vi "BeampointingPerpsectiveDelete.vi"() -> ()   [LabVIEW 2020]
uses:
  Ctrs/beam detection.ctl
  GUI_Beampointing_single_TRA/Ctrs/move.ctl
  Shared/GUI_Template/GUI_master/tcp_new_data_event.ctl
  Shared/GUI_Template/GUI_master/tcp new data cluster.ctl
  Ctrs/thresholds.ctl
  Ctrs/Detection all.ctl
  Ctrs/BP configuration.ctl
  General GUIs/Device GUIs/GUI_Cameras/Controls/Crosshair type def.ctl
  <userlib>/_OpenG.lib/array/array.llb/Filter 1D Array with Scalar (String)__ogtk.vi
  <userlib>/_OpenG.lib/array/array.llb/Sort 1D Array (DBL)__ogtk.vi
  <userlib>/_OpenG.lib/array/array.llb/Reorder 1D Array2 (Variant)__ogtk.vi
  <userlib>/_OpenG.lib/file/file.llb/File Exists - Scalar__ogtk.vi
  <userlib>/_OpenG.lib/array/array.llb/Remove Duplicates from 1D Array (String)__ogtk.vi
  <userlib>/_OpenG.lib/file/file.llb/Strip Path Extension - String__ogtk.vi
  <vilib>/Analysis/NI_AALBase.lvlib
  <vilib>/vision/NI_Vision_Development_Module.lvlib
  <vilib>/Utility/file.llb/Write To Spreadsheet File (string).vi
panel:
  out "Image Dst Out":T1(plugin-control)
  out "12camsproc":string[](array[string])
  out "image::1":T1(plugin-control) caption="CAM-2BL-M4A"
  out "image::2":T1(plugin-control) caption="CAM-2BL-F3M5"
  out "image::3":T1(plugin-control) caption="CAM-2BL-F3M7"
  out "image::4":T1(plugin-control)
  out "image::5":T1(plugin-control)
  out "image::6":T1(plugin-control)
  out "image::7":T1(plugin-control)
  out "image::8":T1(plugin-control)
  out "image::9":T1(plugin-control)
  out "image::10":T1(plugin-control)
  out "image::11":T1(plugin-control)
  out "image::12":T1(plugin-control)
  in  "pixel calib":dbl
  out "A2y":dbl
  out "A1y":dbl
  out "A2x":dbl
  out "A1x":dbl
  in  "y'":dbl
  in  "x'":dbl
  in  "y":dbl
  in  "x":dbl
  in  "distance to target plane":dbl
  in  "seperation":dbl
  in  "downstream mirror":dbl
  in  "upstream mirror":dbl
  in  "Coupled Mirror Move":bool
  out "error out":errorcluster
  in  "active CCDs":i32(listbox)
  out "Prev State":string
  out "tcp data event 2":T2
  out "error out 3":errorcluster
  out "cam means":sgl[](array[numeric])
  in  "save path":path=path "W:/BP_DATA"
  out "millisecond timer value":u32
  out "motor refs 3":refnum<vi>[](array[refnum])
  in  "active man refs":cluster{"Ref X":refnum<vi>, "Ref Y":refnum<vi>}
  in  "#imgs avd so far":dbl
  out "Current State":string
  out "CCDs":string[](array[string])
  in  "GUIdevice 12":string
  in  "GUIdevice 11":string
  in  "GUIdevice 10":string
  in  "GUIdevice 9":string
  out "error out 2":errorcluster
  out "Names":string[](array[string])
  out "Box":T3(array[cluster])
  in  "Tab Cams":T4(tab)=enum."Main"
  in  "Cameras and motors":T5(array[cluster]) {"Motor Alias Y" items=["PlamsaLensHexapod", "IP2 M5 hrz", "IP2 M6 (SFL) hrz", "IP2 M3 (LFL) hrz", "IP2 M5 vrt", "IP2 M6 (SFL) vrt", "IP2 M3 (LFL) vrt", "ch1", "ch2", "ch3", "IP2-M6(vrt)", "IP2-TSZ", "PreplasmaMFA", "Preplasma100mm", "TargetX", "TargetY", "TargetZ", "M1 Y Axis (mm)", "M1 X Axis (mm)", "M2 Y Axis", "M2 X Axis", "M4 Y Axis", "M4 X Axis", "M5 X Axis", "M5 Y Axis", "F3M2 Horizontal", "F3M2 Vertical", "F3M5 Horizontal", "F3M5 Vertical", "F3M6 Horizontal", "F3M3 Vertical", "F3M6 Vertical", "F3M3 Horizontal", "M4A Horizontal", "M4A Vertical", "M2A-horizontal", "M2A-vertical", "Input vertical", "Input horizontal", "Output vertical", "Output horizontal", "HeatM5-X", "HeatM5-Y", "HeatM5-XY", "M1-HPD X position", "broken?", "M1-HPD Y position", "M2-HPD X position", "M2-HPD Y position", "HPDccd2 Stage position", "DMpicoVertical", "DMpicosHorizontal", "Booster horizontal", "Booster vertical", "preamp horizontal", "preamp vertical", "Amp1 out horizontal", "Amp1 out vertical", "Dogleg horizontal", "Dogleg vertical", "DPM-X", "DPM-Y", "DPM-Z", "IP", "PM4-X", "PM4-Y", "SDI_1x", "SDI_1y", "SDI_2x", "SDI_2y", "1BLCompClock", "PilotWavelength", "Compression", "Grating 2&3", "Grating 1&4", "Clocking", "Comp-2BL-separation [mm]", "Comp-2BL-G1G4-angle [degree]", "Comp-2BL-G2G3-angle [degree]", "Comp-2BL-delay [mm]", "HPD2 stage position", "HPD stage position", "AxiconHorizontal", "AxiconVertical"]; "Motor Alias X" items=["PlamsaLensHexapod", "IP2 M5 hrz", "IP2 M6 (SFL) hrz", "IP2 M3 (LFL) hrz", "IP2 M5 vrt", "IP2 M6 (SFL) vrt", "IP2 M3 (LFL) vrt", "ch1", "ch2", "ch3", "IP2-M6(vrt)", "IP2-TSZ", "PreplasmaMFA", "Preplasma100mm", "TargetX", "TargetY", "TargetZ", "M1 Y Axis (mm)", "M1 X Axis (mm)", "M2 Y Axis", "M2 X Axis", "M4 Y Axis", "M4 X Axis", "M5 X Axis", "M5 Y Axis", "F3M2 Horizontal", "F3M2 Vertical", "F3M5 Horizontal", "F3M5 Vertical", "F3M6 Horizontal", "F3M3 Vertical", "F3M6 Vertical", "F3M3 Horizontal", "M4A Horizontal", "M4A Vertical", "M2A-horizontal", "M2A-vertical", "Input vertical", "Input horizontal", "Output vertical", "Output horizontal", "HeatM5-X", "HeatM5-Y", "HeatM5-XY", "M1-HPD X position", "broken?", "M1-HPD Y position", "M2-HPD X position", "M2-HPD Y position", "HPDccd2 Stage position", "DMpicoVertical", "DMpicosHorizontal", "Booster horizontal", "Booster vertical", "preamp horizontal", "preamp vertical", "Amp1 out horizontal", "Amp1 out vertical", "Dogleg horizontal", "Dogleg vertical", "DPM-X", "DPM-Y", "DPM-Z", "IP", "PM4-X", "PM4-Y", "SDI_1x", "SDI_1y", "SDI_2x", "SDI_2y", "1BLCompClock", "PilotWavelength", "Compression", "Grating 2&3", "Grating 1&4", "Clocking", "Comp-2BL-separation [mm]", "Comp-2BL-G1G4-angle [degree]", "Comp-2BL-G2G3-angle [degree]", "Comp-2BL-delay [mm]", "HPD2 stage position", "HPD stage position", "AxiconHorizontal", "AxiconVertical"]}
  in  "tdms root":path=path "c:/BP_DATAsd"
  out "get pos time":u32
  out "config path":string
  out "tolerances (pix)":dbl[](array[numeric])
  in  "device ini":bool
  in  "Exposure:12":dbl=0.095 min=0.0001 max=1.0 format="%#_6f"
  in  "Triggerdelay::12":dbl=0.003 min=0.0 max=0.09 format="%#_6f"
  in  "Exposure::11":dbl=0.095 min=0.0001 max=1.0 format="%#_6f"
  in  "Triggerdelay::11":dbl=0.003 min=0.0 max=0.09 format="%#_6f"
  in  "Exposure::10":dbl=0.095 min=0.0001 max=1.0 format="%#_6f"
  in  "Triggerdelay::10":dbl=0.003 min=0.0 max=0.09 format="%#_6f"
  in  "Exposure::9":dbl=0.095 min=0.0001 max=1.0 format="%#_6f"
  in  "Triggerdelay::9":dbl=0.003 min=0.0 max=0.09 format="%#_6f"
  in  "Trigger::9":bool
  in  "Trigger::10":bool caption="Trigger:10"
  in  "Trigger::11":bool
  in  "Trigger::12":bool
  in  "Target.Y::9":dbl=45.0 caption="T9y" min=0.0 max=2000.0 format="%#_6f"
  in  "Target.X::9":dbl=47.0 caption="Tx9" min=0.0 max=2000.0 format="%#_6f"
  in  "Target.Y::10":dbl=45.0 caption="T10y" min=0.0 max=2000.0 format="%#_6f"
  in  "Target.X::10":dbl=47.0 caption="T10x" min=0.0 max=2000.0 format="%#_6f"
  in  "Target.Y::11":dbl=45.0 caption="T11y" min=0.0 max=2000.0 format="%#_6f"
  in  "Target.X::11":dbl=47.0 caption="T11x" min=0.0 max=2000.0 format="%#_6f"
  in  "Target.Y::12":dbl=45.0 caption="T12y" min=0.0 max=2000.0 format="%#_6f"
  in  "Target.X::12":dbl=47.0 caption="T12x" min=0.0 max=2000.0 format="%#_6f"
  in  "Exposure::8":dbl=0.095 min=3.8e-05 max=1.0 format="%#_6f"
  in  "Triggerdelay::8":dbl=0.003 min=0.0 max=0.09 format="%#_6f"
  in  "Trigger::8":bool
  in  "Target.Y::8":dbl=45.0 caption="T8y" min=0.0 max=2000.0 format="%#_6f"
  in  "Target.X::8":dbl=47.0 caption="T8x" min=0.0 max=2000.0 format="%#_6f"
  in  "Target.Y::7":dbl=45.0 caption="T7x" min=0.0 max=2000.0 format="%#_6f"
  in  "Target.X::7":dbl=47.0 caption="T7y" min=0.0 max=2000.0 format="%#_6f"
  in  "Target.Y::6":dbl=45.0 caption="T6y" min=0.0 max=2000.0 format="%#_6f"
  in  "Target.X::6":dbl=47.0 caption="T6x" min=0.0 max=2000.0 format="%#_6f"
  in  "Target.Y::5":dbl=45.0 caption="T5y" min=0.0 max=2000.0 format="%#_6f"
  in  "Target.X::5":dbl=47.0 caption="T5x" min=0.0 max=2000.0 format="%#_6f"
  in  "Target.Y::4":dbl=45.0 caption="T4y" min=0.0 max=2000.0 format="%#_6f"
  in  "Target.X::4":dbl=47.0 caption="T4x" min=0.0 max=2000.0 format="%#_6f"
  in  "Target.Y::3":dbl=163.0 caption="T3y" min=0.0 max=2000.0 format="%#_6f"
  in  "Target.X::3":dbl=152.0 caption="T3x" min=0.0 max=2000.0 format="%#_6f"
  in  "Target.Y::2":dbl=74.0 caption="T2y" min=0.0 max=2000.0 format="%#_6f"
  in  "Target.X::2":dbl=75.0 caption="T2x" min=0.0 max=2000.0 format="%#_6f"
  in  "Target.Y::1":dbl=61.0 caption="T1y" min=0.0 max=2000.0 format="%#_6f"
  in  "Target.X::1":dbl=77.0 caption="T1x" min=0.0 max=2000.0 format="%#_6f"
  in  "Exposure::7":dbl=0.095 min=3.8e-05 max=1.0 format="%#_6f"
  in  "Triggerdelay::7":dbl=0.003 min=0.0 max=0.09 format="%#_6f"
  in  "Trigger::7":bool
  in  "Exposure::6":dbl=0.095 min=3.8e-05 max=1.0 format="%#_6f"
  in  "Triggerdelay::6":dbl=0.003 min=0.0 max=0.09 format="%#_6f"
  in  "Trigger::6":bool
  in  "Exposure::5":dbl=0.095 min=3.8e-05 max=1.0 format="%#_6f"
  in  "Triggerdelay::5":dbl=0.003 min=0.0 max=0.09 format="%#_6f"
  in  "Trigger::5":bool
  in  "Exposure::4":dbl=0.095 min=3.8e-05 max=10.0 format="%#_6f"
  in  "Triggerdelay::4":dbl=0.003 min=0.0 max=0.09 format="%#_6f"
  in  "Trigger::4":bool
  in  "Exposure::3":dbl=0.095 min=3.8e-05 max=1.0 format="%#_6f"
  in  "Triggerdelay::3":dbl=0.003 min=0.0 max=0.09 format="%#_6f"
  in  "Trigger::3":bool
  in  "Exposure::2":dbl=0.095 min=3.8e-05 max=1.0 format="%#_6f"
  in  "Triggerdelay::2":dbl=0.003 min=0.0 max=0.09 format="%#_6f"
  in  "Trigger::2":bool
  out "Display1":T1(plugin-control) caption="CAM-2BL-M4A"
  out "Display2":T1(plugin-control) caption="CAM-2BL-F3M5"
  out "Display3":T1(plugin-control) caption="CAM-2BL-F3M7"
  out "Display4":T1(plugin-control)
  out "Display5":T1(plugin-control)
  out "Display6":T1(plugin-control)
  out "Display7":T1(plugin-control)
  out "Dsiplay8":T1(plugin-control)
  in  "Exposure::1":dbl=0.095 min=3.8e-05 max=10.0 format="%#_6f"
  in  "Triggerdelay::1":dbl=0.003 min=0.0 max=0.09 format="%#_6f"
  in  "Trigger::1":bool
  in  "UDP error message":string
  out "required Y":bool[](array[boolean])
  out "required X":bool[](array[boolean])
  out "detected":bool[](array[boolean])
  out "name array":string[](array[string])
  out "Display9":T1(plugin-control)
  out "Display10":T1(plugin-control)
  out "Display11":T1(plugin-control)
  out "Display12":T1(plugin-control)
  out "CCD 1":cluster{timestamp[], dbl[]}[](graph)
  in  "History Size":i32=500
  out "History Index":i32
  in  "Cam# history":i32
  out "Moving X":string
  out "Moving Y":string
  in  "centroidy::4":dbl=45.0 caption="T4y" min=0.0 max=0.0 format="%#_6f"
  in  "centroidx::4":dbl=47.0 caption="T4x" min=0.0 max=0.0 format="%#_6f"
  in  "centroidy::3":dbl=163.0 caption="T3y" min=0.0 max=0.0 format="%#_6f"
  in  "centroidx::3":dbl=152.0 caption="T3x" min=0.0 max=0.0 format="%#_6f"
  in  "centroidy::2":dbl=74.0 caption="T2y" min=0.0 max=0.0 format="%#_6f"
  in  "centroidx::2":dbl=75.0 caption="T2x" min=0.0 max=0.0 format="%#_6f"
  in  "centroidy::1":dbl=61.0 caption="T1y" min=0.0 max=0.0 format="%#_6f"
  in  "centroidx::1":dbl=77.0 caption="T1x" min=0.0 max=0.0 format="%#_6f"
  in  "centroidy::8":dbl=45.0 caption="T8y" min=0.0 max=0.0 format="%#_6f"
  in  "centroidx::8":dbl=47.0 caption="T8x" min=0.0 max=0.0 format="%#_6f"
  in  "centroidy::7":dbl=45.0 caption="T7x" min=0.0 max=0.0 format="%#_6f"
  in  "centroidx::7":dbl=47.0 caption="T7y" min=0.0 max=0.0 format="%#_6f"
  in  "centroidy::6":dbl=45.0 caption="T6y" min=0.0 max=0.0 format="%#_6f"
  in  "centroidx::6":dbl=47.0 caption="T6x" min=0.0 max=0.0 format="%#_6f"
  in  "centroidy::5":dbl=45.0 caption="T5y" min=0.0 max=0.0 format="%#_6f"
  in  "centroidx::5":dbl=47.0 caption="T5x" min=0.0 max=0.0 format="%#_6f"
  in  "centroidy::12":dbl=45.0 caption="T12y" min=0.0 max=2000.0 format="%#_6f"
  in  "centroidx::12":dbl=47.0 caption="T12x" min=0.0 max=2000.0 format="%#_6f"
  in  "centroidy::11":dbl=45.0 caption="T11y" min=0.0 max=2000.0 format="%#_6f"
  in  "centroidx::11":dbl=47.0 caption="T11x" min=0.0 max=2000.0 format="%#_6f"
  in  "centroidy::10":dbl=45.0 caption="T10y" min=0.0 max=2000.0 format="%#_6f"
  in  "centroidx::10":dbl=47.0 caption="T10x" min=0.0 max=2000.0 format="%#_6f"
  in  "centroidy::9":dbl=45.0 caption="T9y" min=0.0 max=2000.0 format="%#_6f"
  in  "centroidx::9":dbl=47.0 caption="Tx9" min=0.0 max=2000.0 format="%#_6f"
  out "active ccd particles":T6(array[cluster])
  in  "Speedmode":dbl=5.0 min=1.0 max=20.0
  out "all UDP in motor config good":bool
  in  "PerspectiveCorrectGUI::1":bool caption="Perpsective1"
  in  "PerspectivePath::1":string
  in  "PerspectivePath::2":string caption="PerspectivePath::1"
  in  "PerspectiveCorrectGUI::2":bool caption="Perpsective1"
  in  "PerspectivePath::3":string caption="PerspectivePath::1"
  in  "PerspectiveCorrectGUI::3":bool caption="Perpsective1"
  in  "PerspectivePath::4":string caption="PerspectivePath::1"
  in  "PerspectiveCorrectGUI::4":bool caption="Perpsective1"
  in  "PerspectivePath::5":string caption="PerspectivePath::1"
  in  "PerspectiveCorrectGUI::5":bool caption="Perpsective1"
  in  "PerspectivePath::6":string caption="PerspectivePath::1"
  in  "PerspectiveCorrectGUI::6":bool caption="Perpsective1"
  in  "Feedback Global":bool
  in  "GUIdevice 8":string
  in  "Tab Control":T7(tab)
  in  "alarms":bool
  in  "new tdms":bool
  in  "Save Stats":bool
  in  "Save Config":bool
  in  "Load Config":bool
  in  "update speed [ms]":i32=2000 min=1000 max=10000
  in  "img to avg":i32=15 min=3 max=200
  in  "Reset History":bool
  in  "autodetect":bool
  in  "Detection Rate":dbl=0.9 min=0.001 max=1.0
  in  "Center":bool
  in  "Align":bool
  in  "average centroid":bool
  in  "clear error":bool
  in  "thresholds":T8
  in  "beam detection para":T9={"Filter"=1, "Filter Para"={"X Size"=5, "Y Size"=5, "% Tolerance"=1}, "detection method"=4, "Particle filtering"=[{"Measurement Parameter"=35, "Range Lower Value"=0.0, "Range Upper Value"=500.0, "Range"=FALSE, "Measurement Type"=FALSE}], "Remove small Objects"=TRUE, "Restrict to round Objects"=FALSE, "Use Cam COM"=FALSE} {"Particle filtering"."Measurement Parameter" items=["Center of Mass X", "Center of Mass Y", "First Pixel X", "First Pixel Y", "Bounding Rect Left", "Bounding Rect Top", "Bounding Rect Right", "Bounding Rect Bottom", "Max Feret Diameter Start X", "Max Feret Diameter Start Y", "Max Feret Diameter End X", "Max Feret Diameter End Y", "Max Horiz. Segment Length Left", "Max Horiz. Segment Length Right", "Max Horiz. Segment Length Row", "-", "Bounding Rect Width", "Bounding Rect Height", "Bounding Rect Diagonal", "Perimeter", "Convex Hull Perimeter", "Holes' Perimeter", "Max Feret Diameter", "Equivalent Ellipse Major Axis", "Equivalent Ellipse Minor Axis", "Equivalent Ellipse Minor Axis (Feret)", "Equivalent Rect Long Side", "Equivalent Rect Short Side", "Equivalent Rect Diagonal", "Equivalent Rect Short Side (Feret)", "Average Horiz. Segment Length", "Average Vert. Segment Length", "Hydraulic Radius", "Waddel Disk Diameter", "-", "Area", "Holes' Area", "Particle & Holes' Area", "Convex Hull Area", "Image Area", "-", "Number of Holes", "Number of Horiz. Segments", "Number of Vert. Segments", "-", "Orientation", "Max Feret Diameter Orientation", "-", "% Area/Image Area", "% Area/(Particle & Holes' Area)", "Ratio of Equivalent Ellipse Axes", "Ratio of Equivalent Rect Sides", "-", "Elongation Factor", "Compactness Factor", "Heywood Circularity Factor", "Type Factor", "-", "Sum X", "Sum Y", "Sum XX", "Sum XY", "Sum YY", "Sum XXX", "Sum XXY", "Sum XYY", "Sum YYY", "-", "Moment of Inertia XX", "Moment of Inertia XY", "Moment of Inertia YY", "Moment of Inertia XXX", "Moment of Inertia XXY", "Moment of Inertia XYY", "Moment of Inertia YYY", "Norm. Moment of Inertia XX", "Norm. Moment of Inertia XY", "Norm. Moment of Inertia YY", "Norm. Moment of Inertia XXX", "Norm. Moment of Inertia XXY", "Norm. Moment of Inertia XYY", "Norm. Moment of Inertia YYY", "Hu Moment 1", "Hu Moment 2", "Hu Moment 3", "Hu Moment 4", "Hu Moment 5", "Hu Moment 6", "Hu Moment 7"]; "Particle filtering"."Range Lower Value" format="%.2f"; "Particle filtering"."Range Upper Value" format="%.2f"; "detection method" items=["clustering", "entropy", "metric", "moments", "inter-class variance"]; "Filter" items=["No Filter", "Median Filter", "Low Pass Filter"]}
  out "Active CCD":string
  in  "move config":T11={"Tolerance [%]"=0.1, "Stepsize"=0.0001, "Invert Direction X"=FALSE, "Invert Direction Y"=TRUE, "enable feedback"=FALSE, "Set Centriod Target"=FALSE, "xCal"=0.0001, "xCal neg"=0.0001, "yCal"=0.0001, "yCal neg"=0.0001}
  in  "Position 2":dbl=0.001 caption="Stepsize" min=0.0 max=999999.0 format="%_6f"
  in  "Position 1":dbl=0.001 caption="Stepsize" min=0.0 max=999999.0 format="%_6f"
  in  "Right":bool caption="RelativeMove.Axis 1.CCW::1"
  in  "Left":bool caption="RelativeMove.Axis 1.CW::1"
  in  "Down":bool caption="RelativeMove.Axis. 2.CCW::1"
  in  "Up":bool caption="RelativeMove.Axis 2.CW::1"
  in  "StepSize":dbl=0.01 caption="Stepsize" min=0.0 max=1.0 step=0.001 format="%#_6p"
  in  "Time":timestamp[][](array[timestamp])
  in  "Offset X":dbl[][](array[numeric])
  in  "Mean Centroid X":dbl[][](array[numeric])
  in  "GUIdevice 7":string
  in  "GUIdevice 6":string
  in  "GUIdevice 5":string
  in  "GUIdevice 4":string
  in  "GUIdevice 3":string="TargetCam10Hz_Diode"
  in  "GUIdevice 2":string="StagingM1Far"
  in  "insert tag":bool=TRUE
  in  "stop":bool
  in  "GUIdevice 1":string="StagingM1Near"
  out "error IO 2":errorcluster
  # "code in progess for coupled mirror move: please don't delete (Sam)"
  # "Motor axes must have aliases"
  # "Save config after changing cams/motors"
  # "max"
  # "When running for the first time\nCancel the load configuration\nSet the Camera and motors in the config tab\nSave the configuration\nLoad the configuration\nConfigure the detection and feedback for each camera\nSave the configuration\n\nTips\nIn detection, you can exclude or include particles. Typically, include based on the area of the particle.\nYou can either use the particle centroid, or the center of mass calculated in the camera\nFor the case of camera COM, it will only use it if it is in the bounding box of the detected particle.\nA calibration is critical for good performance. Use MC to perform a motor scan and perform a linear fit of COM vs motor position in x and y. Put the gradients into xCal and yCal.\nStep size in move config no longer used.\nFor motors (like LTAs), set the backlash and set it to default in MC. Backlash amount is retrieved from a positive and negative motor scan, and reading the position distance between the lines of the graph of COM vs motor position.\nUnder system tab, update speed must be > than slowest camera update. Otherwise program will find the slow cam/s not having a new image, and it will perform a new configuration."
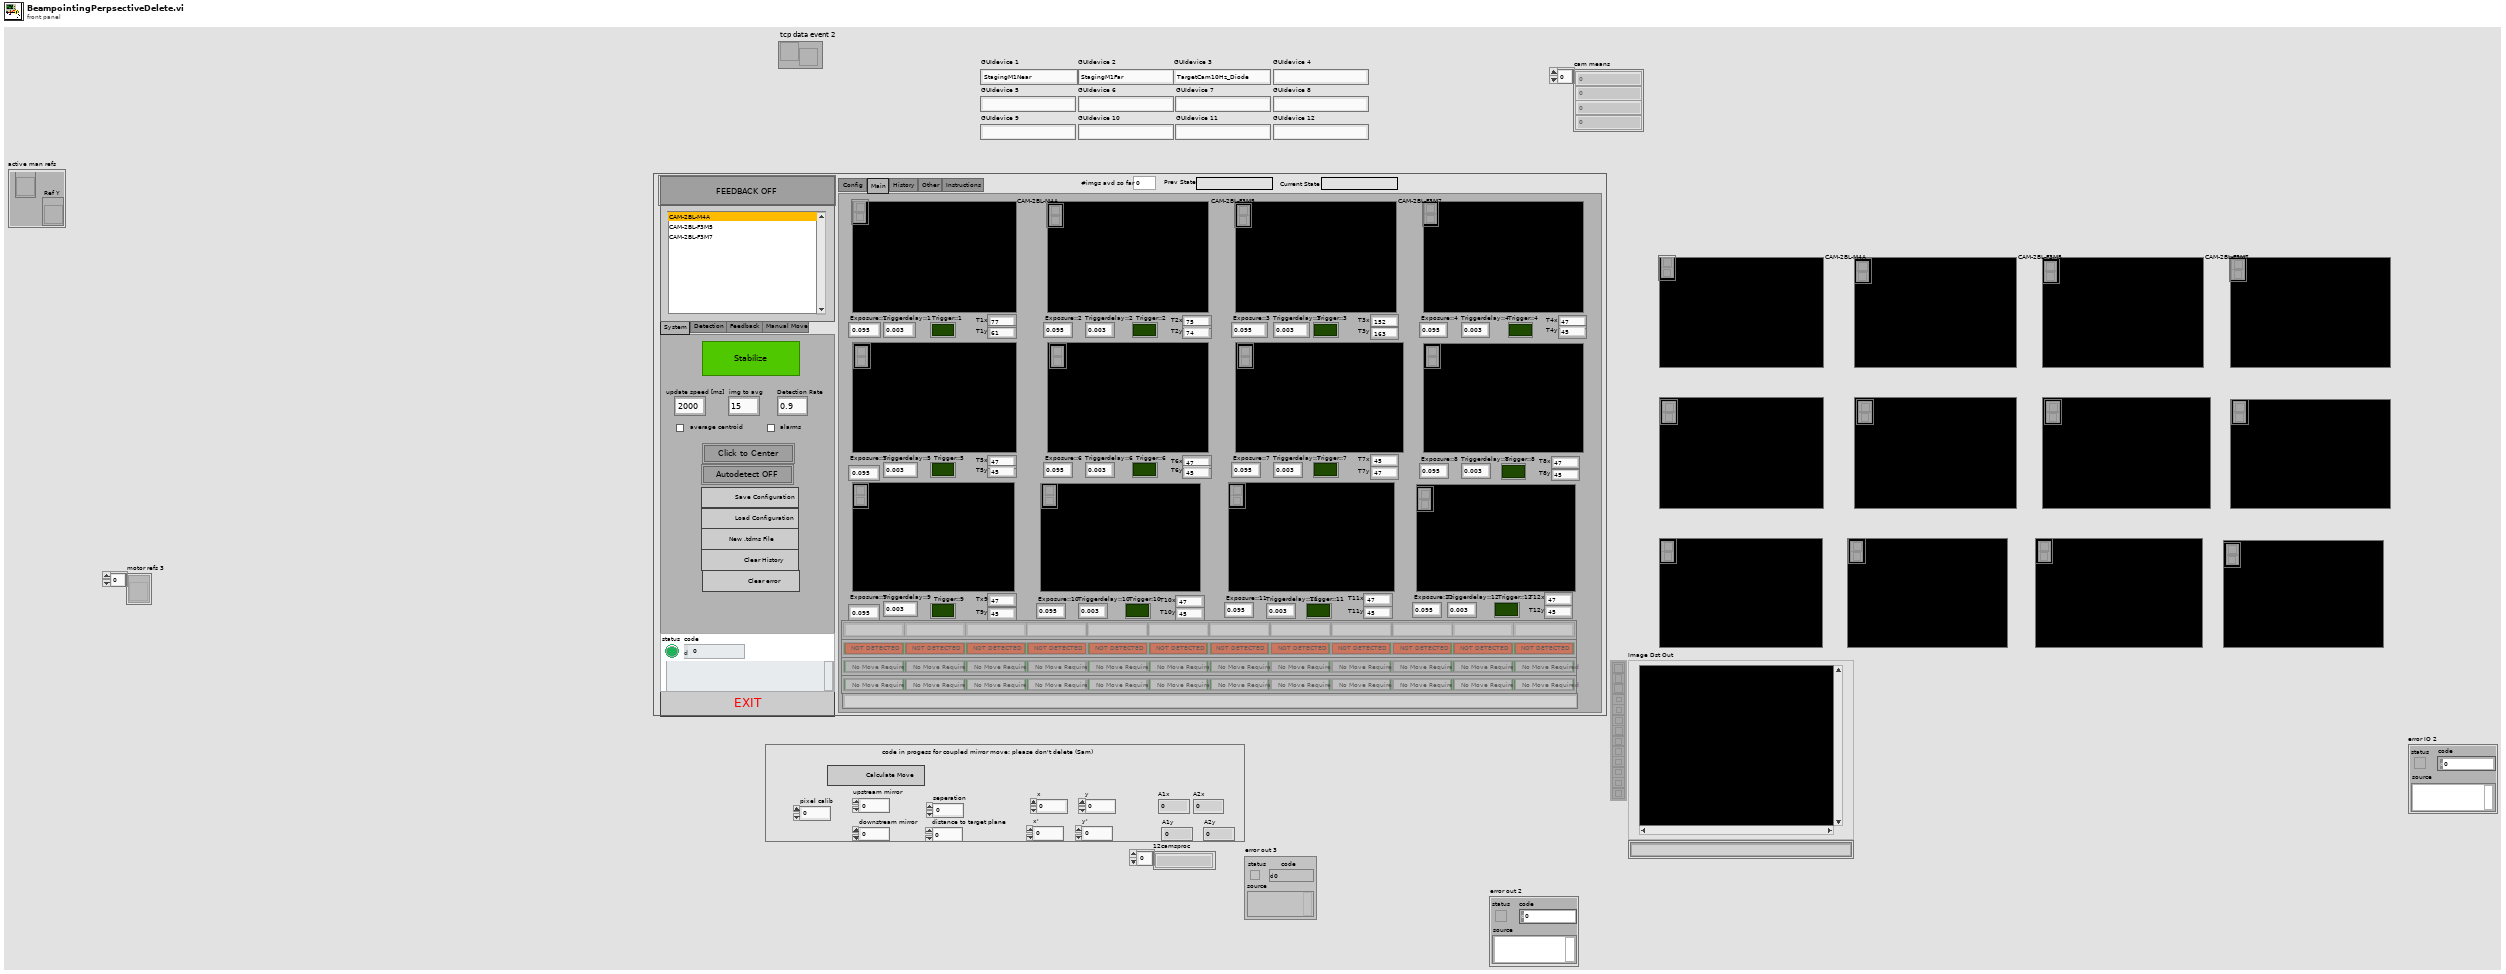
[diagram p1: front panel]
types:
  T1 = typedef "IMAQ Image.ctl" = refnum<image>
  T2 = typedef "tcp_new_data_event.ctl" = refnum<user-event>
  T3 = cluster{"Left":dbl, "Top":dbl, "Right":dbl, "Bottom":dbl}[]
  T4 = enum32{"Config ", "Main", "History", "Other", "Instructions"}
  T5 = cluster{"Camera":string, "Motor Alias X":u16, "Motor Alias Y":u16}[]
  T6 = cluster{"Area":dbl, "Number of Holes":dbl, "Bounding Rect":cluster{"Left":dbl, "Top":dbl, "Right":dbl, "Bottom":dbl}, "Center of Mass":cluster{"X":dbl, "Y":dbl}, "Orientation":dbl, "Dimensions":cluster{"Width":dbl, "Height":dbl}}[]
  T7 = enum32{"System", "Detection", "Feedback", "Manual Move"}
  T8 = typedef "thresholds.ctl" = cluster{"Lower value":sgl, "Upper value":sgl}
  T9 = typedef "beam detection.ctl" = cluster{"Filter":u16, "Filter Para":cluster{"X Size":i32, "Y Size":i32, "% Tolerance":i32}, "detection method":i32, "Particle filtering":cluster{"Measurement Parameter":T10, "Range Lower Value":dbl, "Range Upper Value":dbl, "Range":bool, "Measurement Type":bool}[], "Remove small Objects":bool, "Restrict to round Objects":bool, "Use Cam COM":bool}
  T10 = typedef "Particle Parameters" = i32
  T11 = typedef "move.ctl" = cluster{"Tolerance [%]":dbl, "Stepsize":dbl, "Invert Direction X":bool, "Invert Direction Y":bool, "enable feedback":bool, "Set Centriod Target":bool, "xCal":dbl, "xCal neg":dbl, "yCal":dbl, "yCal neg":dbl}
  T12 = cluster{"Target.X::1":refnum<vi>, "Target.Y::1":refnum<vi>}
  T13 = cluster{"Target.X::2":refnum<vi>, "Target.Y::2":refnum<vi>}
  T14 = cluster{"Target.X::3":refnum<vi>, "Target.Y::3":refnum<vi>}
  T15 = cluster{"Target.X::4":refnum<vi>, "Target.Y::4":refnum<vi>}
  T16 = cluster{"Target.X::5":refnum<vi>, "Target.Y::5":refnum<vi>}
  T17 = cluster{"Target.X::6":refnum<vi>, "Target.Y::6":refnum<vi>}
  T18 = cluster{"Target.X::7":refnum<vi>, "Target.Y::7":refnum<vi>}
  T19 = cluster{"Target.X::8":refnum<vi>, "Target.Y::8":refnum<vi>}
  T20 = cluster{"Target.X::12":refnum<vi>, "Target.Y::12":refnum<vi>}
  T21 = cluster{"Target.X::9":refnum<vi>, "Target.Y::9":refnum<vi>}
  T22 = cluster{"Target.X::10":refnum<vi>, "Target.Y::10":refnum<vi>}
  T23 = cluster{"Target.X::11":refnum<vi>, "Target.Y::11":refnum<vi>}
  T24 = cluster{"Target.X::12":refnum<vi>, "Target.Y::12":refnum<vi>}[]
  T25 = enum32{"invalid app kind", "Development System", "Run Time System", "Student Edition", "Embedded LabVIEW", "Evaluation", "Custom"}
  T26 = enum32{"Invalid", "Standard", "Closed", "Hidden", "Minimized", "Maximized"}
  T27 = typedef "BP configuration.ctl" = cluster{"Camera names":string[], "Motor aliases x":string[], "Motor aliases y":string[], "detection para":T9[], "thresholds":cluster{"Lower value":sgl, "Upper value":sgl}[], "move properties":T11[], "tdms root":path}
  T28 = typedef "tcp new data cluster.ctl" = cluster{"EventEnum":enum16{"new data", "connection status update"}, "Device name":string}
  T29 = enum16{"open", "replace", "create", "open or create", "replace or create", "replace or create with confirmation"}
  T30 = enum8{"Enabled", "Disabled", "Disabled and Grayed Out"}
  T31 = enum16{"open", "open or create", "create or replace", "create", "open (read-only)"}
  T32 = typedef "Detection all.ctl" = cluster{"detection para":T9[], "thresholds":cluster{"Lower value":sgl, "Upper value":sgl}[], "Centroid X":dbl[][], "Centroid Y":dbl[][], "Size":dbl[][], "Centroid refs":cluster{"centroidx::12":refnum<vi>, "centroidy::12":refnum<vi>}[], "img to avg":i32}
  T33 = cluster{"detection para":T9[], "thresholds":cluster{"Lower value":sgl, "Upper value":sgl}[], "Centroid X":dbl[][], "Centroid Y":dbl[][], "Size":dbl[][], "Centroid refs":cluster{"centroidx::12":refnum<vi>, "centroidy::12":refnum<vi>}[], "img to avg":i32}
  T34 = cluster{"Area":dbl, "Number of Holes":dbl, "Bounding Rect":cluster{"Left":dbl, "Top":dbl, "Right":dbl, "Bottom":dbl}, "Center of Mass":cluster{"X":dbl, "Y":dbl}, "Orientation":dbl, "Dimensions":cluster{"Width":dbl, "Height":dbl}}[][]
  T35 = cluster{"Core":cluster{"Current VI Reference":refnum<vi>, "Close Panel on Exit?":bool}, "Detection":T32, "Mean Centroid X":dbl[][], "Mean Centroid Y":dbl[][], "Offset X":dbl[][], "Offset Y":dbl[][], "Offset X stats ":dbl[][], "Offset Y stats ":dbl[][], "Mean Size":dbl[][], "Time":timestamp[][], "move properties":T11[], "active axis refs 2":cluster{"Ref X":refnum<vi>, "Ref Y":refnum<vi>}[], "active ccd":i32, "Feedback global":bool, "Motor X":dbl[][], "Motor Y":dbl[][], "active cams":string[], "tdms ref":refnum<k34>, "active man refs":cluster{"Ref X":refnum<vi>, "Ref Y":refnum<vi>}, "detected":bool[], "speedmode X":bool[], "speedmode Y":bool[], "steps speed X":dbl[], "steps speed Y":dbl[], "Supergui":cluster{"STOP queue":refnum<queue>, "SuperGUI ref":refnum<vi>}, "dev var alias arrays":cluster{"dev variable alias":string[][], "dev variable alias Motors X":string[][], "dev variable alias Motors Y":string[][]}, "Motor positions":cluster{"Positions x":dbl[], "Positions y":dbl[]}, "Config loaded":bool}
  T36 = cluster{"Positions x":dbl[], "Positions y":dbl[]}
  T37 = cluster{"dev variable alias":string[][], "dev variable alias Motors X":string[][], "dev variable alias Motors Y":string[][]}
  T38 = cluster{"Ref X":refnum<vi>, "Ref Y":refnum<vi>}[]
  T39 = cluster{"STOP queue":refnum<queue>, "SuperGUI ref":refnum<vi>}
  T40 = cluster{"Current VI Reference":refnum<vi>, "Close Panel on Exit?":bool}
  T41 = cluster{"centroidx::1":refnum<vi>, "centroidy::1":refnum<vi>}
  T42 = cluster{"centroidx::2":refnum<vi>, "centroidy::2":refnum<vi>}
  T43 = cluster{"centroidx::3":refnum<vi>, "centroidy::3":refnum<vi>}
  T44 = cluster{"centroidx::4":refnum<vi>, "centroidy::4":refnum<vi>}
  T45 = cluster{"centroidx::5":refnum<vi>, "centroidy::5":refnum<vi>}
  T46 = cluster{"centroidx::6":refnum<vi>, "centroidy::6":refnum<vi>}
  T47 = cluster{"centroidx::7":refnum<vi>, "centroidy::7":refnum<vi>}
  T48 = cluster{"centroidx::8":refnum<vi>, "centroidy::8":refnum<vi>}
  T49 = cluster{"centroidx::12":refnum<vi>, "centroidy::12":refnum<vi>}
  T50 = cluster{"centroidx::9":refnum<vi>, "centroidy::9":refnum<vi>}
  T51 = cluster{"centroidx::10":refnum<vi>, "centroidy::10":refnum<vi>}
  T52 = cluster{"centroidx::11":refnum<vi>, "centroidy::11":refnum<vi>}
  T53 = cluster{"centroidx::12":refnum<vi>, "centroidy::12":refnum<vi>}[]
  T54 = cluster{"Camera":string, "Motor Alias X":u16, "Motor Alias Y":u16}
  T55 = typedef "Image Type" = u32
  T56 = cluster{"appended array":timestamp[], "appended array":dbl[]}
  T57 = cluster{"appended array":timestamp[], "appended array":dbl[]}[]
  T58 = typedef "Crosshair type def.ctl" = cluster{"Draw":bool, "Target":cluster{"x":dbl, "y":dbl}, "Size":cluster{"x":dbl, "y":dbl}, "Angle":dbl, "Color":u32, "Thickness":u8, "CrosshairLabel":string}
  T59 = cluster{"Left":i32, "Top":i32, "Right":i32, "Bottom":i32}
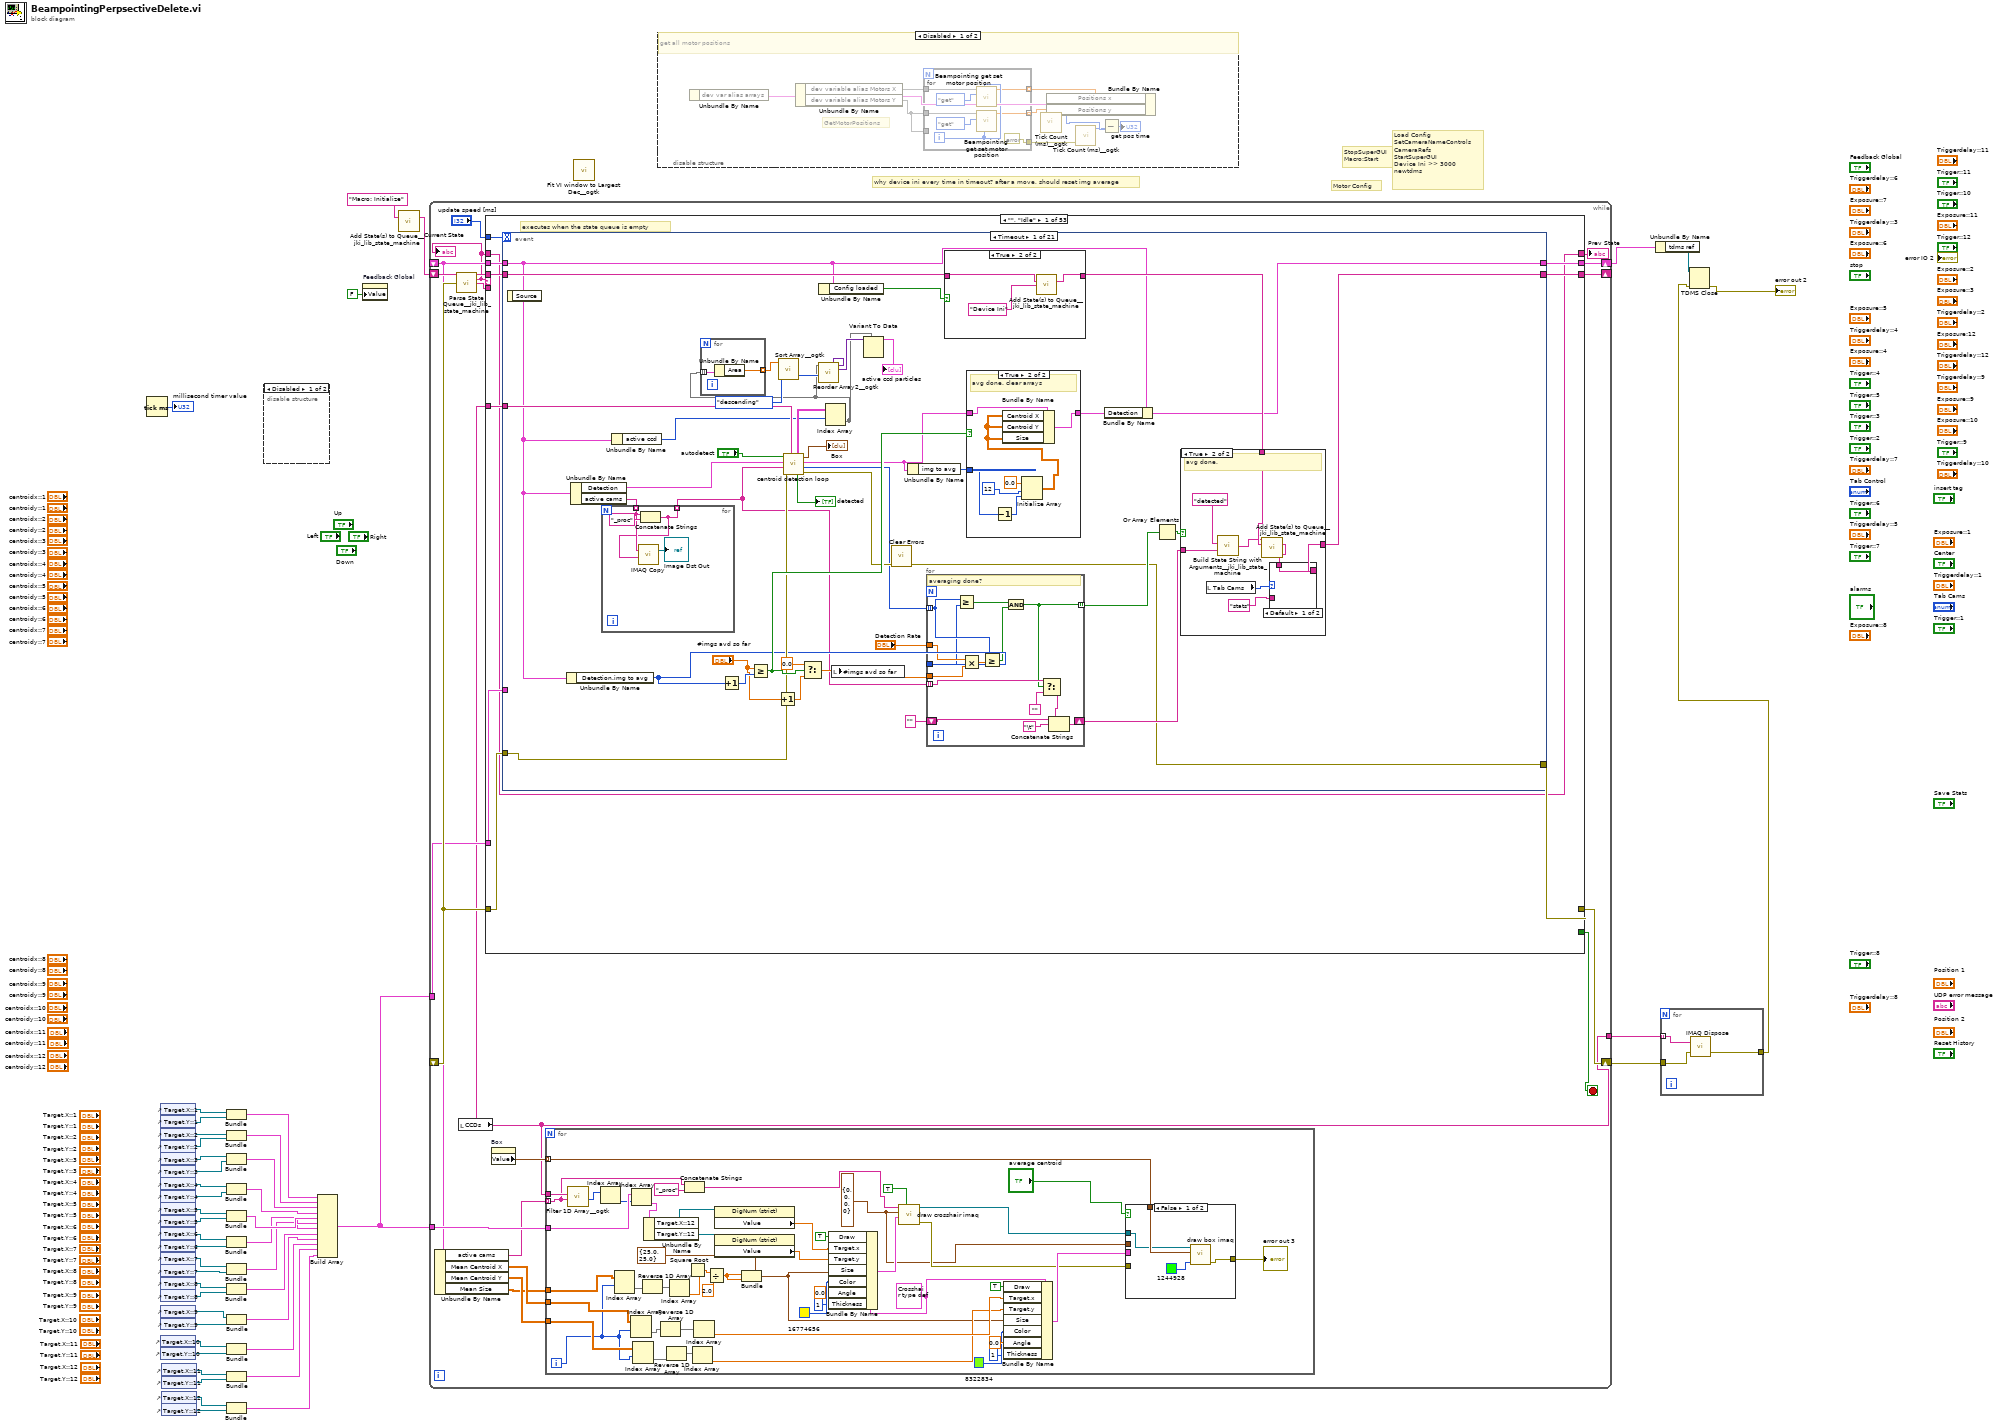
[diagram p0: block diagram]
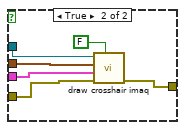
[diagram p4: hidden frame]
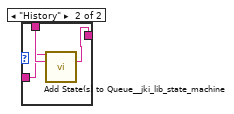
[diagram p8: hidden frame]
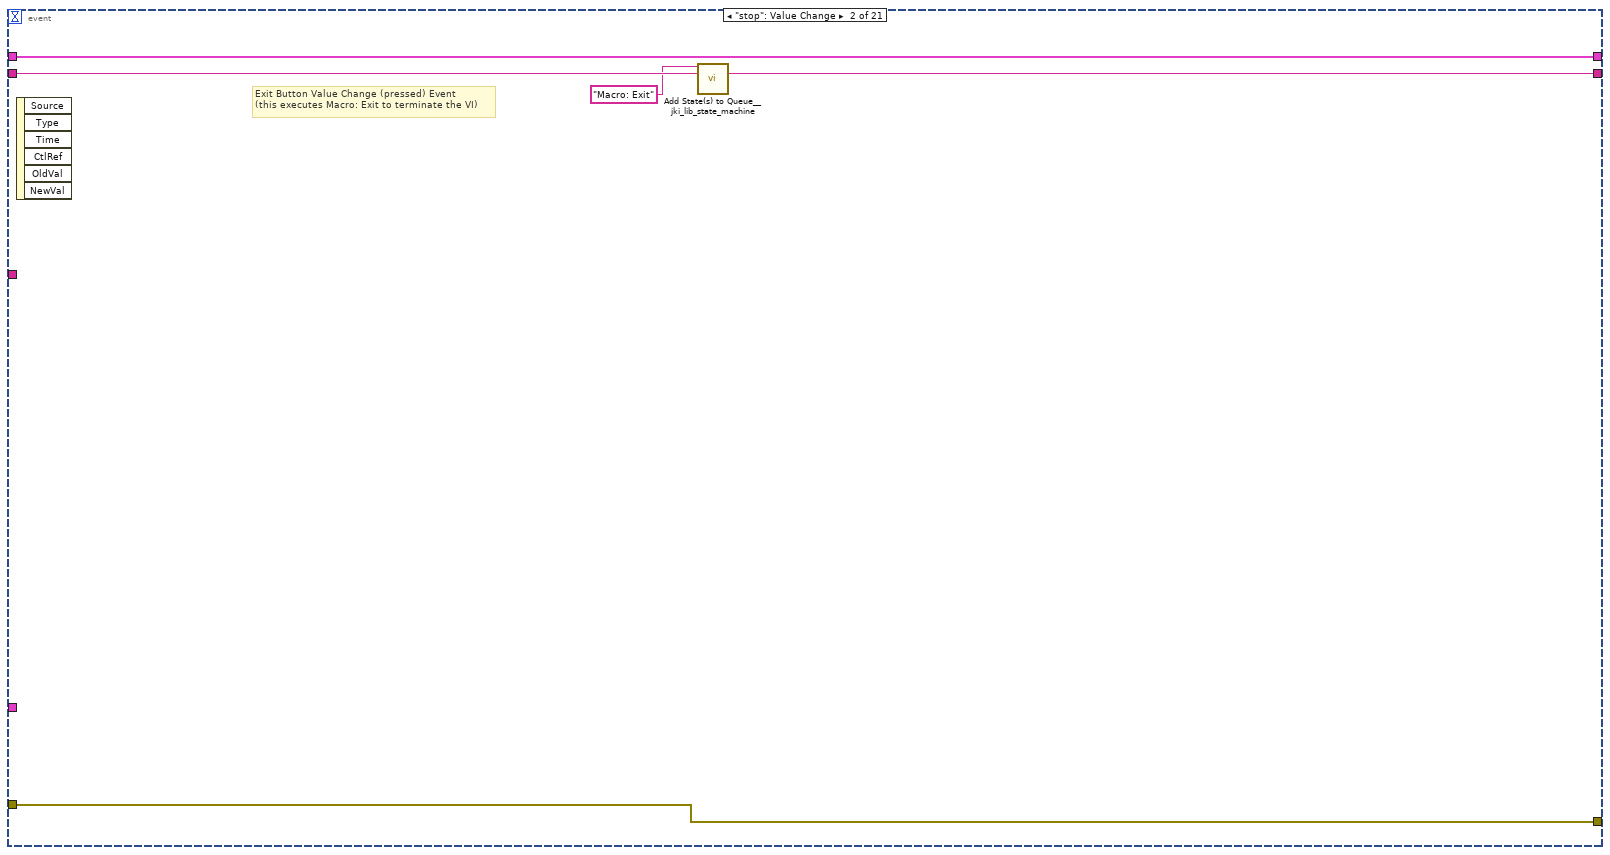
[diagram p9: hidden frame]
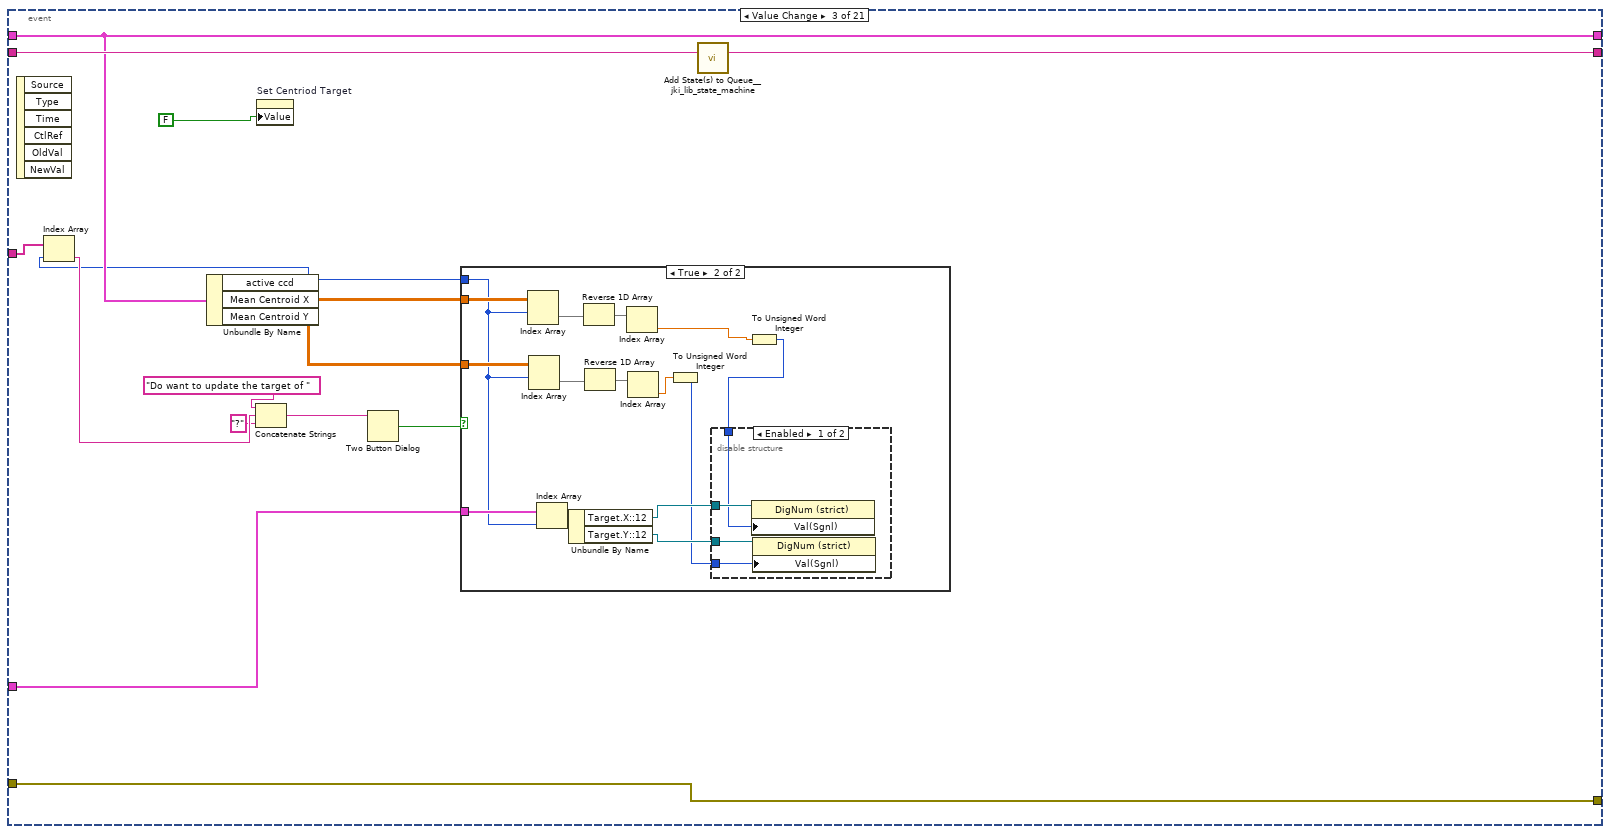
[diagram p10: hidden frame]
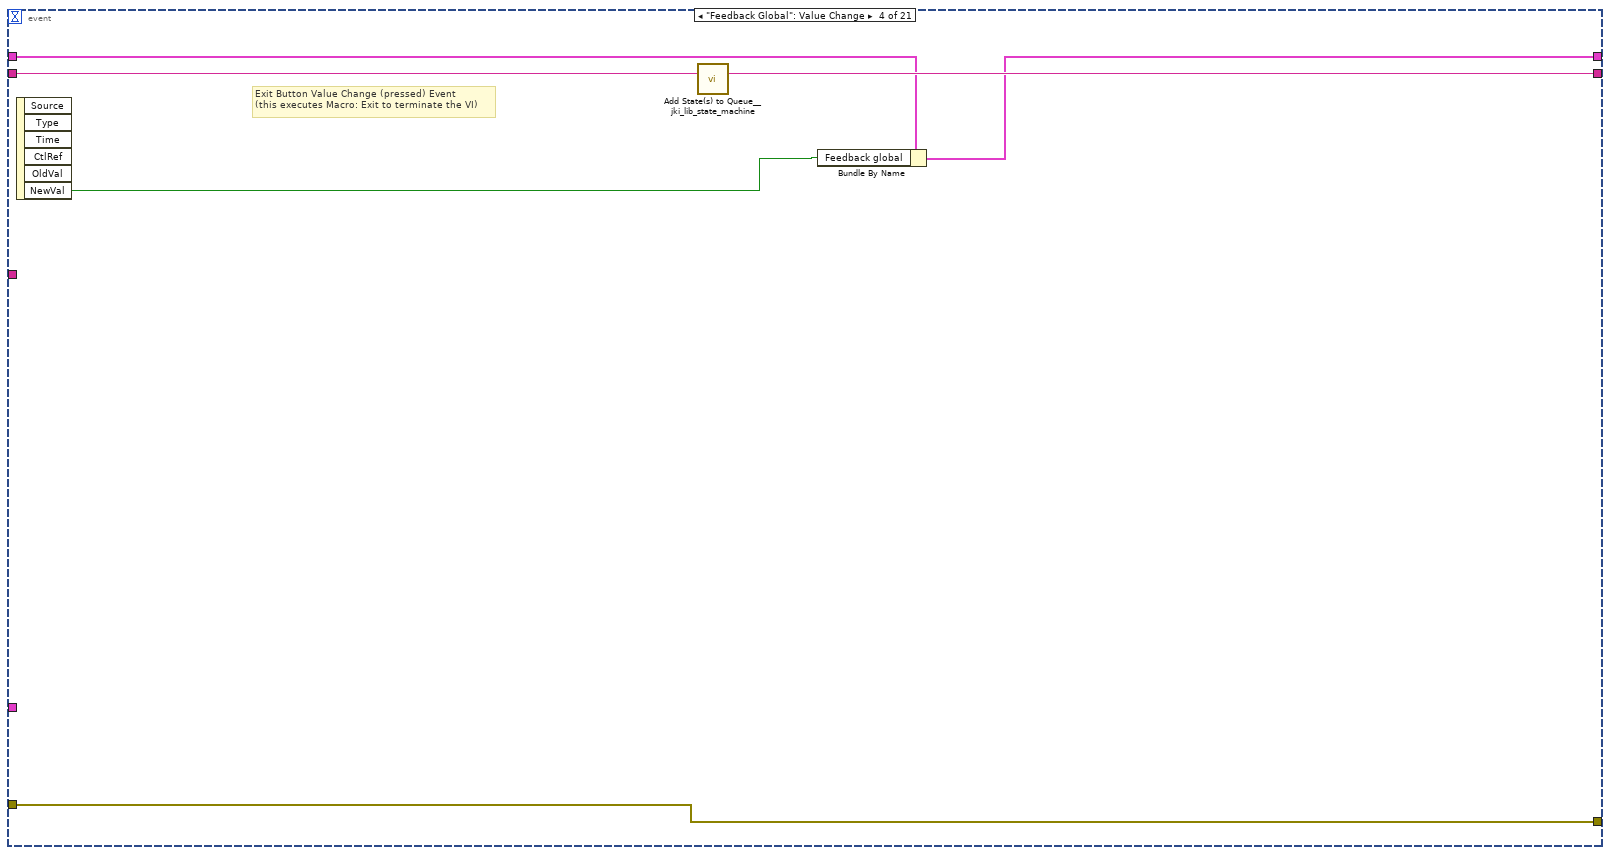
[diagram p13: hidden frame]
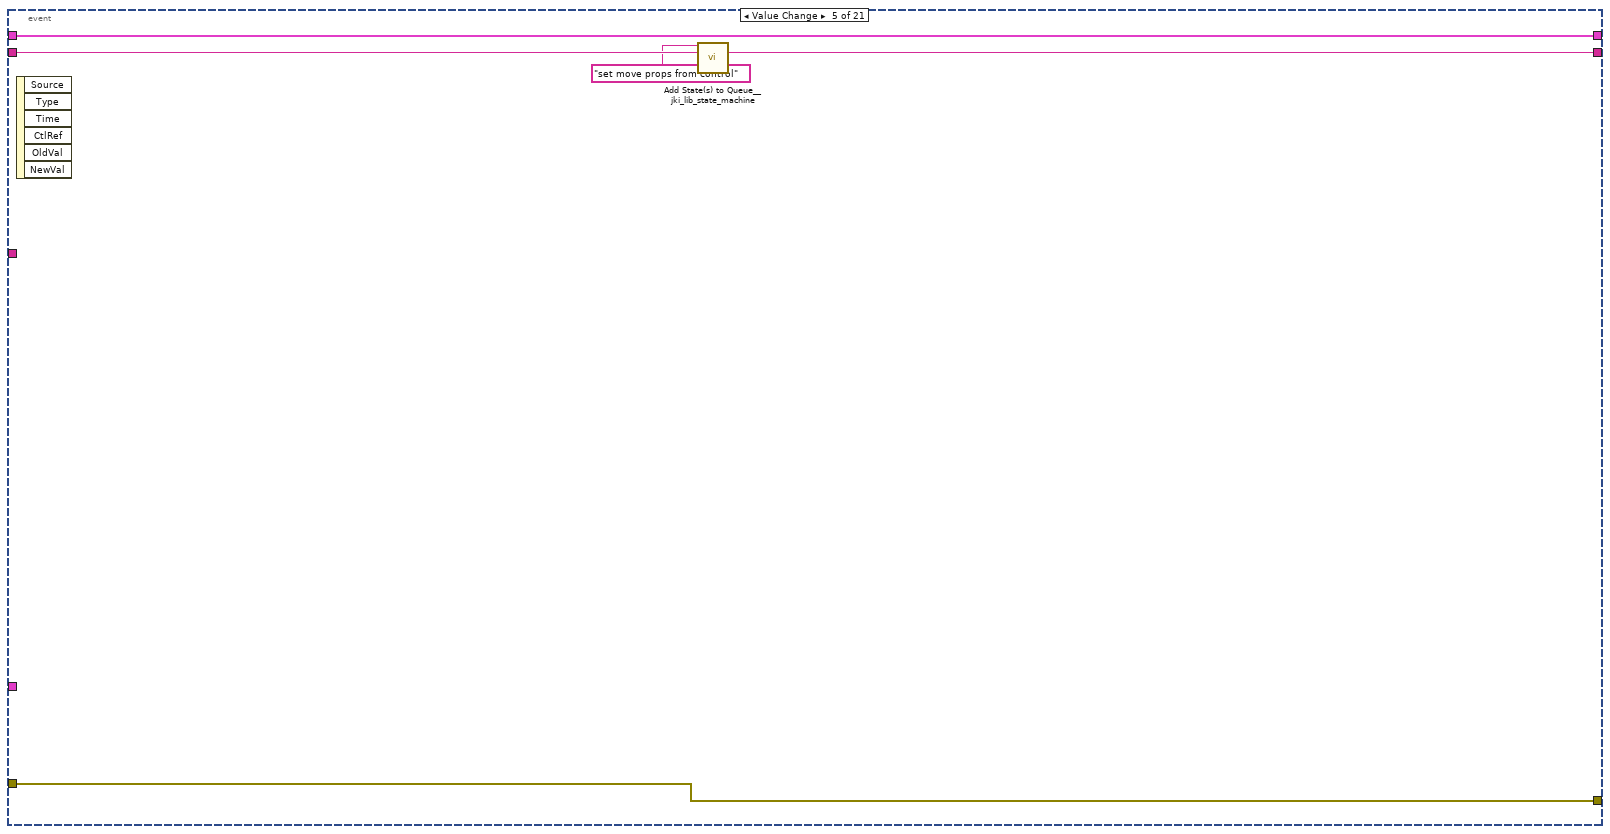
[diagram p14: hidden frame]
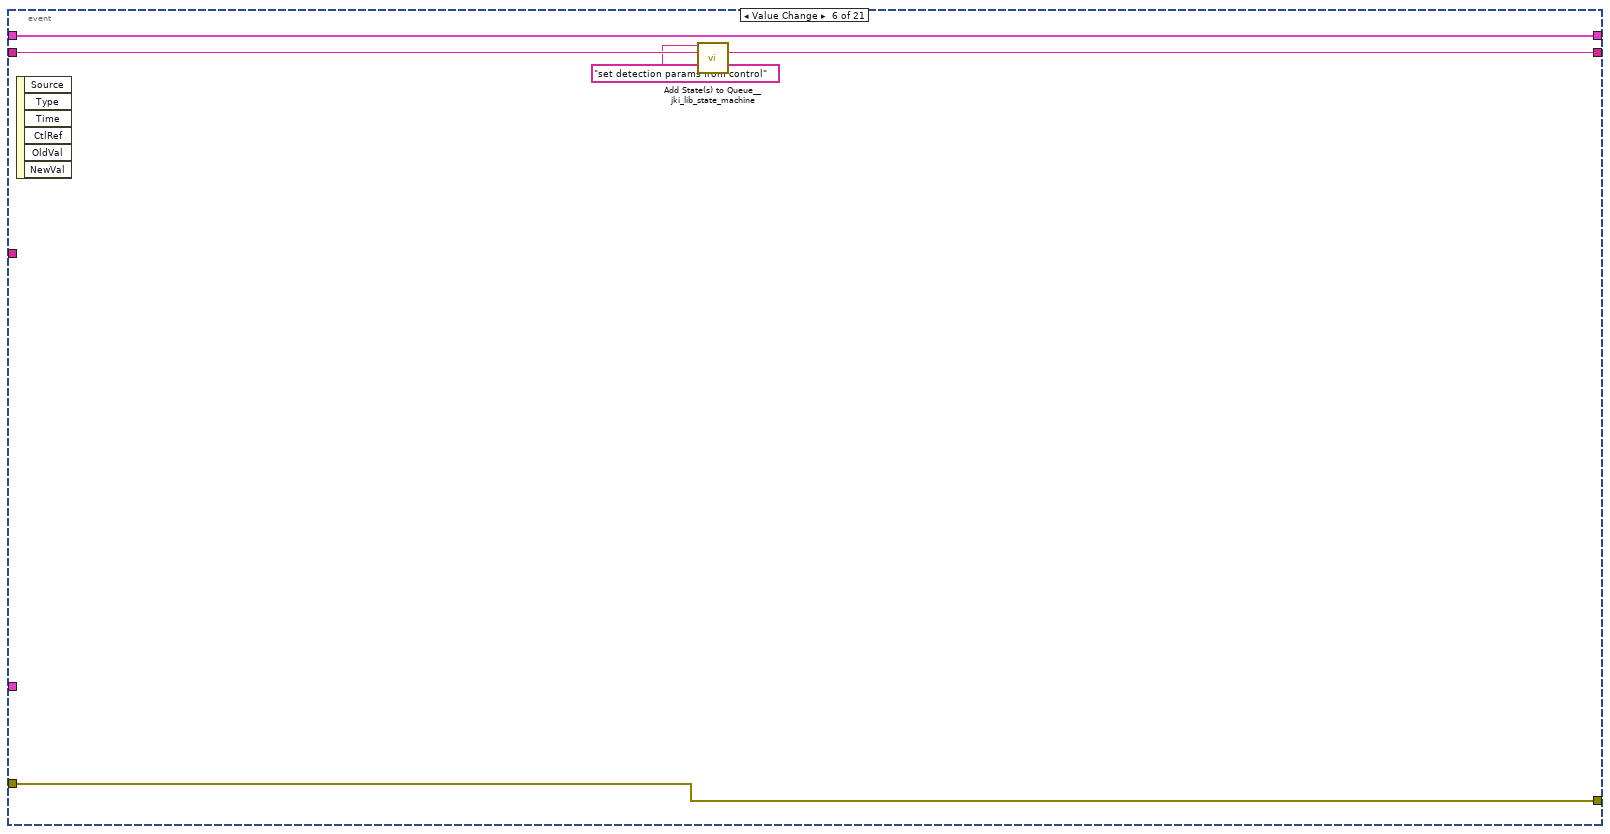
[diagram p15: hidden frame]
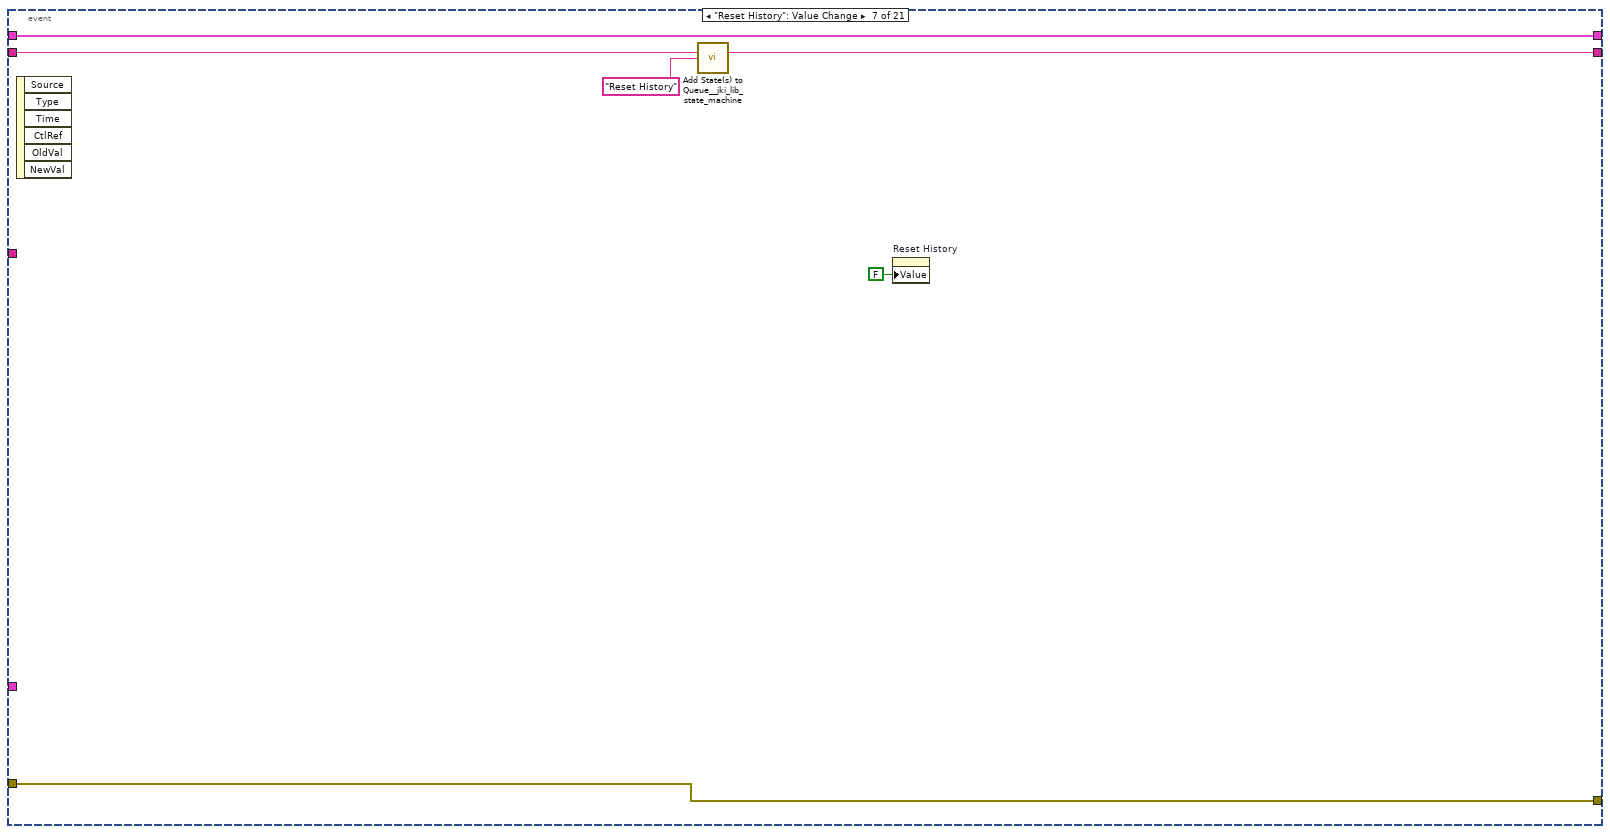
[diagram p16: hidden frame]
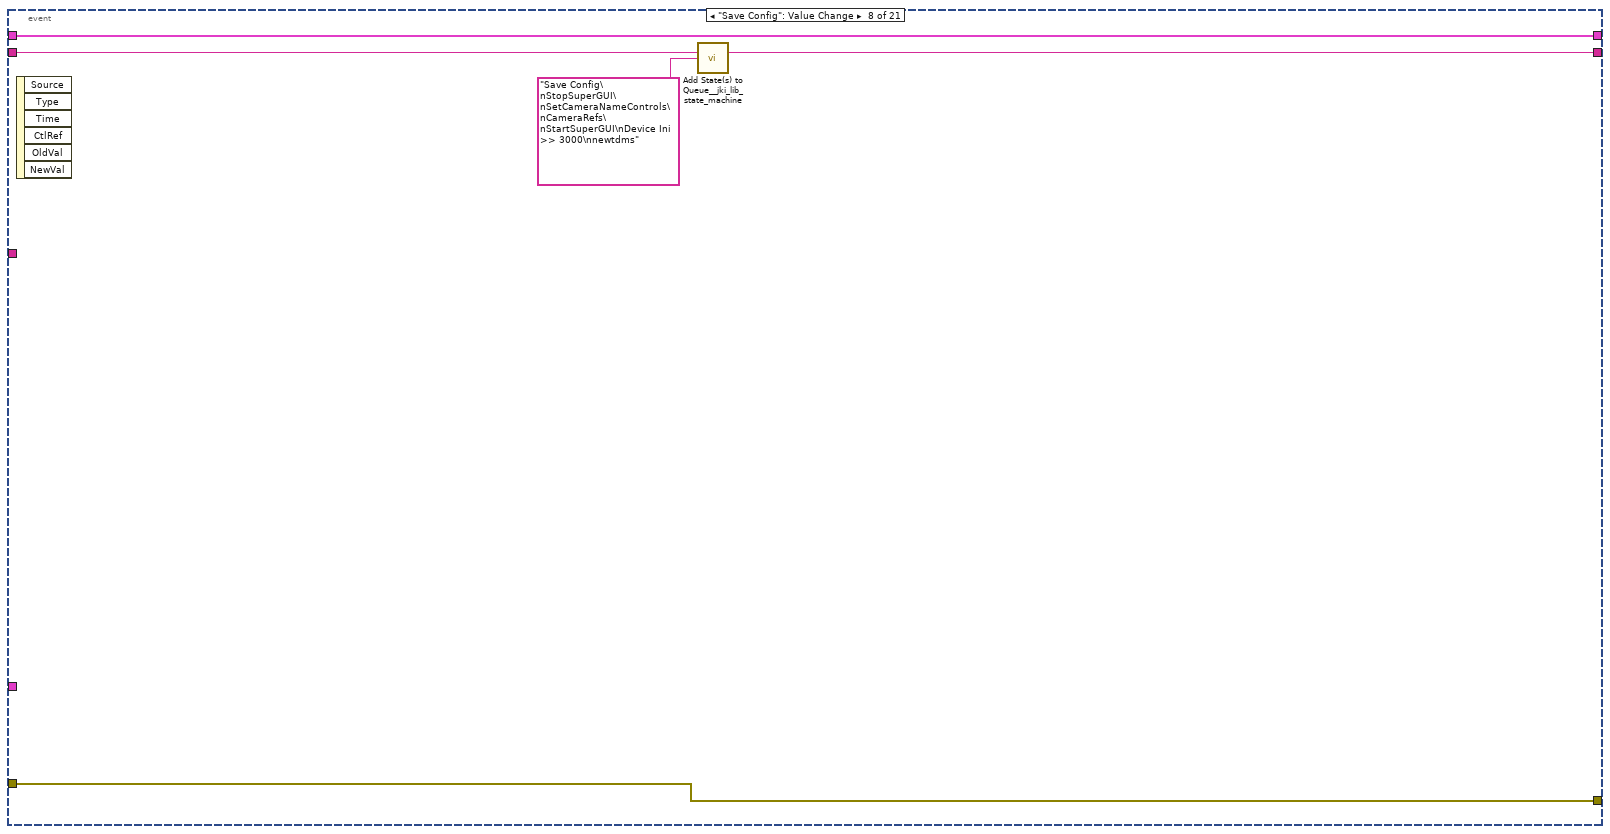
[diagram p17: hidden frame]
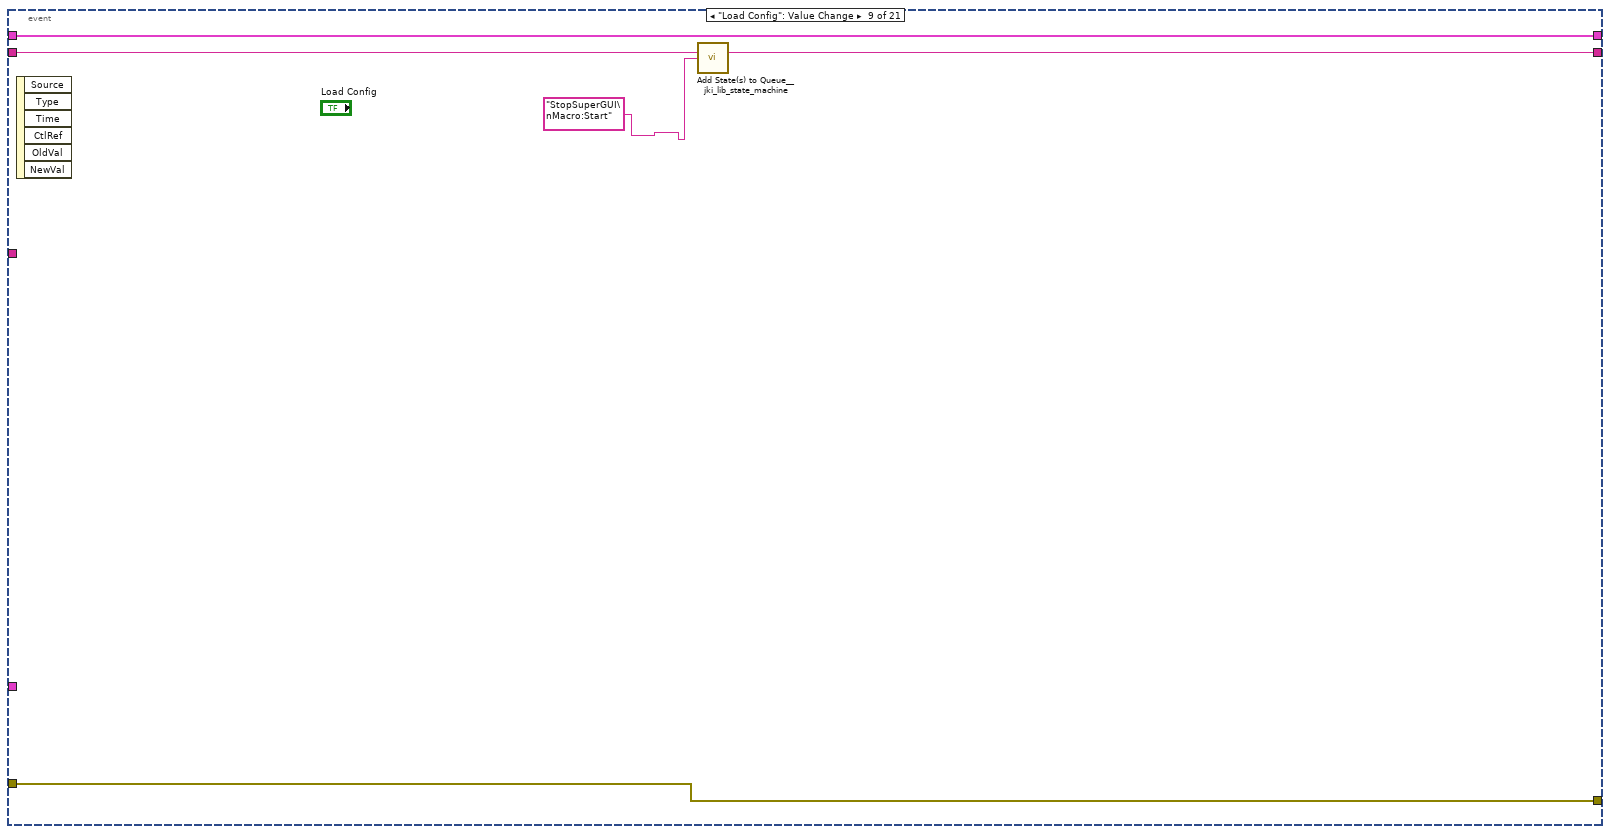
[diagram p18: hidden frame]
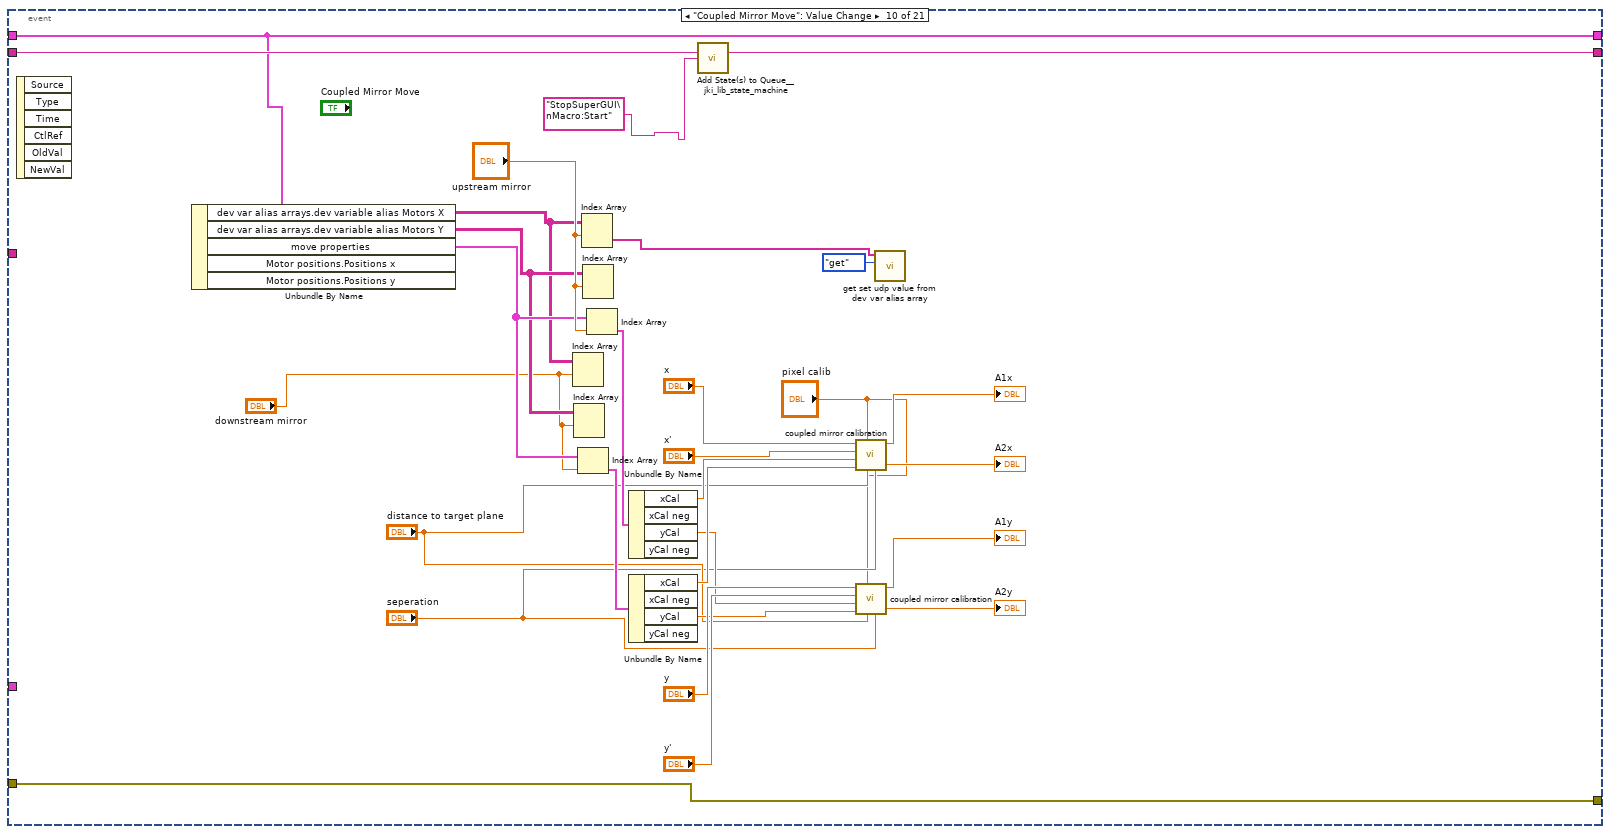
[diagram p19: hidden frame]
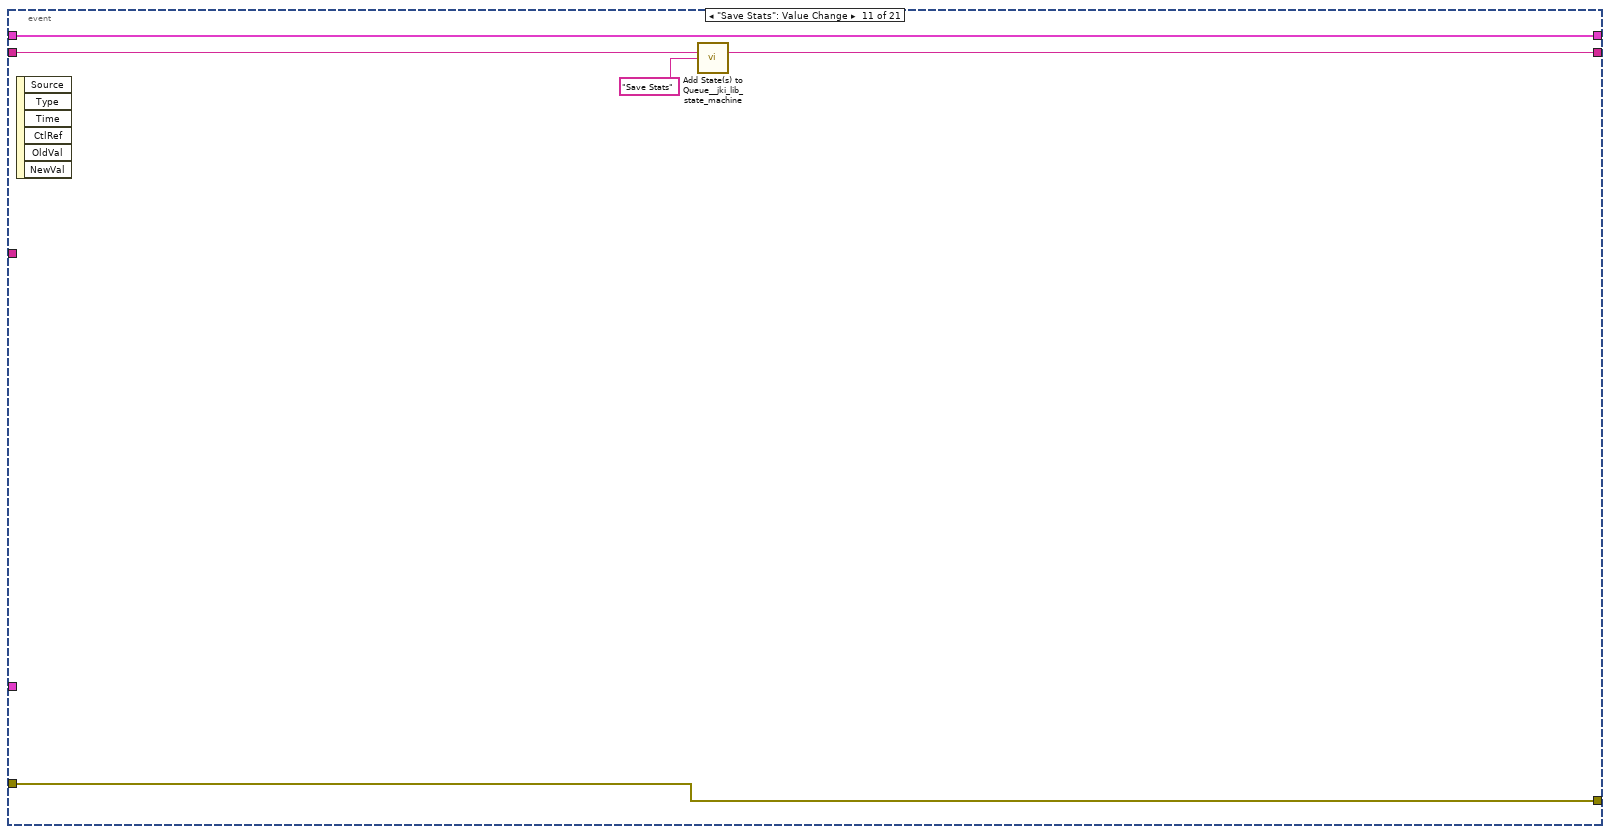
[diagram p20: hidden frame]
diagram:
  # "Motor Config"
  # "Load Config\nSetCameraNameControls\nCameraRefs\nStartSuperGUI\nDevice Ini >> 3000\nnewtdms"
  # "StopSuperGUI\nMacro:Start"
  # "why device ini every time in timeout? after a move, should reset img average"
  n1 = Tick Count (ms)() -> (millisecond timer value=→"millisecond timer value":u32)
  n2 = control-ref of="Target.X::1"() -> (w43:refnum<vi>)
  n3 = control-ref of="Target.Y::1"() -> (w42:refnum<vi>)
  n4 = control-ref of="Target.X::2"() -> (w41:refnum<vi>)
  n5 = control-ref of="Target.Y::2"() -> (w40:refnum<vi>)
  n6 = control-ref of="Target.X::3"() -> (w39:refnum<vi>)
  n7 = control-ref of="Target.Y::3"() -> (w38:refnum<vi>)
  n8 = control-ref of="Target.X::4"() -> (w37:refnum<vi>)
  n9 = control-ref of="Target.Y::4"() -> (w36:refnum<vi>)
  n10 = control-ref of="Target.X::5"() -> (w35:refnum<vi>)
  n11 = control-ref of="Target.Y::5"() -> (w34:refnum<vi>)
  n12 = control-ref of="Target.X::6"() -> (w33:refnum<vi>)
  n13 = control-ref of="Target.Y::6"() -> (w32:refnum<vi>)
  n14 = control-ref of="Target.X::7"() -> (w31:refnum<vi>)
  n15 = control-ref of="Target.Y::7"() -> (w30:refnum<vi>)
  n16 = control-ref of="Target.X::8"() -> (w29:refnum<vi>)
  n17 = control-ref of="Target.Y::8"() -> (w28:refnum<vi>)
  n18 = control-ref of="Target.X::9"() -> (w14:refnum<vi>)
  n19 = control-ref of="Target.Y::9"() -> (w13:refnum<vi>)
  n20 = control-ref of="Target.X::10"() -> (w12:refnum<vi>)
  n21 = control-ref of="Target.Y::10"() -> (w11:refnum<vi>)
  n22 = control-ref of="Target.X::11"() -> (w10:refnum<vi>)
  n23 = control-ref of="Target.Y::11"() -> (w9:refnum<vi>)
  n24 = control-ref of="Target.X::12"() -> (w8:refnum<vi>)
  n25 = control-ref of="Target.Y::12"() -> (w7:refnum<vi>)
  n26 = Bundle("Target.X::1"=w43, "Target.Y::1"=w42) -> (w27:T12)  [unwired: 1 in]
  n27 = Bundle("Target.X::2"=w41, "Target.Y::2"=w40) -> (w26:T13)  [unwired: 1 in]
  n28 = Bundle("Target.X::3"=w39, "Target.Y::3"=w38) -> (w25:T14)  [unwired: 1 in]
  n29 = Bundle("Target.X::4"=w37, "Target.Y::4"=w36) -> (w18:T15)  [unwired: 1 in]
  n30 = Bundle("Target.X::5"=w35, "Target.Y::5"=w34) -> (w24:T16)  [unwired: 1 in]
  n31 = Bundle("Target.X::6"=w33, "Target.Y::6"=w32) -> (w23:T17)  [unwired: 1 in]
  n32 = Bundle("Target.X::7"=w31, "Target.Y::7"=w30) -> (w22:T18)  [unwired: 1 in]
  n33 = Bundle("Target.X::8"=w29, "Target.Y::8"=w28) -> (w21:T19)  [unwired: 1 in]
  n34 = Bundle("Target.X::12"=w8, "Target.Y::12"=w7) -> (w3:T20)  [unwired: 1 in]
  n35 = Bundle("Target.X::9"=w14, "Target.Y::9"=w13) -> (w6:T21)  [unwired: 1 in]
  n36 = Bundle("Target.X::10"=w12, "Target.Y::10"=w11) -> (w5:T22)  [unwired: 1 in]
  n37 = Bundle("Target.X::11"=w10, "Target.Y::11"=w9) -> (w4:T23)  [unwired: 1 in]
  n38 = disable-structure shown="Disabled" {
    frame Disabled {
    }
    frame Enabled {
    }
  }
  n39 = Build Array(w27, w26, w25, w18, w24, w23, w22, w21, w6, w5, w4, w3) -> (w20:T24)
  n40 = property on="Feedback Global" class="Bool (strict)"("Value"=FALSE ("Feedback Global")) -> ()  [unwired: 2 in, 2 out]
  n41 = call <vilib>:"Add State(s) to Queue__jki_lib_state_machine.vi"("State(s) in (\"\")"="Macro: Initialize") -> ("States Out"=w47:string)  [unwired: 14 in]
  n42 = while "JKI - String-Based Queued State Machine (Basic) v1.0" {
    shift-right: [w62] -> w17
    shift-left: _ -> [w56]
    shift-right: [w64] -> w44
    shift-left: _ -> [w61]
    shift-right: [w50] -> _
    shift-left: w47 -> [w65]
    tunnel: w20 -> [w59]
    tunnel: [w51] -> w45
    tunnel: w20 -> [w58]
    stop <- w63 stop-if-true
    n43 = Unbundle By Name(w56) -> ("active cams"=w55:string[], "Mean Centroid X"=w54:dbl[][], "Mean Centroid Y"=w53:dbl[][], "Mean Size"=w52:dbl[][])
    n44 = call <vilib>:"Parse State Queue__jki_lib_state_machine.vi"("State Queue"=w65, "Error In (no error)"=w61) -> ("Remaining States"=w67:string, "Current State"=w48:string, "Arguments"=w66:string)  [unwired: 11 in]
    "Current State" <- w48
    n45 = local read "CCDs"() -> (w51:string[])
    n46 = case shown="\"\", \"Idle\"" w48 {
      selector: w48 -> [_ _ w405 _ _ _ _ _ _ _ _ _ _ _ _ _ _ _ _ _ _ _ _ _ _ _ _ _ _ _ _ _ _ _ _ _ _ _ _ _ _ _ _ _ _ _ _ _ _ _ _ _ _]
      tunnel: w67 -> [w135 w403 w409 w428 w435 w441 w446 w484 w496 w504 w514 w519 w526 w538 w563 w569 w612 w622 w630 w642 w647 w680 w741 w759 w817 w846 w874 w955 w1005 w1033 w1050 w1084 w1094 w1099 w1121 w1267 w1433 w1489 w1531 w1579 w1621 w1665 w1670 w1677 w1753 w1802 w1813 w1818 w1838 w1935 w1962 w1978 w2000]
      tunnel: w66 -> [_ _ _ _ _ _ _ _ _ _ _ _ w521 w533 _ _ _ _ _ _ _ w657 _ _ _ _ w852 _ w995 _ _ _ _ _ w1122 _ w1424 w1482 w1523 w1568 w1615 _ _ _ _ _ _ _ _ _ _ _ _]
      tunnel: w56 -> [w133 w400 w407 w418 w432 w439 w443 _ w489 w501 w511 w517 w524 w532 w560 w566 w572 w618 w627 w634 w644 w650 w739 w757 w815 w831 w867 w953 w992 w1029 w1047 w1077 w1089 w1096 w1110 w1250 w1418 w1473 w1512 w1563 w1617 w1658 w1667 w1674 w1749 w1799 w1810 w1815 w1834 w1933 w1959 w1980 w1991]
      tunnel: [w132 w401 w411 w426 errorcluster {"status"=FALSE, "code"=0, "source"=""} ("error out") w438 w444 w458 w494 w500 w512 w516 w522 w535 w561 w567 w610 w620 w628 w640 w645 w653 w738 w756 w814 w828 w870 w951 w997 w1031 w1039 w1082 w1092 w1097 w1150 w1280 w1414 w1487 w1529 w1558 w1613 w1663 w1668 w1675 w1750 w1800 w1811 w1816 w1827 w1904 w1960 w1976 w1998] -> w64
      tunnel: w61 -> [w131 w401 w410 w426 w429 w438 w444 w458 w486 w500 w512 w516 w523 w536 w561 w567 w610 w620 w628 w640 w645 w651 w738 w756 w814 w829 w871 w952 w982 w1031 w1040 w1082 w1092 w1097 w1150 w1280 w1413 w1487 w1529 w1557 w1614 w1663 w1668 w1675 w1751 w1800 w1811 w1816 w1828 w1931 w1960 w1976 w1998]
      tunnel: [w134 w402 w408 w427 w434 w440 w445 w483 w495 w503 w513 w518 w525 w537 w562 w568 w611 w621 w629 w641 w646 w679 w740 w758 w816 w845 w861 w954 w1004 w1032 w1049 w1083 w1093 w1098 w1104 w1281 w1432 w1488 w1530 w1578 w1620 w1664 w1669 w1676 w1752 w1801 w1812 w1817 w1837 w1934 w1961 w1977 w1999] -> w50
      tunnel: [_ _ _ _ _ TRUE _ _ _ _ _ _ _ _ _ _ _ _ _ _ _ _ _ _ _ _ _ _ _ _ _ _ _ _ _ _ _ _ _ _ _ _ _ _ _ _ _ _ _ _ _ _ _] -> w63
      tunnel: [w128 w400 w407 w417 w432 w439 w443 w459 w489 w501 w511 w517 w524 w532 w560 w566 w571 w617 w627 w634 w644 w672 w739 w757 w815 w830 w872 w953 w999 w1028 w1048 w1076 w1088 w1096 w1103 w1251 w1417 w1472 w1511 w1562 w1619 w1657 w1667 w1674 w1749 w1798 w1810 w1815 w1834 w1932 w1959 w1979 w1990] -> w62
      tunnel: "update speed [ms]" -> [w130 _ _ _ _ _ _ _ _ _ _ _ _ _ _ _ _ _ _ _ _ _ _ _ _ _ _ _ _ _ _ _ _ _ _ _ _ _ _ _ _ _ _ _ _ _ _ _ _ _ _ _ _]
      tunnel: w59 -> [w127 _ _ _ _ _ _ _ _ _ _ _ _ _ _ _ _ _ _ _ _ _ _ _ _ _ _ _ _ _ _ _ _ _ w1101 _ _ _ _ _ _ _ _ _ _ _ _ _ _ _ w1944 _ _]
      tunnel: w51 -> [w129 _ _ _ _ _ _ _ _ _ _ _ _ _ _ _ _ _ _ _ _ _ _ _ _ _ w873 _ w1000 _ _ _ _ _ w1114 w1252 w1431 _ _ w1577 w1616 _ _ w1673 _ _ _ _ w1833 _ _ _ _]
      tunnel: [w126 w399 w404 w416 w430 w436 w442 w451 w492 w497 w510 w515 w520 w531 w559 w564 w609 w613 w625 w631 w643 w662 w737 w742 w813 w826 w848 w938 w990 w1024 w1043 w1075 w1087 w1095 w1102 w1241 w1422 w1481 w1522 w1567 w1612 w1662 w1666 w1671 w1731 w1793 w1809 w1814 w1819 w1905 w1942 w1972 w1981] -> w49
      tunnel: w48 -> [w126 w399 w404 w416 w430 w436 w442 w451 w492 w497 w510 w515 w520 w531 w559 w564 w609 w613 w625 w631 w643 w662 w737 w742 w813 w826 w848 w938 w990 w1024 w1043 w1075 w1087 w1095 w1102 w1241 w1422 w1481 w1522 w1567 w1612 w1662 w1666 w1671 w1731 w1793 w1809 w1814 w1819 w1905 w1942 w1972 w1981]
      frame "", "Idle" {
        # "executes when the state queue is empty"
        n47 = event shown="[0] Timeout" {
          selector: _ -> [_ _ _ _ _ _ _ _ _ _ _ _ _ _ _ _ _ _ _ _ _]
          dyn-events: _ -> [_ _ _ _ _ _ _ _ _ _ _ _ _ _ _ _ _ _ _ _ _]
          timeout: w130 -> [_ _ _ _ _ _ _ _ _ _ _ _ _ _ _ _ _ _ _ _ _]
          tunnel: w135 -> [w154 w225 w240 w265 w270 w275 w281 w286 w291 w320 w325 w327 w342 w354 w359 w364 w370 w378 w387 w391 w398]
          tunnel: [w165 w224 w239 w264 w269 w274 w280 w285 w290 w319 w324 w326 w341 w353 w358 w363 w369 w377 w386 w390 w397] -> w134
          tunnel: w133 -> [w145 w222 w237 w261 w267 w272 w278 w283 w288 w292 w322 w330 w340 w352 w357 w362 w368 w376 w380 w392 w395]
          tunnel: [w171 w223 w238 w263 w268 w273 w279 w284 w289 w318 w323 w329 w335 w347 w356 w361 w367 w375 w385 w389 w396] -> w132
          tunnel: w131 -> [w161 w223 w238 w263 w268 w273 w279 w284 w289 w318 w323 w329 w336 w348 w356 w361 w367 w375 w385 w389 w396]
          tunnel: [w147 w222 w237 w260 w267 w272 w278 w283 w288 w292 w322 w330 w340 w352 w357 w362 w368 w376 w380 w392 w395] -> w128
          tunnel: w129 -> [w162 _ w233 _ _ _ _ _ _ _ _ _ _ _ _ _ _ _ _ _ _]
          tunnel: w127 -> [_ _ w235 _ _ _ _ _ _ _ _ _ _ _ _ _ _ _ _ _ _]
          event Timeout {
            n48 = event-data() -> ()  [unwired: 1 in, 1 out]
            n49 = Unbundle By Name(w145) -> ("Detection.img to avg"=w152:i32)
            n50 = Unbundle By Name(w145) -> ("Detection"=w150:T32, "active cams"=w137:string[])
            n51 = for {
              tunnel: w137 -> [w178] mode=indexing
              tunnel: [w177] -> w136 mode=indexing
              n52 = Concatenate Strings(w178, "_proc" ("string")) -> (w177:string)
              n53 = call "IMAQ Copy"("Image Dst"=w177, "Image Src"=w178) -> ("Image Dst Out"=→"Image Dst Out":T1)  [unwired: 4 in, 1 out]
            }
            n54 = Unbundle By Name(w145) -> ("active ccd"=w149:i32)
            n55 = Increment(x=w152) -> (x+1=w166:i32)
            n56 = Greater Or Equal?(x="#imgs avd so far", y=w166) -> (x >= y?=w164:bool)
            n57 = Increment(x="#imgs avd so far") -> (x+1=w168:dbl)
            n58 = call "centroid detection loop.vi"("CCDs"=w162, "error in (no error)"=w161, "active cams"=w136, "Detection in"=w150, "autodetect"="autodetect") -> ("error out"=w159:errorcluster, "# where centr y is 0"=w157:i32[], "Detection out"=w146:T33, "bounding rectangle"=→"Box":T3, "detected array"=→"detected":bool[], "Particle Reports (Pixels)"=w160:T34)  [unwired: 1 in]
            n59 = Select(t=0.0, s=w164, f=w168) -> (s? t:f=w167:dbl)
            n60 = Unbundle By Name(w145) -> ("Config loaded"=w144:bool)
            n61 = Index Array(array=w160, index (row)=w149) -> (element=w139:T6)  [unwired: 1 in]
            n62 = for {
              tunnel: w139 -> [w181] mode=indexing
              tunnel: [w180] -> w143 mode=indexing
              n63 = Unbundle By Name(w181) -> ("Area"=w180:dbl)
            }
            n64 = call-poly <userlib>:"Sort Array__ogtk.vi"("Order"=enum16{"ascending", "descending"}."descending", "Array in"=w143) -> ("Sorted Pointers"=w141:i32[])  [unwired: 8 in, 1 out]
            n65 = call-poly <userlib>:"Reorder Array2__ogtk.vi"("indices"=w141, "array"=w139) -> ("reordered array"=w140:variant[])  [unwired: 9 in]
            n66 = local write "#imgs avd so far"(w167) -> ()
            n67 = Variant To Data(type=w139, Variant=w140) -> (data=→"active ccd particles":T6)  [unwired: 1 in, 1 out]
            n68 = call <vilib>:"Clear Errors.vi"("error in (no error)"=w159) -> ("error out"=w171:errorcluster)  [unwired: 5 in, 1 out]
            n69 = Unbundle By Name(w146) -> ("img to avg"=w155:i32)
            n70 = for {
              tunnel: w157 -> [w214] mode=indexing
              tunnel: w136 -> [w220] mode=indexing
              shift-right: [w215] -> w172
              shift-left: "" ("GUIdevice 7") -> [w218]
              tunnel: [w209] -> w174 mode=indexing
              tunnel: "Detection Rate" -> [w213]
              tunnel: w167 -> [w211]
              tunnel: w152 -> [w207]
              # "averaging done?"
              n71 = Greater Or Equal?(x=w214, y=w207) -> (x >= y?=w210:bool)
              n72 = Multiply(x=w213, y=w211) -> (x*y=w212:dbl)
              n73 = Greater Or Equal?(x=w214, y=w212) -> (x >= y?=w208:bool)
              n74 = And(x=w210, y=w208) -> (x .and. y?=w209:bool)
              n75 = Select(t=w220, s=w209, f="") -> (s? t:f=w216:string)
              n76 = Concatenate Strings(w218, "\t", w216) -> (w215:string)
            }
            n77 = case shown="True" w144 {
              tunnel: w154 -> [w182 w185]
              tunnel: [w182 w184] -> w153
              frame False {
              }
              frame True {
                n78 = call <vilib>:"Add State(s) to Queue__jki_lib_state_machine.vi"("State(s) in (\"\")"=w185, "State(s) at Back (\"\")"="Device Ini" ("State(s) at Back (\"\")")) -> ("States Out"=w184:string)  [unwired: 13 in]
              }
            }
            n79 = case shown="True" w164 {
              tunnel: w146 -> [w186 w193]
              tunnel: [w186 w192] -> w148
              tunnel: w155 -> [_ w188]
              frame False {
              }
              frame True {
                # "avg done. clear arrays"
                n80 = Decrement(x=w188) -> (x-1=w191:i32)
                n81 = Initialize Array(0.0 ("element"), 12 ("dimension size"), w191) -> (w187:dbl[][])
                n82 = Bundle By Name(cluster=w193, "Centroid X"=w187, "Centroid Y"=w187, "Size"=w187) -> (w192:T33)
              }
            }
            n83 = Bundle By Name(cluster=w145, "Detection"=w148) -> (w147:T35)
            n84 = Or Array Elements(Boolean array=w174) -> (logical OR=w173:bool)
            n85 = case shown="True" w173 {
              tunnel: w172 -> [_ w201]
              tunnel: w153 -> [w194 w200]
              tunnel: [w194 w195] -> w165
              frame False {
                # "avg not done yet"
              }
              frame True {
                # "avg done."
                n86 = local read "Tab Cams"() -> (w198:T4)
                n87 = call <vilib>:"Build State String with Arguments__jki_lib_state_machine.vi"("Arguments (\"\")"=w201, "State"="detected") -> ("State with Arguments"=w199:string)  [unwired: 4 in]
                n88 = call <vilib>:"Add State(s) to Queue__jki_lib_state_machine.vi"("State(s) in Front (\"\")"=w199, "State(s) in (\"\")"=w200) -> ("States Out"=w196:string)  [unwired: 13 in]
                n89 = case shown="Default" w198 {
                  tunnel: w196 -> [w203 w206]
                  tunnel: "stats" ("State") -> [_ w205]
                  tunnel: [w203 w204] -> w195
                  frame Default {
                  }
                  frame "History" {
                    n90 = call <vilib>:"Add State(s) to Queue__jki_lib_state_machine.vi"("State(s) in Front (\"\")"=w205, "State(s) in (\"\")"=w206) -> ("States Out"=w204:string)  [unwired: 13 in]
                  }
                }
              }
            }
          }
          event "stop": Value Change {
            # "Exit Button Value Change (pressed) Event\n(this executes Macro: Exit to terminate the VI)"
            n91 = event-data() -> ()  [unwired: 1 in, 6 out]
            n92 = call <vilib>:"Add State(s) to Queue__jki_lib_state_machine.vi"("State(s) in Front (\"\")"="Macro: Exit", "State(s) in (\"\")"=w225) -> ("States Out"=w224:string)  [unwired: 13 in]
          }
          event Value Change {
            n93 = event-data() -> ()  [unwired: 1 in, 6 out]
            n94 = Unbundle By Name(w237) -> ("active ccd"=w229:i32, "Mean Centroid X"=w228:dbl[][], "Mean Centroid Y"=w227:dbl[][])
            n95 = Index Array(array=w233, index=w229) -> (element=w232:string)
            n96 = Concatenate Strings("Do want to update the target of " ("message"), w232, "?" ("string")) -> (w230:string)
            n97 = property on="Set Centriod Target" class="Bool (strict)"("Value"=FALSE) -> ()  [unwired: 2 in, 2 out]
            n98 = Two Button Dialog(message=w230) -> (T button?=w236:bool)  [unwired: 2 in]
            n99 = case shown="True" w236 {
              tunnel: w235 -> [_ w249]
              tunnel: w229 -> [_ w248]
              tunnel: w228 -> [_ w255]
              tunnel: w227 -> [_ w250]
              frame False {
              }
              frame True {
                n100 = Index Array(array=w255, index (row)=w248) -> (element=w254:dbl[])  [unwired: 1 in]
                n101 = Index Array(array=w250, index (row)=w248) -> (element=w251:dbl[])  [unwired: 1 in]
                n102 = Index Array(array=w249, index=w248) -> (element=w247:T20)
                n103 = Unbundle By Name(w247) -> ("Target.X::12"=w246:refnum<vi>, "Target.Y::12"=w245:refnum<vi>)
                n104 = Reverse 1D Array(array=w254) -> (reversed array=w253:dbl[])
                n105 = Reverse 1D Array(array=w251) -> (reversed array=w252:dbl[])
                n106 = Index Array(array=w253) -> (element=w244:dbl)  [unwired: 1 in]
                n107 = Index Array(array=w252) -> (element=w242:dbl)  [unwired: 1 in]
                n108 = To Unsigned Word Integer(number=w242) -> (unsigned 16bit integer=w241:u16)
                n109 = To Unsigned Word Integer(number=w244) -> (unsigned 16bit integer=w243:u16)
                n110 = disable-structure shown="Enabled" {
                  disable-tunnel: w246 -> [w259 _]
                  disable-tunnel: w243 -> [w258 _]
                  disable-tunnel: w245 -> [w257 _]
                  disable-tunnel: w241 -> [w256 _]
                  frame Enabled {
                    n111 = property class="DigNum (strict)"(reference=w259, "Val(Sgnl)"=w258) -> ()  [unwired: 1 in, 2 out]
                    n112 = property class="DigNum (strict)"(reference=w257, "Val(Sgnl)"=w256) -> ()  [unwired: 1 in, 2 out]
                  }
                  frame Disabled {
                  }
                }
              }
            }
            n113 = call <vilib>:"Add State(s) to Queue__jki_lib_state_machine.vi"("State(s) in (\"\")"=w240) -> ("States Out"=w239:string)  [unwired: 14 in]
          }
          event "Feedback Global": Value Change {
            # "Exit Button Value Change (pressed) Event\n(this executes Macro: Exit to terminate the VI)"
            n114 = event-data() -> ("NewVal"=w262:bool)  [unwired: 1 in, 5 out]
            n115 = call <vilib>:"Add State(s) to Queue__jki_lib_state_machine.vi"("State(s) in (\"\")"=w265) -> ("States Out"=w264:string)  [unwired: 14 in]
            n116 = Bundle By Name(cluster=w261, "Feedback global"=w262) -> (w260:T35)
          }
          event Value Change {
            n117 = event-data() -> ()  [unwired: 1 in, 6 out]
            n118 = call <vilib>:"Add State(s) to Queue__jki_lib_state_machine.vi"("State(s) in Front (\"\")"="set move props from control", "State(s) in (\"\")"=w270) -> ("States Out"=w269:string)  [unwired: 13 in]
          }
          event Value Change {
            n119 = event-data() -> ()  [unwired: 1 in, 6 out]
            n120 = call <vilib>:"Add State(s) to Queue__jki_lib_state_machine.vi"("State(s) in Front (\"\")"="set detection params from control", "State(s) in (\"\")"=w275) -> ("States Out"=w274:string)  [unwired: 13 in]
          }
          event "Reset History": Value Change {
            n121 = event-data() -> ()  [unwired: 1 in, 6 out]
            n122 = call <vilib>:"Add State(s) to Queue__jki_lib_state_machine.vi"("State(s) in (\"\")"=w281, "State(s) at Back (\"\")"="Reset History" ("State(s) at Back (\"\")")) -> ("States Out"=w280:string)  [unwired: 13 in]
            n123 = property on="Reset History" class="Bool (strict)"("Value"=FALSE ("Reset History")) -> ()  [unwired: 2 in, 2 out]
          }
          event "Save Config": Value Change {
            n124 = event-data() -> ()  [unwired: 1 in, 6 out]
            n125 = call <vilib>:"Add State(s) to Queue__jki_lib_state_machine.vi"("State(s) in (\"\")"=w286, "State(s) at Back (\"\")"="Save Config\nStopSuperGUI\nSetCameraNameControls\nCameraRefs\nStartSuperGUI\nDevice Ini >> 3000\nnewtdms" ("State(s) at Back (\"\")")) -> ("States Out"=w285:string)  [unwired: 13 in]
          }
          event "Load Config": Value Change {
            n126 = event-data() -> ()  [unwired: 1 in, 6 out]
            n127 = call <vilib>:"Add State(s) to Queue__jki_lib_state_machine.vi"("State(s) in (\"\")"=w291, "State(s) at Back (\"\")"="StopSuperGUI\nMacro:Start" ("State(s) at Back (\"\")")) -> ("States Out"=w290:string)  [unwired: 13 in]
          }
          event "Coupled Mirror Move": Value Change {
            n128 = event-data() -> ()  [unwired: 1 in, 6 out]
            n129 = Unbundle By Name(w292) -> ("dev var alias arrays.dev variable alias Motors X"=w310:string[][], "dev var alias arrays.dev variable alias Motors Y"=w311:string[][], "move properties"=w312:T11[])  [unwired: 2 out]
            n130 = Index Array(array=w310, index (row)="downstream mirror") -> ()  [unwired: 1 in, 1 out]
            n131 = Index Array(array=w311, index (row)="downstream mirror") -> ()  [unwired: 1 in, 1 out]
            n132 = Index Array(array=w312, index="downstream mirror") -> (element=w308:T11)
            n133 = Index Array(array=w310, index (row)="upstream mirror") -> (element=w315:string[])  [unwired: 1 in]
            n134 = Index Array(array=w311, index (row)="upstream mirror") -> ()  [unwired: 1 in, 1 out]
            n135 = Index Array(array=w312, index="upstream mirror") -> (element=w313:T11)
            n136 = Unbundle By Name(w313) -> ("xCal"=w302:dbl, "yCal"=w299:dbl)  [unwired: 2 out]
            n137 = Unbundle By Name(w308) -> ("xCal"=w303:dbl, "yCal"=w298:dbl)  [unwired: 2 out]
            n138 = call <vilib>:"Add State(s) to Queue__jki_lib_state_machine.vi"("State(s) in (\"\")"=w320, "State(s) at Back (\"\")"="StopSuperGUI\nMacro:Start" ("State(s) at Back (\"\")")) -> ("States Out"=w319:string)  [unwired: 13 in]
            n139 = call "coupled mirror calibration.vi"("seperation"="seperation", "distance to target plane"="distance to target plane", "pixel calib"="pixel calib", "xCal 2"=w303, "xCal"=w302, "x'"="x'", "x"="x") -> ("A2x"=→"A2x":dbl, "A1x"=→"A1x":dbl)  [unwired: 3 in]
            n140 = call "coupled mirror calibration.vi"("seperation"="seperation", "distance to target plane"="distance to target plane", "pixel calib"="pixel calib", "xCal 2"=w298, "xCal"=w299, "x'"="y'", "x"="y") -> ("A2x"=→"A2y":dbl, "A1x"=→"A1y":dbl)  [unwired: 3 in]
            n141 = call "get set udp value from dev var alias array.vi"("get or set"=enum16{"get", "set"}."get", "dev variable alias Motors X"=w315) -> ()  [unwired: 7 in, 3 out]
          }
          event "Save Stats": Value Change {
            n142 = event-data() -> ()  [unwired: 1 in, 6 out]
            n143 = call <vilib>:"Add State(s) to Queue__jki_lib_state_machine.vi"("State(s) in (\"\")"=w325, "State(s) at Back (\"\")"="Save Stats" ("State(s) at Back (\"\")")) -> ("States Out"=w324:string)  [unwired: 13 in]
          }
          event "Tab Cams": Value Change {
            n144 = event-data() -> ()  [unwired: 1 in, 6 out]
            n145 = call <vilib>:"Add State(s) to Queue__jki_lib_state_machine.vi"("State(s) in (\"\")"=w327, "State(s) at Back (\"\")"="stats" ("State")) -> ("States Out"=w326:string)  [unwired: 13 in]
          }
          event "Left", "Right": Value Change {
            n146 = event-data() -> ("CtlRef"=w339:refnum<vi>)  [unwired: 1 in, 5 out]
            n147 = property class="Bool (strict)"(reference=w339, error in=w336) -> (reference out=w338:refnum<vi>, error out=w337:errorcluster, "Label.Text"=w333:string)
            n148 = property class="Bool (strict)"(reference=w338, error in=w337, "Value"=FALSE) -> (error out=w335:errorcluster)  [unwired: 1 out]
            n149 = call <vilib>:"Build State String with Arguments__jki_lib_state_machine.vi"("Arguments (\"\")"=w333, "State"="ManMove X") -> ("State with Arguments"=w332:string)  [unwired: 4 in]
            n150 = call <vilib>:"Add State(s) to Queue__jki_lib_state_machine.vi"("State(s) in (\"\")"=w342, "State(s) at Back (\"\")"=w332) -> ("States Out"=w341:string)  [unwired: 13 in]
          }
          event "Up", "Down": Value Change {
            n151 = event-data() -> ("CtlRef"=w351:refnum<vi>)  [unwired: 1 in, 5 out]
            n152 = property class="Bool (strict)"(reference=w351, error in=w348) -> (reference out=w350:refnum<vi>, error out=w349:errorcluster, "Label.Text"=w345:string)
            n153 = property class="Bool (strict)"(reference=w350, error in=w349, "Value"=FALSE) -> (error out=w347:errorcluster)  [unwired: 1 out]
            n154 = call <vilib>:"Build State String with Arguments__jki_lib_state_machine.vi"("Arguments (\"\")"=w345, "State"="ManMove Y") -> ("State with Arguments"=w344:string)  [unwired: 4 in]
            n155 = call <vilib>:"Add State(s) to Queue__jki_lib_state_machine.vi"("State(s) in (\"\")"=w354, "State(s) at Back (\"\")"=w344) -> ("States Out"=w353:string)  [unwired: 13 in]
          }
          event "Center": Value Change {
            n156 = event-data() -> ()  [unwired: 1 in, 6 out]
            n157 = call <vilib>:"Add State(s) to Queue__jki_lib_state_machine.vi"("State(s) in (\"\")"=w359, "State(s) at Back (\"\")"="Center" ("State(s) at Back (\"\")")) -> ("States Out"=w358:string)  [unwired: 13 in]
          }
          event "new tdms", "tdms root": Value Change {
            n158 = event-data() -> ()  [unwired: 1 in, 6 out]
            n159 = call <vilib>:"Add State(s) to Queue__jki_lib_state_machine.vi"("State(s) in (\"\")"=w364, "State(s) at Back (\"\")"="newtdms" ("State(s) at Back (\"\")")) -> ("States Out"=w363:string)  [unwired: 13 in]
          }
          event "device ini": Value Change {
            n160 = event-data() -> ()  [unwired: 1 in, 6 out]
            n161 = property on="device ini" class="Bool (strict)"("Value"=FALSE ("test")) -> ()  [unwired: 2 in, 2 out]
            n162 = disable-structure shown="Enabled" {
              disable-tunnel: ["Device Ini" ("State(s) at Back (\"\")") "StopSuperGUI\nMacro:Start" ("State(s) at Back (\"\")")] -> w366
              frame Disabled {
              }
              frame Enabled {
              }
            }
            n163 = call <vilib>:"Add State(s) to Queue__jki_lib_state_machine.vi"("State(s) in (\"\")"=w370, "State(s) at Back (\"\")"=w366) -> ("States Out"=w369:string)  [unwired: 13 in]
          }
          event "clear error": Value Change {
            n164 = event-data() -> ()  [unwired: 1 in, 6 out]
            n165 = property on="clear error" class="Bool (strict)"("Value"=FALSE ("test")) -> ()  [unwired: 2 in, 2 out]
            n166 = local write "error out"(errorcluster {"status"=FALSE, "code"=0, "source"=""} ("error out")) -> ()
            n167 = call <vilib>:"Add State(s) to Queue__jki_lib_state_machine.vi"("State(s) in (\"\")"=w378) -> ("States Out"=w377:string)  [unwired: 14 in]
          }
          event "active CCDs": Value Change {
            n168 = event-data() -> ("NewVal"=w381:i32)  [unwired: 1 in, 5 out]
            n169 = Unbundle By Name(w380) -> ("active cams"=w382:string[])
            n170 = Index Array(array=w382, index=w381) -> (element=w383:string)
            n171 = call <vilib>:"Build State String with Arguments__jki_lib_state_machine.vi"("Arguments (\"\")"=w383, "State"="active" ("State(s) at Back (\"\")")) -> ("State with Arguments"=w379:string)  [unwired: 4 in]
            n172 = call <vilib>:"Add State(s) to Queue__jki_lib_state_machine.vi"("State(s) in (\"\")"=w387, "State(s) at Back (\"\")"=w379) -> ("States Out"=w386:string)  [unwired: 13 in]
          }
          event "img to avg": Value Change {
            n173 = event-data() -> ()  [unwired: 1 in, 6 out]
            n174 = call <vilib>:"Add State(s) to Queue__jki_lib_state_machine.vi"("State(s) in Front (\"\")"="ImgToAvg" ("State(s) at Back (\"\")"), "State(s) in (\"\")"=w391) -> ("States Out"=w390:string)  [unwired: 13 in]
          }
          event Panel Close? {
            # "Discard the event because we'll close the front panel ourselves in Macro: Exit"
            # "Close Panel button (pressed) Event\n(this executes Macro: Exit to terminate the VI)"
            n175 = event-data() -> ()  [unwired: 1 in, 1 out]
            n176 = call <vilib>:"Add State(s) to Queue__jki_lib_state_machine.vi"("State(s) in Front (\"\")"="Macro: Exit", "State(s) in (\"\")"=w398) -> ("States Out"=w397:string)  [unwired: 13 in]
            n177 = event-data("Discard?"=TRUE) -> ()  [unwired: 1 in, 1 out]
          }
        }
      }
      frame "---------- Core ----------" {
        # "Do not put any code in this frame.\n(it is a separator no-op)"
        n178 = call <vilib>:"Add State(s) to Queue__jki_lib_state_machine.vi"("State(s) in (\"\")"=w403) -> ("States Out"=w402:string)  [unwired: 14 in]
      }
      frame Default {
        w414 = 42 items=["No error", "Argument error", "Memory is full", "Out of zone", "End of file", "File already open", "Generic file I/O error", "File not found", "File permission error", "Disk is full", "Duplicate path", "Too many files open", "System feature not enabled", "Resource file not found", "Cannot add resource", "Resource not found", "Image not found", "Image memory error", "Pen does not exist", "Config type invalid", "Config token not found", "Config parse error", "Config memory error", "Bad external code format", "Bad external code offset", "External code not present", "Null window", "Destroy window error", "Null menu", "Print aborted", "Bad print record", "Print driver error", "Windows error during printing", "Memory error during printing", "Print dialog error", "Generic print error", "Invalid device refnum", "Device not found", "Device parameter error", "Device unit error", "Cannot open device", "Device call aborted", "Generic error", "Cancelled by user", "Object ID too low", "Object ID too high", "Object not in heap", "Unknown heap", "Unknown object (invalid DefProc)", "Unknown object (DefProc not in table)", "Message out of range", "Invalid (null) method", "Unknown message", "Manager call not supported", "Bad address", "Network operation in progress", "Network operation timed out", "Connection is busy", "Network attribute not supported", "Network error", "Address in use", "System out of memory", "Connection aborted", "Connection refused", "Not connected", "Already connected", "Connection closed", "Initialization error (interapplication manager)", "Bad occurrence", "Wait on unbound occurrence handler", "Occurrence queue overflow", "Datalog type conflict", "Unused", "Unrecognized type (interapplication manager)", "Memory corrupt", "Failed to make temporary DLL", "Old CIN version", "Drag socket not found", "Failed to load drop-object", "Failed to register OLE object", "Failed to release OLE object", "Format specifier type mismatch", "Unknown format specifier", "Too few format specifiers", "Too many format specifiers", "Scan failed", "Newer CIN version", "Error converting to variant", "Runtime menu error", "Password tampered", "Variant attribute not found", "Incompatible variant data type", "Event data is not available", "Event Store is not present", "Occurrence is not found", "Event Queue is not created", "Event info is not available", "Refnum passed is NULL", "Error retrieving Class GUID", "Error retrieving CoClass GUID", "Error retrieving TypeLib GUID.", "Bad built application magic bytes.", "Specific driver is different from the specific driver associated with the Logical Name.", "There is no session opened to the class driver.", "Max Error", "MAX - Error with config objects", "MAX - Error loading configuration", "MAX - Group not supported"]
        # "Current State"
        # "Do not delete, rename, or modify this frame.\n(this is used to capture unhandled states and typos)"
        # "Handle mistyped state name (developer tool)"
        n179 = Format Into String(format string="Software Exception: Unhandled State \"%s\"." ("message"), error in=w410, w405) -> (resulting string=w413:string, error out=w412:errorcluster)  [unwired: 1 in]
        n180 = call <vilib>:"Error Cluster From Error Code.vi"("show call chain? (False)"=TRUE, "error in (no error)"=w412, "error message (\"\")"=w413, "error code (0)"=w414) -> ("error out"=w411:errorcluster)  [unwired: 5 in]
        n181 = call <vilib>:"Add State(s) to Queue__jki_lib_state_machine.vi"("State(s) in (\"\")"=w409) -> ("States Out"=w408:string)  [unwired: 14 in]
      }
      frame "Initialize Core Data" {
        # "Do not delete, rename, or modify this frame.\n(this is used to determine panel behavior on exit)"
        # "originally closed?"
        # "exe?"
        # "If panel starts closed or is an EXE, then close it when we exit"
        n182 = property class="VI"() -> ("Front Panel.Open"=w425:bool)  [unwired: 2 in, 2 out]
        n183 = property class="App"() -> ("App.Kind"=w424:T25)  [unwired: 2 in, 2 out]
        n184 = control-ref of="Current VI Reference"() -> (w419:refnum<vi>)
        n185 = Not(x=w425) -> (.not. x?=w422:bool)
        n186 = Equal?(x=w424, y=T25."Run Time System" ("Application:Kind")) -> (x = y?=w421:bool)
        n187 = Or(x=w422, y=w421) -> (x .or. y?=w420:bool)
        n188 = Bundle By Name(cluster=w418, "Core.Current VI Reference"=w419, "Core.Close Panel on Exit?"=w420) -> (w417:T35)
        n189 = call <vilib>:"Add State(s) to Queue__jki_lib_state_machine.vi"("State(s) in (\"\")"=w428) -> ("States Out"=w427:string)  [unwired: 14 in]
      }
      frame "Error Handler" {
        # "Unhandled Error -- Display it"
        # "Handle any errors here.\nYou can also output any states to clean-up after errors occur"
        # "Clear error"
        n190 = call <vilib>:"Add State(s) to Queue__jki_lib_state_machine.vi"("State(s) in Front (\"\")"="/* Post Error States", "State(s) in (\"\")"=w435) -> ("States Out"=w434:string)  [unwired: 13 in]
        "error out" <- w429
      }
      frame "Exit" {
        # "Do not put any code in this frame.\n(No errors that occur here will be handled.)"
        n191 = call <vilib>:"Add State(s) to Queue__jki_lib_state_machine.vi"("State(s) in (\"\")"=w441) -> ("States Out"=w440:string)  [unwired: 14 in]
      }
      frame "---------- Data ----------" {
        # "Do not put any code in this frame.\n(It is a separator no-op. You can make a copy of this frame to create a new Data frame)"
        n192 = call <vilib>:"Add State(s) to Queue__jki_lib_state_machine.vi"("State(s) in (\"\")"=w446) -> ("States Out"=w445:string)  [unwired: 14 in]
      }
      frame "Data: Initialize" {
        w447 = FALSE  # Config loaded
        w449 = T32 {"detection para"=[{"Filter"=1, "Filter Para"={"X Size"=5, "Y Size"=5, "% Tolerance"=1}, "detection method"=4, "Particle filtering"=[{"Measurement Parameter"=35, "Range Lower Value"=0.0, "Range Upper Value"=0.0, "Range"=TRUE, "Measurement Type"=FALSE}], "Remove small Objects"=TRUE, "Restrict to round Objects"=FALSE, "Use Cam COM"=FALSE}, {"Filter"=1, "Filter Para"={"X Size"=5, "Y Size"=5, "% Tolerance"=1}, "detection method"=4, "Particle filtering"=[{"Measurement Parameter"=35, "Range Lower Value"=0.0, "Range Upper Value"=500.0, "Range"=FALSE, "Measurement Type"=FALSE}], "Remove small Objects"=TRUE, "Restrict to round Objects"=FALSE, "Use Cam COM"=FALSE}, {"Filter"=1, "Filter Para"={"X Size"=5, "Y Size"=5, "% Tolerance"=1}, "detection method"=4, "Particle filtering"=[{"Measurement Parameter"=35, "Range Lower Value"=0.0, "Range Upper Value"=500.0, "Range"=TRUE, "Measurement Type"=FALSE}], "Remove small Objects"=TRUE, "Restrict to round Objects"=FALSE, "Use Cam COM"=FALSE}, {"Filter"=1, "Filter Para"={"X Size"=5, "Y Size"=5, "% Tolerance"=1}, "detection method"=4, "Particle filtering"=[{"Measurement Parameter"=35, "Range Lower Value"=0.0, "Range Upper Value"=500.0, "Range"=TRUE, "Measurement Type"=FALSE}], "Remove small Objects"=TRUE, "Restrict to round Objects"=FALSE, "Use Cam COM"=FALSE}, {"Filter"=1, "Filter Para"={"X Size"=5, "Y Size"=5, "% Tolerance"=1}, "detection method"=4, "Particle filtering"=[{"Measurement Parameter"=35, "Range Lower Value"=0.0, "Range Upper Value"=500.0, "Range"=TRUE, "Measurement Type"=FALSE}], "Remove small Objects"=TRUE, "Restrict to round Objects"=FALSE, "Use Cam COM"=FALSE}, {"Filter"=1, "Filter Para"={"X Size"=5, "Y Size"=5, "% Tolerance"=1}, "detection method"=4, "Particle filtering"=[{"Measurement Parameter"=35, "Range Lower Value"=0.0, "Range Upper Value"=500.0, "Range"=TRUE, "Measurement Type"=FALSE}], "Remove small Objects"=TRUE, "Restrict to round Objects"=FALSE, "Use Cam COM"=FALSE}, {"Filter"=1, "Filter Para"={"X Size"=5, "Y Size"=5, "% Tolerance"=1}, "detection method"=4, "Particle filtering"=[{"Measurement Parameter"=35, "Range Lower Value"=0.0, "Range Upper Value"=500.0, "Range"=TRUE, "Measurement Type"=FALSE}], "Remove small Objects"=TRUE, "Restrict to round Objects"=FALSE, "Use Cam COM"=FALSE}, {"Filter"=1, "Filter Para"={"X Size"=5, "Y Size"=5, "% Tolerance"=1}, "detection method"=3, "Particle filtering"=[{"Measurement Parameter"=35, "Range Lower Value"=0.0, "Range Upper Value"=0.0, "Range"=FALSE, "Measurement Type"=FALSE}], "Remove small Objects"=TRUE, "Restrict to round Objects"=FALSE, "Use Cam COM"=FALSE}, {"Filter"=1, "Filter Para"={"X Size"=5, "Y Size"=5, "% Tolerance"=1}, "detection method"=4, "Particle filtering"=[{"Measurement Parameter"=35, "Range Lower Value"=0.0, "Range Upper Value"=0.0, "Range"=FALSE, "Measurement Type"=FALSE}], "Remove small Objects"=TRUE, "Restrict to round Objects"=FALSE, "Use Cam COM"=FALSE}, {"Filter"=1, "Filter Para"={"X Size"=5, "Y Size"=5, "% Tolerance"=1}, "detection method"=4, "Particle filtering"=[{"Measurement Parameter"=35, "Range Lower Value"=0.0, "Range Upper Value"=500.0, "Range"=TRUE, "Measurement Type"=FALSE}], "Remove small Objects"=TRUE, "Restrict to round Objects"=FALSE, "Use Cam COM"=FALSE}, {"Filter"=1, "Filter Para"={"X Size"=5, "Y Size"=5, "% Tolerance"=1}, "detection method"=4, "Particle filtering"=[{"Measurement Parameter"=35, "Range Lower Value"=0.0, "Range Upper Value"=500.0, "Range"=TRUE, "Measurement Type"=FALSE}], "Remove small Objects"=TRUE, "Restrict to round Objects"=FALSE, "Use Cam COM"=FALSE}, {"Filter"=1, "Filter Para"={"X Size"=5, "Y Size"=5, "% Tolerance"=1}, "detection method"=4, "Particle filtering"=[{"Measurement Parameter"=35, "Range Lower Value"=0.0, "Range Upper Value"=500.0, "Range"=TRUE, "Measurement Type"=FALSE}], "Remove small Objects"=TRUE, "Restrict to round Objects"=FALSE, "Use Cam COM"=FALSE}], "thresholds"=[{"Lower value"=93.0, "Upper value"=255.0}, {"Lower value"=105.0, "Upper value"=255.0}, {"Lower value"=0.0, "Upper value"=255.0}, {"Lower value"=127.0, "Upper value"=255.0}, {"Lower value"=0.0, "Upper value"=255.0}, {"Lower value"=0.0, "Upper value"=255.0}, {"Lower value"=0.0, "Upper value"=255.0}, {"Lower value"=0.0, "Upper value"=255.0}, {"Lower value"=0.0, "Upper value"=255.0}, {"Lower value"=0.0, "Upper value"=255.0}, {"Lower value"=0.0, "Upper value"=255.0}, {"Lower value"=0.0, "Upper value"=255.0}], "Centroid X"=[], "Centroid Y"=[], "Size"=[], "Centroid refs"=[], "img to avg"=6}  # Detection
        w450 = T36 {"Positions x"=[0.0, 0.0, 0.0, 0.0, 0.0, 0.0, 0.0, 0.0, 0.0, 0.0, 0.0, 0.0], "Positions y"=[0.0, 0.0, 0.0, 0.0, 0.0, 0.0, 0.0, 0.0, 0.0, 0.0, 0.0, 0.0]}  # Motor positions
        w452 = T37 {"dev variable alias"=[], "dev variable alias Motors X"=[], "dev variable alias Motors Y"=[]}  # dev var alias arrays
        w470 = dbl[][] []  # Offset Y stats
        w478 = dbl[][] []  # Mean Size
        w476 = T11[] [{"Tolerance [%]"=0.1, "Stepsize"=0.0001, "Invert Direction X"=FALSE, "Invert Direction Y"=TRUE, "enable feedback"=FALSE, "Set Centriod Target"=FALSE, "xCal"=0.0001, "xCal neg"=0.0001, "yCal"=0.0001, "yCal neg"=0.0001}, {"Tolerance [%]"=0.1, "Stepsize"=0.0001, "Invert Direction X"=FALSE, "Invert Direction Y"=TRUE, "enable feedback"=FALSE, "Set Centriod Target"=FALSE, "xCal"=0.0001, "xCal neg"=0.0001, "yCal"=0.0001, "yCal neg"=0.0001}, {"Tolerance [%]"=0.1, "Stepsize"=0.0001, "Invert Direction X"=FALSE, "Invert Direction Y"=TRUE, "enable feedback"=FALSE, "Set Centriod Target"=FALSE, "xCal"=0.0001, "xCal neg"=0.0001, "yCal"=0.0001, "yCal neg"=0.0001}, {"Tolerance [%]"=0.1, "Stepsize"=0.0001, "Invert Direction X"=FALSE, "Invert Direction Y"=TRUE, "enable feedback"=FALSE, "Set Centriod Target"=FALSE, "xCal"=0.0001, "xCal neg"=0.0001, "yCal"=0.0001, "yCal neg"=0.0001}, {"Tolerance [%]"=0.1, "Stepsize"=0.0001, "Invert Direction X"=FALSE, "Invert Direction Y"=TRUE, "enable feedback"=FALSE, "Set Centriod Target"=FALSE, "xCal"=0.0001, "xCal neg"=0.0001, "yCal"=0.0001, "yCal neg"=0.0001}, {"Tolerance [%]"=0.1, "Stepsize"=0.0001, "Invert Direction X"=FALSE, "Invert Direction Y"=TRUE, "enable feedback"=FALSE, "Set Centriod Target"=FALSE, "xCal"=0.0001, "xCal neg"=0.0001, "yCal"=0.0001, "yCal neg"=0.0001}, {"Tolerance [%]"=0.1, "Stepsize"=0.0001, "Invert Direction X"=FALSE, "Invert Direction Y"=TRUE, "enable feedback"=FALSE, "Set Centriod Target"=FALSE, "xCal"=0.0001, "xCal neg"=0.0001, "yCal"=0.0001, "yCal neg"=0.0001}, {"Tolerance [%]"=0.1, "Stepsize"=0.0001, "Invert Direction X"=FALSE, "Invert Direction Y"=TRUE, "enable feedback"=FALSE, "Set Centriod Target"=FALSE, "xCal"=0.0001, "xCal neg"=0.0001, "yCal"=0.0001, "yCal neg"=0.0001}, {"Tolerance [%]"=0.1, "Stepsize"=0.0001, "Invert Direction X"=FALSE, "Invert Direction Y"=TRUE, "enable feedback"=FALSE, "Set Centriod Target"=FALSE, "xCal"=0.0001, "xCal neg"=0.0001, "yCal"=0.0001, "yCal neg"=0.0001}, {"Tolerance [%]"=0.1, "Stepsize"=0.0001, "Invert Direction X"=FALSE, "Invert Direction Y"=TRUE, "enable feedback"=FALSE, "Set Centriod Target"=FALSE, "xCal"=0.0001, "xCal neg"=0.0001, "yCal"=0.0001, "yCal neg"=0.0001}, {"Tolerance [%]"=0.1, "Stepsize"=0.0001, "Invert Direction X"=FALSE, "Invert Direction Y"=TRUE, "enable feedback"=FALSE, "Set Centriod Target"=FALSE, "xCal"=0.0001, "xCal neg"=0.0001, "yCal"=0.0001, "yCal neg"=0.0001}, {"Tolerance [%]"=0.1, "Stepsize"=0.0001, "Invert Direction X"=FALSE, "Invert Direction Y"=TRUE, "enable feedback"=FALSE, "Set Centriod Target"=FALSE, "xCal"=0.0001, "xCal neg"=0.0001, "yCal"=0.0001, "yCal neg"=0.0001}, {"Tolerance [%]"=0.1, "Stepsize"=0.0001, "Invert Direction X"=FALSE, "Invert Direction Y"=TRUE, "enable feedback"=FALSE, "Set Centriod Target"=FALSE, "xCal"=0.0001, "xCal neg"=0.0001, "yCal"=0.0001, "yCal neg"=0.0001}]  # move properties
        w475 = T38 []  # active axis refs 2
        w469 = dbl[][] []  # Motor X
        w468 = dbl[][] []  # Motor Y
        w467 = string[] []  # active cams
        w453 = T39 {"STOP queue"=refnum, "SuperGUI ref"=refnum}  # Supergui
        w454 = dbl[] [0.0, 0.0, 0.0, 0.0, 0.0, 0.0, 0.0, 0.0, 0.0, 0.0, 0.0, 0.0]  # steps speed Y
        w455 = dbl[] [0.0, 0.0, 0.0, 0.0, 0.0, 0.0, 0.0, 0.0, 0.0, 0.0, 0.0, 0.0]  # steps speed X
        w456 = refnum<k34> refnum  # tdms ref
        w457 = bool[] [FALSE, FALSE, FALSE, FALSE, TRUE, TRUE, TRUE, FALSE, FALSE, FALSE, FALSE, FALSE]  # detected
        w464 = bool[] [FALSE, FALSE, FALSE, FALSE, FALSE, FALSE, FALSE, FALSE, FALSE, FALSE, FALSE, TRUE]  # speedmode Y
        w465 = bool[] [FALSE, FALSE, FALSE, FALSE, FALSE, FALSE, FALSE, FALSE, FALSE, FALSE, FALSE, TRUE]  # speedmode X
        w473 = FALSE  # Feedback global
        w474 = 0  # active ccd
        w482 = T40 {"Current VI Reference"=refnum, "Close Panel on Exit?"=FALSE}  # Core
        # "Initialize the shift-register data, here.\n(data names are defined by what you wire into the bundle function)"
        n193 = call <vilib>:"Add State(s) to Queue__jki_lib_state_machine.vi"("State(s) in (\"\")"=w484) -> ("States Out"=w483:string)  [unwired: 14 in]
        n194 = Unbundle By Name(w449) -> ("img to avg"=w448:i32)
        n195 = Bundle("Core"=w482, "Detection"=w449, "Mean Centroid X"="Mean Centroid X", "Mean Centroid Y"=dbl[][] [], "Offset X"="Offset X", "Offset Y"=dbl[][] [], "Offset X stats"=dbl[][] [], "Offset Y stats"=w470, "Mean Size"=w478, "Time"="Time", "move properties"=w476, "active axis refs 2"=w475, "active ccd"=w474, "Feedback global"=w473, "Motor X"=w469, "Motor Y"=w468, "active cams"=w467, "tdms ref"=w456, "active man refs"="active man refs", "detected"=w457, "speedmode X"=w465, "speedmode Y"=w464, "steps speed X"=w455, "steps speed Y"=w454, "Supergui"=w453, "dev var alias arrays"=w452, "Motor positions"=w450, "Config loaded"=w447) -> (w460:T35)  [unwired: 1 in]
        n196 = Initialize Array(0.0 ("element"), 12 ("dimension size"), w448) -> (w463:dbl[][])
        n197 = Bundle By Name(cluster=w460, "Detection.Centroid X"=w463, "Detection.Centroid Y"=w463, "Detection.Size"=w463) -> (w459:T35)
      }
      frame "Data: Cleanup" {
        # "Cleanup any data and references, here.\n(this is called automatically, by the Macro: Exit)"
        n198 = Unbundle By Name(w489) -> ("Core.Current VI Reference"=w493:refnum<vi>)
        n199 = Unbundle By Name(w489) -> ("tdms ref"=w491:refnum<k34>)
        n200 = call "close fgv udp connections.vi"("error in"=w486) -> ("error out"=w485:errorcluster)  [unwired: 10 in]
        n201 = TDMS Close(8:w485, 11:w491) -> (0:w490:errorcluster)  [unwired: 1 out]
        n202 = call <vilib>:"Clear Errors.vi"("error in (no error)"=w490) -> ("error out"=w488:errorcluster)  [unwired: 5 in, 1 out]
        n203 = Merge Errors(w488, w485) -> (w487:errorcluster)
        n204 = Close Reference(reference=w493, error in (no error)=w487) -> (error out=w494:errorcluster)
        n205 = call <vilib>:"Add State(s) to Queue__jki_lib_state_machine.vi"("State(s) in (\"\")"=w496) -> ("States Out"=w495:string)  [unwired: 14 in]
      }
      frame "StopSuperGUI" {
        # "Initialize the User Interface, here.\n(this is called automatically, by the Macro: Init)"
        n206 = Unbundle By Name(w501) -> ("Supergui.SuperGUI ref"=w499:refnum<vi>, "Supergui.STOP queue"=w502:refnum<queue>)
        n207 = Not A Number/Path/Refnum?(number/path/refnum=w499) -> (NaN/Path/Refnum?=w498:bool)
        n208 = case shown="False" w498 {
          tunnel: w502 -> [w509 _]
          tunnel: w499 -> [w505 _]
          frame False {
            n209 = Release Queue(queue=w509) -> (error out=w508:errorcluster)  [unwired: 2 in, 2 out]
            n210 = call-by-ref "Wait On Asynchronous Call"(reference=w505, error in=w508) -> (error out=w507:errorcluster, 0:"error out"=w506:errorcluster)  [unwired: 11 in, 1 out]
            n211 = call <vilib>:"Clear Errors.vi"("error in (no error)"=w506) -> ()  [unwired: 5 in, 2 out]
            n212 = call <vilib>:"Clear Errors.vi"("error in (no error)"=w507) -> ()  [unwired: 5 in, 2 out]
          }
          frame True {
          }
        }
        n213 = call <vilib>:"Add State(s) to Queue__jki_lib_state_machine.vi"("State(s) in (\"\")"=w504) -> ("States Out"=w503:string)  [unwired: 14 in]
      }
      frame "---------- UI ----------" {
        # "Do not put any code in this frame.\n(It is a separator no-op. You can make a copy of this frame to create a new UI frame)"
        n214 = call <vilib>:"Add State(s) to Queue__jki_lib_state_machine.vi"("State(s) in (\"\")"=w514) -> ("States Out"=w513:string)  [unwired: 14 in]
      }
      frame "UI: Initialize" {
        # "Initialize the User Interface, here.\n(this is called automatically, by the Macro: Init)"
        n215 = call <vilib>:"Add State(s) to Queue__jki_lib_state_machine.vi"("State(s) in (\"\")"=w519) -> ("States Out"=w518:string)  [unwired: 14 in]
      }
      frame "UI: Cursor Set" {
        # "Argument"
        # "Set and Unset Cursor Busy.\n(Usage: \"UI: Cursor Set >> Busy|Idle\")"
        n216 = case shown="\"Idle\", Default" w521 {
          tunnel: w523 -> [w528 w530]
          tunnel: [w527 w529] -> w522
          frame "Idle", Default {
            n217 = call <vilib>:"Unset Busy.vi"("error in (no error)"=w528) -> ("error out"=w527:errorcluster)  [unwired: 10 in]
          }
          frame "Busy" {
            n218 = call <vilib>:"Set Busy.vi"("error in (no error)"=w530) -> ("error out"=w529:errorcluster)  [unwired: 9 in, 1 out]
          }
        }
        n219 = call <vilib>:"Add State(s) to Queue__jki_lib_state_machine.vi"("State(s) in (\"\")"=w526) -> ("States Out"=w525:string)  [unwired: 14 in]
      }
      frame "UI: Front Panel State" {
        # "Argument"
        # "Set Front Panel Open or Closed\n(Usage: \"UI: Front Panel State >> Open|Close\")"
        n220 = Unbundle By Name(w532) -> ("Core.Current VI Reference"=w534:refnum<vi>)
        n221 = case shown="\"Open\", Default" w533 {
          tunnel: w536 -> [w542 w553]
          tunnel: [w543 w554] -> w535
          tunnel: w534 -> [_ _]
          frame "Open", Default {
            n222 = property class="VI"(error in=w542) -> (reference out=w540:refnum<vi>, error out=w541:errorcluster, "Front Panel.Open"=w539:bool)  [unwired: 1 in]
            n223 = case shown="False" w539 {
              tunnel: [w546 w549] -> w543
              tunnel: w541 -> [w545 w549]
              tunnel: w540 -> [w544 _]
              frame False {
                n224 = invoke class="VI" method="FP.Open"(reference=w544, error in=w545, "Activate"=TRUE, "State"=T26."Standard") -> (error out=w546:errorcluster)  [unwired: 1 in, 4 out]
              }
              frame True {
              }
            }
          }
          frame "Close" {
            n225 = property class="VI"(error in=w553) -> (reference out=w551:refnum<vi>, error out=w552:errorcluster, "Front Panel.Open"=w550:bool)  [unwired: 1 in]
            n226 = case shown="True" w550 {
              tunnel: [w555 w558] -> w554
              tunnel: w552 -> [w555 w557]
              tunnel: w551 -> [_ w556]
              frame False {
              }
              frame True {
                n227 = invoke class="VI" method="FP.Close"(reference=w556, error in=w557) -> (error out=w558:errorcluster)  [unwired: 1 in, 2 out]
              }
            }
          }
        }
        n228 = call <vilib>:"Add State(s) to Queue__jki_lib_state_machine.vi"("State(s) in (\"\")"=w538) -> ("States Out"=w537:string)  [unwired: 14 in]
      }
      frame "---------- Macro ----------" {
        # "Do not put any code in this frame.\n(It is a separator no-op. You can make a copy of this frame to create a new Macro frame)"
        n229 = call <vilib>:"Add State(s) to Queue__jki_lib_state_machine.vi"("State(s) in (\"\")"=w563) -> ("States Out"=w562:string)  [unwired: 14 in]
      }
      frame "Macro: Initialize" {
        # "Initialization Macro\n(This is called once, when the VI starts)"
        n230 = call <vilib>:"Add State(s) to Queue__jki_lib_state_machine.vi"("State(s) in Front (\"\")"="Data: Initialize\nCentroidRefs\nInitialize Core Data\nUI: Initialize\nUI: Front Panel State >> Open\nGetMotorsFromDB\nMacro:Start", "State(s) in (\"\")"=w569) -> ("States Out"=w568:string)  [unwired: 13 in]
      }
      frame "CentroidRefs" {
        n231 = control-ref of="centroidx::1"() -> (w608:refnum<vi>)
        n232 = control-ref of="centroidy::1"() -> (w607:refnum<vi>)
        n233 = control-ref of="centroidx::2"() -> (w606:refnum<vi>)
        n234 = control-ref of="centroidy::2"() -> (w605:refnum<vi>)
        n235 = control-ref of="centroidx::3"() -> (w604:refnum<vi>)
        n236 = control-ref of="centroidy::3"() -> (w603:refnum<vi>)
        n237 = control-ref of="centroidx::4"() -> (w602:refnum<vi>)
        n238 = control-ref of="centroidy::4"() -> (w601:refnum<vi>)
        n239 = control-ref of="centroidx::5"() -> (w600:refnum<vi>)
        n240 = control-ref of="centroidy::5"() -> (w599:refnum<vi>)
        n241 = control-ref of="centroidx::6"() -> (w598:refnum<vi>)
        n242 = control-ref of="centroidy::6"() -> (w597:refnum<vi>)
        n243 = control-ref of="centroidx::7"() -> (w596:refnum<vi>)
        n244 = control-ref of="centroidy::7"() -> (w595:refnum<vi>)
        n245 = control-ref of="centroidx::8"() -> (w594:refnum<vi>)
        n246 = control-ref of="centroidy::8"() -> (w593:refnum<vi>)
        n247 = control-ref of="centroidx::9"() -> (w584:refnum<vi>)
        n248 = control-ref of="centroidy::9"() -> (w583:refnum<vi>)
        n249 = control-ref of="centroidx::10"() -> (w582:refnum<vi>)
        n250 = control-ref of="centroidy::10"() -> (w581:refnum<vi>)
        n251 = control-ref of="centroidx::11"() -> (w580:refnum<vi>)
        n252 = control-ref of="centroidy::11"() -> (w579:refnum<vi>)
        n253 = control-ref of="centroidx::12"() -> (w578:refnum<vi>)
        n254 = control-ref of="centroidy::12"() -> (w577:refnum<vi>)
        n255 = Bundle("centroidx::1"=w608, "centroidy::1"=w607) -> (w592:T41)  [unwired: 1 in]
        n256 = Bundle("centroidx::2"=w606, "centroidy::2"=w605) -> (w591:T42)  [unwired: 1 in]
        n257 = Bundle("centroidx::3"=w604, "centroidy::3"=w603) -> (w590:T43)  [unwired: 1 in]
        n258 = Bundle("centroidx::4"=w602, "centroidy::4"=w601) -> (w585:T44)  [unwired: 1 in]
        n259 = Bundle("centroidx::5"=w600, "centroidy::5"=w599) -> (w589:T45)  [unwired: 1 in]
        n260 = Bundle("centroidx::6"=w598, "centroidy::6"=w597) -> (w588:T46)  [unwired: 1 in]
        n261 = Bundle("centroidx::7"=w596, "centroidy::7"=w595) -> (w587:T47)  [unwired: 1 in]
        n262 = Bundle("centroidx::8"=w594, "centroidy::8"=w593) -> (w586:T48)  [unwired: 1 in]
        n263 = Bundle("centroidx::12"=w578, "centroidy::12"=w577) -> (w573:T49)  [unwired: 1 in]
        n264 = Bundle("centroidx::9"=w584, "centroidy::9"=w583) -> (w576:T50)  [unwired: 1 in]
        n265 = Bundle("centroidx::10"=w582, "centroidy::10"=w581) -> (w575:T51)  [unwired: 1 in]
        n266 = Bundle("centroidx::11"=w580, "centroidy::11"=w579) -> (w574:T52)  [unwired: 1 in]
        n267 = Build Array(w592, w591, w590, w585, w589, w588, w587, w586, w576, w575, w574, w573) -> (w570:T53)
        n268 = Bundle By Name(cluster=w572, "Detection.Centroid refs"=w570) -> (w571:T35)
        n269 = call <vilib>:"Add State(s) to Queue__jki_lib_state_machine.vi"("State(s) in (\"\")"=w612) -> ("States Out"=w611:string)  [unwired: 14 in]
      }
      frame "GetMotorsFromDB" {
        n270 = call "get all aliases of a class.vi"("class (eg motor)"="motor") -> ("dev variable alias"=w616:string[][])  [unwired: 10 in]
        n271 = Bundle By Name(cluster=w618, "dev var alias arrays.dev variable alias"=w616) -> (w617:T35)
        n272 = Index Array(array=w616, index (col)=2 ("disabled index (col)")) -> (element=w614:string[])  [unwired: 1 in]
        "Names" <- w614
        n273 = property on="Motor Alias Y" class="Ring (strict)"("Strings []"=w614) -> ()  [unwired: 2 in, 2 out]
        n274 = property on="Motor Alias X" class="Ring (strict)"("Strings []"=w614) -> ()  [unwired: 2 in, 2 out]
        n275 = call <vilib>:"Add State(s) to Queue__jki_lib_state_machine.vi"("State(s) in (\"\")"=w622) -> ("States Out"=w621:string)  [unwired: 14 in]
      }
      frame "Macro:Start" {
        # "Dont believe JKI. This state is indeed called with \"load config button\" and more"
        # "Initialization Macro\n(This is called once, when the VI starts)"
        n276 = local write "config path"("" ("config path")) -> ()
        n277 = call <vilib>:"Add State(s) to Queue__jki_lib_state_machine.vi"("State(s) in Front (\"\")"="Load Config\nSetCameraNameControls\nCameraRefs\nStartSuperGUI\nDevice Ini >> 3000\nnewtdms\nImgToAvg", "State(s) in (\"\")"=w630) -> ("States Out"=w629:string)  [unwired: 13 in]
        n278 = local write "active CCDs"(0 ("active CCDs")) -> ()
      }
      frame "Macro: Exit" {
        # "Exit Macro\n(This is called once, when the VI exits)"
        n279 = Unbundle By Name(w634) -> ("Core.Close Panel on Exit?"=w633:bool)
        n280 = Select(t="UI: Front Panel State >> Close", s=w633, f="") -> (s? t:f=w637:string)
        n281 = call <vilib>:"Add State(s) to Queue__jki_lib_state_machine.vi"("State(s) in Front (\"\")"="StopSuperGUI" ("State(s) in Front (\"\")"), "State(s) in (\"\")"=w637, "State(s) at Back (\"\")"="Data: Cleanup\nExit") -> ("States Out"=w635:string)  [unwired: 12 in]
        n282 = call <vilib>:"Add State(s) to Queue__jki_lib_state_machine.vi"("State(s) in Front (\"\")"=w635, "State(s) in (\"\")"=w642) -> ("States Out"=w641:string)  [unwired: 13 in]
      }
      frame "---------- Ini and Configure ----------" {
        # "Template Separator\n(You can make a copy of, or modify, this frame)"
        n283 = call <vilib>:"Add State(s) to Queue__jki_lib_state_machine.vi"("State(s) in (\"\")"=w647) -> ("States Out"=w646:string)  [unwired: 14 in]
      }
      frame "Load Config" {
        w664 = T54 {"Camera"="", "Motor Alias X"=0, "Motor Alias Y"=0}  # Camera and motors
        # "Your code here.\n(You can make a copy of, or modify, this frame)"
        n284 = Unbundle By Name(w650) -> ("Detection.detection para"=w678:T9[], "move properties"=w675:T11[], "Detection.thresholds"=w670:cluster{"Lower value":sgl, "Upper value":sgl}[])
        n285 = Empty String/Path?(string/path=w657) -> (empty?=w658:bool)
        n286 = case shown="True" w658 {
          tunnel: [w696 w705] -> w654
          tunnel: w651 -> [w695 w704]
          tunnel: [w695 w703] -> w655
          tunnel: w657 -> [w697 _]
          frame False {
            n287 = String To Path(string=w697) -> (path=w696:path)
          }
          frame True {
            n288 = call <vilib>:"Application Directory.vi"() -> ("Application Directory"=w699:path)
            n289 = Build Path(base path=w699, name or relative path=path "cfg") -> (appended path=w701:path)
            n290 = call-poly <userlib>:"File Exists__ogtk.vi"("file path"=w701) -> ("exists"=w700:bool)  [unwired: 6 in, 1 out]
            n291 = case shown="True" w700 {
              tunnel: w701 -> [w709 w710]
              tunnel: [w708 w710] -> w698
              frame False {
                n292 = Create Folder(path (use dialog)=w709) -> (created path=w708:path)  [unwired: 2 in, 2 out]
              }
              frame True {
              }
            }
            n293 = call "File Dialog2"("start path"=w698, "error in"=w704, "pattern (all files)"="*.cfg", "pattern label"="config") -> ("selected path"=w705:path, "error out"=w703:errorcluster)  [unwired: 8 in, 2 out]
          }
        }
        n294 = property on="Load Config" class="Bool (strict)"("Value"=FALSE ("Load Config")) -> ()  [unwired: 2 in, 2 out]
        n295 = Path To String(path=w654) -> (string=→"config path":string)
        n296 = case shown="No Error" w655 {
          tunnel: w680 -> [w691 _]
          tunnel: [w690 _] -> w679
          tunnel: w655 -> [w685 _]
          tunnel: w654 -> [w684 _]
          tunnel: [w683 w694] -> w653
          tunnel: [w682 T27 {"Camera names"=[], "Motor aliases x"=[], "Motor aliases y"=[], "detection para"=[], "thresholds"=[], "move properties"=[], "tdms root"=path "c:/BP_DATAsd"} ("BP Configuration")] -> w652
          tunnel: w651 -> [_ w694]
          tunnel: [TRUE ("Config loaded") FALSE ("Config loaded")] -> w648
          frame No Error {
            w686 = T27 {"Camera names"=[], "Motor aliases x"=[], "Motor aliases y"=[], "detection para"=[], "thresholds"=[], "move properties"=[], "tdms root"=path "c:/BP_DATAsd"}  # BP Configuration
            n297 = call <userlib>:"MGI Read Anything.vi"("Type of Anything"=w686, "Error In"=w685, "Path (dialog)"=w684) -> ("Error Out"=w688:errorcluster, "Anything"=w687:variant)  [unwired: 5 in, 2 out]
            n298 = Variant To Data(error in=w688, type=w686, Variant=w687) -> (data=w682:T27, error out=w683:errorcluster)
            n299 = call <vilib>:"Add State(s) to Queue__jki_lib_state_machine.vi"("State(s) in (\"\")"=w691, "State(s) at Back (\"\")"="Motor Config" ("State(s) at Back (\"\")")) -> ("States Out"=w690:string)  [unwired: 13 in]
          }
          frame Error {
          }
        }
        n300 = Unbundle By Name(w652) -> ("Motor aliases x"=w669:string[], "Motor aliases y"=w666:string[], "Camera names"=w661:string[], "detection para"=w677:T9[], "move properties"=w676:T11[], "thresholds"=w671:cluster{"Lower value":sgl, "Upper value":sgl}[], "tdms root"=w656:path)
        n301 = local write "tdms root"(w656) -> ()
        n302 = Bundle By Name(cluster=w650, "Config loaded"=w648) -> (w649:T35)
        n303 = call-poly <userlib>:"Remove Duplicates from 1D Array__ogtk.vi"("Input Array"=w661) -> ("Output Array"=w660:string[])  [unwired: 1 out]
        "CCDs" <- w660
        n304 = property on="Motor Alias X" class="Ring (strict)"() -> ("Strings []"=w665:string[])  [unwired: 2 in, 2 out]
        n305 = for {
          tunnel: w660 -> [w733]
          tunnel: w677 -> [w735]
          tunnel: w676 -> [w734]
          shift-right: [w728] -> w674
          shift-left: w678 -> [w732]
          shift-right: [w726] -> w673
          shift-left: w675 -> [w731]
          tunnel: w671 -> [w727]
          shift-right: [w723] -> w667
          shift-left: w670 -> [w725]
          tunnel: w669 -> [w722]
          tunnel: w666 -> [w720]
          tunnel: w665 -> [w716]
          tunnel: w664 -> [w718]
          tunnel: [w713] -> w663 mode=indexing
          tunnel: w660 -> [w711] mode=indexing
          i -> [w721]
          n306 = call-poly <userlib>:"Filter 1D Array__ogtk.vi"("items to filter"=w711, "array"=w733) -> ("filtered item indices"=w736:i32[])  [unwired: 4 in, 1 out]
          n307 = Index Array(array=w736) -> (element=w719:i32)  [unwired: 1 in]
          n308 = Index Array(array=w720, index=w719) -> (element=w712:string)
          n309 = Index Array(array=w722, index=w719) -> (element=w715:string)
          n310 = Index Array(array=w735, index=w719) -> (element=w730:T9)
          n311 = Index Array(array=w734, index=w719) -> (element=w729:T11)
          n312 = Index Array(array=w727, index=w719) -> (element=w724:cluster{"Lower value":sgl, "Upper value":sgl})
          n313 = Search 1D Array(1D array=w716, element=w712) -> (index of element=w717:i32)  [unwired: 1 in]
          n314 = Search 1D Array(1D array=w716, element=w715) -> (index of element=w714:i32)  [unwired: 1 in]
          n315 = Bundle By Name(cluster=w718, "Camera"=w711, "Motor Alias Y"=w717, "Motor Alias X"=w714) -> (w713:T54)
          n316 = Replace Array Subset(array=w732, new element=w730, index=w721) -> (w728:T9[])
          n317 = Replace Array Subset(array=w731, new element=w729, index=w721) -> (w726:T11[])
          n318 = Replace Array Subset(array=w725, new element=w724, index=w721) -> (w723:cluster{"Lower value":sgl, "Upper value":sgl}[])
        }
        n319 = property on="Cameras and motors" class="Arr (strict)"("Value"=w663) -> ()  [unwired: 2 in, 2 out]
        n320 = Bundle By Name(cluster=w649, "Detection.detection para"=w674, "move properties"=w673, "Detection.thresholds"=w667) -> (w672:T35)
      }
      frame "MotorRefs" {
        n321 = call <vilib>:"Add State(s) to Queue__jki_lib_state_machine.vi"("State(s) in (\"\")"=w741) -> ("States Out"=w740:string)  [unwired: 14 in]
      }
      frame "SetCameraNameControls" {
        # "Initialize the User Interface, here.\n(this is called automatically, by the Macro: Init)"
        n322 = local read "CCDs"() -> (w755:string[])
        n323 = Index Array(array=w755) -> (element #1=w754:string, element #2=w753:string, element #3=w752:string, element #4=w751:string, element #5=w750:string, element #6=w749:string, element #7=w748:string, element #8=w747:string, element #9=w746:string, element #10=w745:string, element #11=w744:string, element #12=w743:string)  [unwired: 12 in]
        n324 = property on="GUIdevice 1" class="Str"("Val(Sgnl)"=w754) -> ()  [unwired: 2 in, 2 out]
        n325 = property on="GUIdevice 2" class="Str"("Val(Sgnl)"=w753) -> ()  [unwired: 2 in, 2 out]
        n326 = property on="GUIdevice 3" class="Str"("Val(Sgnl)"=w752) -> ()  [unwired: 2 in, 2 out]
        n327 = property on="GUIdevice 4" class="Str"("Val(Sgnl)"=w751) -> ()  [unwired: 2 in, 2 out]
        n328 = property on="GUIdevice 5" class="Str"("Val(Sgnl)"=w750) -> ()  [unwired: 2 in, 2 out]
        n329 = property on="GUIdevice 6" class="Str"("Val(Sgnl)"=w749) -> ()  [unwired: 2 in, 2 out]
        n330 = property on="GUIdevice 7" class="Str"("Val(Sgnl)"=w748) -> ()  [unwired: 2 in, 2 out]
        n331 = property on="GUIdevice 8" class="Str"("Val(Sgnl)"=w747) -> ()  [unwired: 2 in, 2 out]
        n332 = property on="GUIdevice 9" class="Str"("Val(Sgnl)"=w746) -> ()  [unwired: 2 in, 2 out]
        n333 = property on="GUIdevice 10" class="Str"("Val(Sgnl)"=w745) -> ()  [unwired: 2 in, 2 out]
        n334 = property on="GUIdevice 11" class="Str"("Val(Sgnl)"=w744) -> ()  [unwired: 2 in, 2 out]
        n335 = property on="GUIdevice 12" class="Str"("Val(Sgnl)"=w743) -> ()  [unwired: 2 in, 2 out]
        n336 = call <vilib>:"Add State(s) to Queue__jki_lib_state_machine.vi"("State(s) in (\"\")"=w759) -> ("States Out"=w758:string)  [unwired: 14 in]
      }
      frame "CameraRefs" {
        n337 = control-ref of="Display1"() -> (w786:refnum<vi>)
        n338 = control-ref of="Display2"() -> (w785:refnum<vi>)
        n339 = control-ref of="Display3"() -> (w784:refnum<vi>)
        n340 = control-ref of="Display4"() -> (w783:refnum<vi>)
        n341 = control-ref of="Display5"() -> (w782:refnum<vi>)
        n342 = control-ref of="Display6"() -> (w781:refnum<vi>)
        n343 = control-ref of="Display7"() -> (w780:refnum<vi>)
        n344 = control-ref of="Dsiplay8"() -> (w779:refnum<vi>)
        n345 = control-ref of="Display9"() -> (w778:refnum<vi>)
        n346 = control-ref of="Display10"() -> (w777:refnum<vi>)
        n347 = control-ref of="Display11"() -> (w776:refnum<vi>)
        n348 = control-ref of="Display12"() -> (w775:refnum<vi>)
        n349 = Build Array(w786, w785, w784, w783, w782, w781, w780, w779, w778, w777, w776, w775) -> (w774:refnum<vi>[])
        n350 = Build Array("GUIdevice 1", "GUIdevice 2", "GUIdevice 3", "GUIdevice 4", "GUIdevice 5", "GUIdevice 6", "GUIdevice 7", "GUIdevice 8", "GUIdevice 9", "GUIdevice 10", "GUIdevice 11", "GUIdevice 12") -> (w800:string[])
        n351 = for {
          tunnel: w800 -> [w820] mode=indexing
          tunnel: [w824] -> w799 mode=indexing
          tunnel: w774 -> [w821] mode=indexing
          tunnel: [w819] -> w773 mode=indexing
          tunnel: [w818] -> w760 mode=indexing
          w823 = T55 0 items=["Grayscale (U8)", "Grayscale (I16)", "Grayscale (SGL)", "Complex (CSG)", "RGB (U32)", "HSL (U32)", "RGB (U64)", "Grayscale (U16)"] ("Image Type")
          w825 = T55 0 items=["Grayscale (U8)", "Grayscale (I16)", "Grayscale (SGL)", "Complex (CSG)", "RGB (U32)", "HSL (U32)", "RGB (U64)", "Grayscale (U16)"] ("Image Type")
          n352 = Concatenate Strings(w820, "_proc" ("string")) -> (w818:string)
          n353 = property on="Property Node" class="ImageControl"(reference=w821, "Caption.Text"=w820) -> ()  [unwired: 1 in, 2 out]
          n354 = call "IMAQ Create"("Image Name"=w820, "Image Type"=w825) -> ("New Image"=w824:T1)  [unwired: 3 in, 1 out]
          n355 = call "IMAQ Create"("Image Name"=w818, "Image Type"=w823) -> ("New Image"=w819:T1)  [unwired: 3 in, 1 out]
        }
        "12camsproc" <- w760
        n356 = call <vilib>:"Add State(s) to Queue__jki_lib_state_machine.vi"("State(s) in (\"\")"=w817) -> ("States Out"=w816:string)  [unwired: 14 in]
        n357 = Index Array(array=w773) -> (element #1=→"Display1":T1, element #2=→"Display2":T1, element #3=→"Display3":T1, element #4=→"Display4":T1, element #5=→"Display5":T1, element #6=→"Display6":T1, element #7=→"Display7":T1, element #8=→"Dsiplay8":T1, element #9=→"Display9":T1, element #10=→"Display10":T1, element #11=→"Display11":T1, element #12=→"Display12":T1)  [unwired: 12 in]
        n358 = Index Array(array=w799) -> (element #1=→"image::1":T1, element #2=→"image::2":T1, element #3=→"image::3":T1, element #4=→"image::4":T1, element #5=→"image::5":T1, element #6=→"image::6":T1, element #7=→"image::7":T1, element #8=→"image::8":T1, element #9=→"image::9":T1, element #10=→"image::10":T1, element #11=→"image::11":T1, element #12=→"image::12":T1)  [unwired: 12 in]
      }
      frame "StartSuperGUI" {
        # "create stop queue for supergui and its clones"
        # "can make an icon"
        # "x100 abort will be dependent on caller VI\nx80 abort will be independent of caller vi, this will abort vi when labview is closed."
        # "Initialize the User Interface, here.\n(this is called automatically, by the Macro: Init)"
        n359 = vi-ref "GUI_Master_subvi_reentrant_queues.vi"() -> (w834:refnum<vi>)
        n360 = call "supergui create stop queue.vi"() -> ("STOP Queue out"=w835:refnum<queue>)  [unwired: 11 in]
        n361 = control-ref of="This Application"() -> (w838:refnum<vi>)
        n362 = property class="VI"(reference=w834) -> ("Path"=w833:path)  [unwired: 1 in, 2 out]
        n363 = control-ref of="This VI"() -> (w837:refnum<vi>)
        n364 = Create User Event(user event datatype=T28 {"EventEnum"=enum."new data", "Device name"="Device name"} ("New Event"), error in=w829) -> (user event=w839:refnum<user-event>, error out=w840:errorcluster)
        "tcp data event 2" <- w839
        n365 = Current VI's Menubar() -> (w836:refnum<k9>)
        n366 = register-events(w839) -> ()  [unwired: 2 in, 2 out]
        n367 = Open VI Reference(type specifier VI Refnum (for type only)=refnum<vi> refnum, vi path=w833, options=256, error in (no error)=w829) -> (vi reference=w844:refnum<vi>, error out=w843:errorcluster)  [unwired: 2 in]
        n368 = call <vilib>:"Add State(s) to Queue__jki_lib_state_machine.vi"("State(s) in (\"\")"=w846) -> ("States Out"=w845:string)  [unwired: 14 in]
        n369 = call-by-ref "Start Asynchronous Call"(reference=w844, error in=w843, "STOP Queue in"=w835, "This Application"=w838, 8:"error in (no error)"=w840, "tcp data event"=w839, "Caller menu reference"=w836, "Caller VI ref"=w837) -> (reference out=w832:refnum<vi>, error out=w828:errorcluster)  [unwired: 5 in, 1 out]
        n370 = Bundle By Name(cluster=w831, "Supergui.SuperGUI ref"=w832, "Supergui.STOP queue"=w835) -> (w830:T35)
      }
      frame "Device Ini" {
        n371 = Empty String/Path?(string/path=w852) -> (empty?=w869:bool)
        n372 = flat-sequence {
          tunnel: w873 -> [w876]
          tunnel: [w876] -> w847
          tunnel: w868 -> [w875]
          tunnel: w847 -> [w881]
          tunnel: [w879] -> w855
          frame #0 {
            # "check"
            n373 = Wait (ms)(milliseconds to wait=w875) -> ()  [unwired: 1 out]
          }
          frame #1 {
            # "check if cam images are new"
            n374 = local read "cam means"() -> (w877:sgl[])
            n375 = for {
              tunnel: w881 -> [w884] mode=indexing
              shift-right: [w889] -> w879
              shift-left: string[] [] -> [w890]
              tunnel: [w883] -> w878 mode=indexing
              shift-right: [w887] -> _
              shift-left: w877 -> [w887]
              i -> [w888]
              n376 = call "IMAQ Histograph"("Image"=w884) -> ("error out"=w882:errorcluster, "Mean Value"=w883:sgl)  [unwired: 7 in, 2 out]
              n377 = Index Array(array=w887, index=w888) -> (element=w886:sgl)
              n378 = call <vilib>:"Clear Errors.vi"("error in (no error)"=w882) -> ()  [unwired: 5 in, 2 out]
              n379 = Equal?(x=w883, y=w886) -> (x = y?=w885:bool)
              n380 = case shown="False" w885 {
                tunnel: w890 -> [w893 w894]
                tunnel: [w892 w894] -> w889
                tunnel: w884 -> [w891 _]
                frame False {
                  n381 = Build Array (concatenate)(w893, w891) -> (w892:string[])
                }
                frame True {
                }
              }
            }
            "cam means" <- w878
          }
        }
        n382 = case shown="False" w869 {
          tunnel: w852 -> [w930 _]
          tunnel: [w929 0] -> w868
          frame False {
            n383 = Decimal String To Number(string=w930) -> (number=w929:i32)  [unwired: 2 in, 1 out]
          }
          frame True {
          }
        }
        n384 = Unbundle By Name(w867) -> ("active cams"=w860:string[])
        n385 = Equal?(x=w852, y="T") -> (x = y?=w850:bool)
        n386 = Equal?(x=w860, y=w855) -> (x = y?=w866:bool[])
        n387 = Empty Array?(array=w860) -> (empty?=w865:bool)
        n388 = Not(x=w865) -> (.not. x?=w864:bool)
        n389 = Build Array (concatenate)(w866, w864) -> (w863:bool[])
        n390 = Array Size(array=w855) -> (size(s)=w859:i32)
        n391 = Array Size(array=w860) -> (size(s)=w858:i32)
        n392 = And Array Elements(Boolean array=w863) -> (logical AND=w856:bool)
        n393 = Equal?(x=w859, y=w858) -> (x = y?=w857:bool)
        n394 = And(x=w857, y=w856) -> (x .and. y?=w854:bool)
        n395 = Not(x=w854) -> (.not. x?=w851:bool)
        n396 = Or(x=w851, y=w850) -> (x .or. y?=w849:bool)
        n397 = call <vilib>:"Add State(s) to Queue__jki_lib_state_machine.vi"("State(s) in (\"\")"=w874) -> ("States Out"=w862:string)  [unwired: 14 in]
        n398 = case shown="True" w849 {
          tunnel: [w897 w912] -> w872
          tunnel: w871 -> [w896 w911]
          tunnel: [w896 w911] -> w870
          tunnel: w867 -> [w897 w908]
          tunnel: w855 -> [_ w899]
          tunnel: w862 -> [w895 w901]
          tunnel: [w895 w898] -> w861
          frame False {
          }
          frame True {
            # "#todo check repercussion of not loading config here"
            # "# active cams changed, perform configuration"
            n399 = local write "#imgs avd so far"(0.0 ("Numeric")) -> ()
            n400 = property on="active CCDs" class="LstBox (strict)"("Item Names"=w899) -> ()  [unwired: 2 in, 2 out]
            n401 = Bundle By Name(cluster=w908, "active cams"=w899) -> (w902:T35)
            n402 = Array Size(array=w899) -> (size(s)=w918:i32)
            n403 = Initialize Array(0.0 ("element"), w918, 0 ("dimension size")) -> (w913:dbl[][])
            n404 = Unbundle By Name(w902) -> ("Detection.img to avg"=w907:i32)
            n405 = Initialize Array(0.0 ("element"), 12 ("dimension size"), w907) -> (w906:dbl[][])
            n406 = for {
              N: 1 -> [_]
              shift-right: [w923] -> w916
              shift-left: timestamp[][] [] ("Time") -> [w925]
              n407 = for {
                N: 12 -> [_]
                tunnel: w925 -> [w928] mode=indexing
                tunnel: [w926] -> w923 mode=indexing
                n408 = Get Date/Time In Seconds() -> (seconds since 1Jan1904=w927:timestamp)
                n409 = Build Array (concatenate)(w928, w927) -> (w926:timestamp[])
              }
            }
            n410 = Bundle By Name(cluster=w902, "Offset X stats"=w913, "Offset Y stats"=w913, "Detection.Centroid X"=w906, "Detection.Centroid Y"=w906, "Mean Centroid X"=w913, "Mean Centroid Y"=w913, "Offset X"=w913, "Offset Y"=w913, "Detection.Size"=w906, "Mean Size"=w913, "Motor X"=w913, "Motor Y"=w913) -> (w912:T35)
            n411 = disable-structure shown="Enabled" {
              disable-tunnel: [w920 _] -> w904
              frame Enabled {
                n412 = property on="config path" class="Str"() -> ("Value"=w921:string)  [unwired: 2 in, 2 out]
                n413 = call <vilib>:"Build State String with Arguments__jki_lib_state_machine.vi"("Arguments (\"\")"=w921, "State"="Load Config" ("State(s) in Front (\"\")")) -> ("State with Arguments"=w920:string)  [unwired: 4 in]
              }
              frame Disabled {
              }
            }
            n414 = property on="Time" class="Arr (strict)"("Value"=w916) -> ()  [unwired: 2 in, 2 out]
            n415 = call <vilib>:"Add State(s) to Queue__jki_lib_state_machine.vi"("State(s) in (\"\")"=w901, "State(s) at Back (\"\")"="active\nCenter" ("State(s) in Front (\"\")")) -> ("States Out"=w905:string)  [unwired: 13 in]
            n416 = call <vilib>:"Add State(s) to Queue__jki_lib_state_machine.vi"("State(s) in (\"\")"=w905, "State(s) at Back (\"\")"=w904) -> ("States Out"=w898:string)  [unwired: 13 in]
            "name array" <- w899
          }
        }
      }
      frame "Save Config" {
        w944 = T27 {"Camera names"=[], "Motor aliases x"=[], "Motor aliases y"=[], "detection para"=[], "thresholds"=[], "move properties"=[], "tdms root"=path "c:/BP_DATAsd"}  # BP Configuration
        n417 = property on="Save Config" class="Bool (strict)"("Value"=FALSE ("Save Config")) -> ()  [unwired: 2 in, 2 out]
        n418 = local read "Cameras and motors"() -> (w939:T5)
        n419 = property on="Motor Alias X" class="Ring (strict)"() -> ("Strings []"=w940:string[])  [unwired: 2 in, 2 out]
        n420 = call "File Dialog"("pattern (all files)"="*.cfg", "pattern label"="config") -> ("selected path"=w934:path)  [unwired: 10 in, 3 out]
        n421 = for {
          tunnel: [w961] -> w943 mode=indexing
          tunnel: [w957] -> w942 mode=indexing
          tunnel: w940 -> [w959]
          tunnel: w939 -> [w962] mode=indexing
          tunnel: [w956] -> w937 mode=indexing
          n422 = Unbundle By Name(w962) -> ("Camera"=w956:string, "Motor Alias X"=w960:u16, "Motor Alias Y"=w958:u16)
          n423 = Index Array(array=w959, index=w958) -> (element=w957:string)
          n424 = Index Array(array=w959, index=w960) -> (element=w961:string)
        }
        n425 = Unbundle By Name(w953) -> ("move properties"=w947:T11[], "Detection.detection para"=w946:T9[], "Detection.thresholds"=w945:cluster{"Lower value":sgl, "Upper value":sgl}[])
        n426 = local read "tdms root"() -> (w936:path)
        n427 = Bundle By Name(cluster=w944, "Camera names"=w937, "move properties"=w947, "detection para"=w946, "thresholds"=w945, "Motor aliases x"=w943, "Motor aliases y"=w942, "tdms root"=w936) -> (w941:T27)
        n428 = disable-structure shown="Enabled" {
          disable-tunnel: w952 -> [w966 w974]
          disable-tunnel: [w965 w973] -> w951
          disable-tunnel: w934 -> [w964 w972]
          disable-tunnel: w941 -> [w963 w975]
          frame Disabled {
            n429 = Open/Create/Replace File(file path (use dialog)=w964, error in=w966, operation (0:open)=T29."replace or create with confirmation") -> (refnum out=w968:refnum<file>, error out=w969:errorcluster)  [unwired: 3 in, 1 out]
            n430 = Write to Binary File(file (use dialog)=w968, data=w963, error in=w969) -> (refnum out=w971:refnum<file>, error out=w970:errorcluster)  [unwired: 3 in, 1 out]
            n431 = Close File(refnum=w971, error in=w970) -> (error out=w965:errorcluster)  [unwired: 1 out]
          }
          frame Enabled {
            n432 = call <userlib>:"MGI Write Anything.vi"("Error In"=w974, "Anything"=w975, "Path (dialog)"=w972) -> ("Error Out"=w973:errorcluster)  [unwired: 6 in, 2 out]
          }
        }
        n433 = Path To String(path=w934) -> (string=w933:string)
        n434 = call <vilib>:"Build State String with Arguments__jki_lib_state_machine.vi"("Arguments (\"\")"=w933, "State"="Load Config" ("State(s) at Back (\"\")")) -> ("State with Arguments"=w932:string)  [unwired: 4 in]
        n435 = call <vilib>:"Add State(s) to Queue__jki_lib_state_machine.vi"("State(s) in Front (\"\")"=w932, "State(s) in (\"\")"=w955) -> ("States Out"=w954:string)  [unwired: 13 in]
      }
      frame "active" {
        # "problem. when trying to change move config or beam\ndet para, it kees getting overwritten here"
        n436 = Empty String/Path?(string/path=w995) -> (empty?=w994:bool)
        n437 = Unbundle By Name(w992) -> ("move properties"=w1002:T11[], "Detection.detection para"=w998:T9[], "active ccd"=w985:i32, "active cams"=w984:string[], "Detection.thresholds"=w976:cluster{"Lower value":sgl, "Upper value":sgl}[])
        n438 = Unbundle By Name(w992) -> ("dev var alias arrays.dev variable alias Motors X"=w989:string[][], "dev var alias arrays.dev variable alias Motors Y"=w987:string[][])
        n439 = call-poly <userlib>:"Filter 1D Array__ogtk.vi"("items to filter"=w995, "array"=w1000) -> ("filtered item indices"=w1003:i32[])  [unwired: 4 in, 1 out]
        n440 = Index Array(array=w1003) -> (element=w993:i32)  [unwired: 1 in]
        n441 = Select(t=w985, s=w994, f=w993) -> (s? t:f=w978:i32)
        n442 = Index Array(array=w1002, index=w978) -> (element=w1001:T11)
        n443 = Index Array(array=w998, index=w978) -> (element=w979:T9)
        n444 = Index Array(array=w976, index=w978) -> (element=w977:cluster{"Lower value":sgl, "Upper value":sgl})
        n445 = property on="move config" class="Clust (strict)"(error in=w982, "Value"=w1001) -> (error out=w996:errorcluster)  [unwired: 1 in, 1 out]
        n446 = local write "thresholds"(w977) -> ()
        n447 = Index Array(array=w984, index=w978) -> (element=→"Active CCD":string)
        n448 = property on="beam detection para" class="Clust (strict)"(error in=w996, "Value"=w979) -> (error out=w981:errorcluster)  [unwired: 1 in, 1 out]
        n449 = disable-structure shown="Enabled" {
          disable-tunnel: w989 -> [w1015 w1023]
          disable-tunnel: [w1013 w1022] -> w988
          disable-tunnel: w987 -> [w1011 w1021]
          disable-tunnel: [w1010 w1020] -> w986
          disable-tunnel: w978 -> [w1009 w1019]
          disable-tunnel: w981 -> [w1008 w1018]
          disable-tunnel: [w1006 w1016] -> w980
          frame Disabled {
            n450 = call "Beampointing get set motor position.vi"("Active CCD"=w1009, "error in (no error)"=w1008, "get or set"=enum16{"get", "set"}."get", "dev variable alias Motors X"=w1011) -> ("error out"=w1007:errorcluster, "Actual Position"=w1010:dbl)  [unwired: 6 in]
            n451 = call "Beampointing get set motor position.vi"("Active CCD"=w1009, "error in (no error)"=w1007, "get or set"=enum16{"get", "set"}."get", "dev variable alias Motors X"=w1015) -> ("error out"=w1006:errorcluster, "Actual Position"=w1013:dbl)  [unwired: 6 in]
          }
          frame Enabled {
            n452 = call "Beampointing get motor position tcp.vi"("Active CCD"=w1019, "error in (no error)"=w1018, "dev variable alias Motors X"=w1021) -> ("error out"=w1017:errorcluster, "value"=w1020:dbl)  [unwired: 7 in]
            n453 = call "Beampointing get motor position tcp.vi"("Active CCD"=w1019, "error in (no error)"=w1017, "dev variable alias Motors X"=w1023) -> ("error out"=w1016:errorcluster, "value"=w1022:dbl)  [unwired: 7 in]
          }
        }
        n454 = call <vilib>:"Add State(s) to Queue__jki_lib_state_machine.vi"("State(s) in (\"\")"=w1005) -> ("States Out"=w1004:string)  [unwired: 14 in]
        n455 = Bundle By Name(cluster=w992, "active ccd"=w978) -> (w999:T35)
        n456 = property on="Position 1" class="DigNum (strict)"(error in=w980, "Value"=w988) -> (error out=w991:errorcluster)  [unwired: 1 in, 1 out]
        n457 = property on="Position 2" class="DigNum (strict)"(error in=w991, "Value"=w986) -> (error out=w997:errorcluster)  [unwired: 1 in, 1 out]
      }
      frame "set detection params from control" {
        # "Your code here.\n(You can make a copy of, or modify, this frame)"
        n458 = Unbundle By Name(w1029) -> ("Detection.detection para"=w1025:T9[], "active ccd"=w1030:i32)
        n459 = Replace Array Subset(array=w1025, new element="beam detection para", index=w1030) -> (w1026:T9[])
        n460 = Bundle By Name(cluster=w1029, "Detection.detection para"=w1026) -> (w1028:T35)
        n461 = call <vilib>:"Add State(s) to Queue__jki_lib_state_machine.vi"("State(s) in (\"\")"=w1033) -> ("States Out"=w1032:string)  [unwired: 14 in]
      }
      frame "Motor Config" {
        n462 = for {
          tunnel: w1047 -> [w1070]
          tunnel: "Cameras and motors" -> [w1069] mode=indexing
          tunnel: [w1057] -> w1045 mode=indexing
          tunnel: [w1062] -> w1044 mode=indexing
          tunnel: [w1060] -> w1042 mode=indexing
          tunnel: [w1058] -> w1041 mode=indexing
          tunnel: w1040 -> [w1055]
          tunnel: [w1054] -> w1039
          tunnel: [w1052] -> w1038 mode=indexing
          tunnel: [w1051] -> w1037 mode=indexing
          w1053 = 3000 ("slow timeout ms (3000)")
          n463 = Unbundle By Name(w1070) -> ("dev var alias arrays.dev variable alias"=w1066:string[][])
          n464 = Index Array(array=w1066, index (col)=2 ("disabled index (col)")) -> (element=w1065:string[])  [unwired: 1 in]
          n465 = Unbundle By Name(w1069) -> ("Motor Alias X"=w1074:u16, "Motor Alias Y"=w1064:u16)
          n466 = property on="Motor Alias X" class="Ring (strict)"() -> ("Strings []"=w1063:string[])  [unwired: 2 in, 2 out]
          n467 = Index Array(array=w1063, index=w1074) -> (element=w1073:string)
          n468 = Search 1D Array(1D array=w1065, element=w1073) -> (index of element=w1072:i32)  [unwired: 1 in]
          n469 = Index Array(array=w1066, index (row)=w1072) -> (element=w1057:string[])  [unwired: 1 in]
          n470 = Index Array(array=w1063, index=w1064) -> (element=w1067:string)
          n471 = Search 1D Array(1D array=w1065, element=w1067) -> (index of element=w1068:i32)  [unwired: 1 in]
          n472 = Index Array(array=w1066, index (row)=w1068) -> (element=w1062:string[])  [unwired: 1 in]
          n473 = call "get set udp value from dev var alias array.vi"("slow timeout ms (3000)"=w1053, "error in (no error)"=w1055, "get or set"=enum16{"get", "set"}."get", "dev variable alias Motors X"=w1062) -> ("error out"=w1056:errorcluster, "No errors =T"=w1051:bool, "Numeric"=w1060:dbl)  [unwired: 5 in]
          n474 = call "get set udp value from dev var alias array.vi"("slow timeout ms (3000)"=w1053, "error in (no error)"=w1056, "get or set"=enum16{"get", "set"}."get", "dev variable alias Motors X"=w1057) -> ("error out"=w1054:errorcluster, "No errors =T"=w1052:bool, "Numeric"=w1058:dbl)  [unwired: 5 in]
        }
        n475 = call <vilib>:"Add State(s) to Queue__jki_lib_state_machine.vi"("State(s) in (\"\")"=w1050) -> ("States Out"=w1049:string)  [unwired: 14 in]
        n476 = And Array Elements(Boolean array=w1038) -> (logical AND=w1036:bool)
        n477 = And Array Elements(Boolean array=w1037) -> (logical AND=w1035:bool)
        n478 = And(x=w1036, y=w1035) -> (x .and. y?=→"all UDP in motor config good":bool)
        n479 = Bundle By Name(cluster=w1047, "dev var alias arrays.dev variable alias Motors X"=w1045, "dev var alias arrays.dev variable alias Motors Y"=w1044, "Motor positions.Positions x"=w1041, "Motor positions.Positions y"=w1042) -> (w1048:T35)
      }
      frame "set move props from control" {
        # "Your code here.\n(You can make a copy of, or modify, this frame)"
        n480 = Unbundle By Name(w1077) -> ("move properties"=w1081:T11[], "active ccd"=w1080:i32)
        n481 = Replace Array Subset(array=w1081, new element="move config", index=w1080) -> (w1078:T11[])
        n482 = Bundle By Name(cluster=w1077, "move properties"=w1078) -> (w1076:T35)
        n483 = call <vilib>:"Add State(s) to Queue__jki_lib_state_machine.vi"("State(s) in (\"\")"=w1084) -> ("States Out"=w1083:string)  [unwired: 14 in]
      }
      frame "set thresholds" {
        # "Your code here.\n(You can make a copy of, or modify, this frame)"
        n484 = Unbundle By Name(w1089) -> ("Detection.thresholds"=w1091:cluster{"Lower value":sgl, "Upper value":sgl}[], "active ccd"=w1090:i32)
        n485 = Replace Array Subset(array=w1091, new element="thresholds", index=w1090) -> (w1085:cluster{"Lower value":sgl, "Upper value":sgl}[])
        n486 = Bundle By Name(cluster=w1089, "Detection.thresholds"=w1085) -> (w1088:T35)
        n487 = call <vilib>:"Add State(s) to Queue__jki_lib_state_machine.vi"("State(s) in (\"\")"=w1094) -> ("States Out"=w1093:string)  [unwired: 14 in]
      }
      frame "----------Centroid & Move----------" {
        # "Template Separator\n(You can make a copy of, or modify, this frame)"
        n488 = call <vilib>:"Add State(s) to Queue__jki_lib_state_machine.vi"("State(s) in (\"\")"=w1099) -> ("States Out"=w1098:string)  [unwired: 14 in]
      }
      frame "detected" {
        n489 = Unbundle By Name(w1110) -> ("Offset X"=w1142:dbl[][], "Offset Y"=w1141:dbl[][], "Detection.Size"=w1140:dbl[][], "Mean Size"=w1139:dbl[][], "Time"=w1136:timestamp[][], "Motor X"=w1119:dbl[][], "Motor positions"=w1118:T36, "Motor Y"=w1117:dbl[][])  [unwired: 1 out]
        n490 = Spreadsheet String To Array(format string="%s", spreadsheet string=w1122, array type (2D Dbl)=string[] []) -> (array=w1113:string[])  [unwired: 1 in]
        n491 = for {
          tunnel: w1114 -> [w1154] mode=indexing
          tunnel: w1113 -> [w1153]
          tunnel: [w1152] -> w1112 mode=indexing
          n492 = for {
            tunnel: w1154 -> [w1157]
            tunnel: [w1156] -> w1151 mode=indexing
            tunnel: w1153 -> [w1155] mode=indexing
            n493 = Equal?(x=w1157, y=w1155) -> (x = y?=w1156:bool)
          }
          n494 = Or Array Elements(Boolean array=w1151) -> (logical OR=w1152:bool)
        }
        n495 = local read "Cameras and motors"() -> (w1100:T5)
        n496 = Unbundle By Name(w1110) -> ("Mean Centroid X"=w1145:dbl[][], "Mean Centroid Y"=w1144:dbl[][], "Detection.Centroid X"=w1147:dbl[][], "Detection.Centroid Y"=w1146:dbl[][])
        n497 = call <vilib>:"Add State(s) to Queue__jki_lib_state_machine.vi"("State(s) in (\"\")"=w1121) -> ("States Out"=w1120:string)  [unwired: 14 in]
        n498 = for {
          tunnel: w1147 -> [w1207]
          tunnel: w1146 -> [w1206]
          tunnel: w1145 -> [w1205]
          tunnel: w1144 -> [w1204]
          tunnel: [w1203] -> w1133 mode=indexing
          tunnel: [w1202] -> w1143 mode=indexing
          tunnel: w1142 -> [w1201]
          tunnel: w1141 -> [w1200]
          tunnel: [w1199] -> w1111 mode=indexing
          tunnel: [w1198] -> w1134 mode=indexing
          tunnel: w1140 -> [w1197]
          tunnel: w1139 -> [w1196]
          tunnel: [w1195] -> w1138 mode=indexing
          tunnel: w1136 -> [w1194]
          tunnel: [w1193] -> w1135 mode=indexing
          tunnel: w1119 -> [w1190]
          tunnel: w1118 -> [w1163]
          tunnel: w1117 -> [w1189]
          tunnel: [w1169] -> w1116 mode=indexing
          tunnel: [w1168] -> w1115 mode=indexing
          tunnel: w1112 -> [w1167]
          tunnel: w1101 -> [w1165]
          tunnel: w1100 -> [_] mode=indexing
          i -> [w1159]
          n499 = Index Array(array=w1165, index=w1159) -> (element=w1164:T20)
          n500 = Unbundle By Name(w1163) -> ("Positions x"=w1162:dbl[], "Positions y"=w1160:dbl[])
          n501 = Unbundle By Name(w1164) -> ("Target.X::12"=w1173:refnum<vi>, "Target.Y::12"=w1172:refnum<vi>)
          n502 = Index Array(array=w1190, index (row)=w1159) -> (element=w1191:dbl[])  [unwired: 1 in]
          n503 = Index Array(array=w1162, index=w1159) -> (element=w1161:dbl)
          n504 = Index Array(array=w1189, index (row)=w1159) -> (element=w1192:dbl[])  [unwired: 1 in]
          n505 = Index Array(array=w1167, index=w1159) -> (element=w1166:bool)
          n506 = Index Array(array=w1205, index (row)=w1159) -> (element=w1185:dbl[])  [unwired: 1 in]
          n507 = Index Array(array=w1204, index (row)=w1159) -> (element=w1186:dbl[])  [unwired: 1 in]
          n508 = Index Array(array=w1207, index (row)=w1159) -> (element=w1188:dbl[])  [unwired: 1 in]
          n509 = Index Array(array=w1206, index (row)=w1159) -> (element=w1187:dbl[])  [unwired: 1 in]
          n510 = Index Array(array=w1201, index (row)=w1159) -> (element=w1181:dbl[])  [unwired: 1 in]
          n511 = Index Array(array=w1200, index (row)=w1159) -> (element=w1180:dbl[])  [unwired: 1 in]
          n512 = Index Array(array=w1197, index (row)=w1159) -> (element=w1178:dbl[])  [unwired: 1 in]
          n513 = Index Array(array=w1196, index (row)=w1159) -> (element=w1177:dbl[])  [unwired: 1 in]
          n514 = Index Array(array=w1194, index (row)=w1159) -> (element=w1174:timestamp[])  [unwired: 1 in]
          n515 = Index Array(array=w1160, index=w1159) -> (element=w1158:dbl)
          n516 = property class="DigNum (strict)"(reference=w1173) -> ("Value"=w1171:dbl)  [unwired: 1 in, 2 out]
          n517 = property class="DigNum (strict)"(reference=w1172) -> ("Value"=w1170:dbl)  [unwired: 1 in, 2 out]
          n518 = call <vilib>:"Std Deviation and Variance.vi"("X"=w1188) -> ("mean"=w1184:dbl)  [unwired: 1 in, 2 out]
          n519 = call <vilib>:"Std Deviation and Variance.vi"("X"=w1187) -> ("mean"=w1183:dbl)  [unwired: 1 in, 2 out]
          n520 = call <vilib>:"Std Deviation and Variance.vi"("X"=w1178) -> ("mean"=w1176:dbl)  [unwired: 1 in, 2 out]
          n521 = Get Date/Time In Seconds() -> (seconds since 1Jan1904=w1175:timestamp)
          n522 = Subtract(x=w1171, y=w1184) -> (x-y=w1182:dbl)
          n523 = Subtract(x=w1170, y=w1183) -> (x-y=w1179:dbl)
          n524 = case shown="True" w1166 {
            tunnel: [w1220 w1239] -> w1203
            tunnel: [w1208 w1238] -> w1202
            tunnel: [w1209 w1237] -> w1199
            tunnel: [w1210 w1236] -> w1198
            tunnel: [w1211 w1235] -> w1195
            tunnel: [w1212 w1234] -> w1193
            tunnel: w1186 -> [w1218 w1233]
            tunnel: w1185 -> [w1219 w1232]
            tunnel: w1184 -> [_ w1231]
            tunnel: w1183 -> [_ w1230]
            tunnel: w1182 -> [_ w1229]
            tunnel: w1181 -> [w1217 w1228]
            tunnel: w1180 -> [w1216 w1227]
            tunnel: w1179 -> [_ w1226]
            tunnel: w1177 -> [w1215 w1225]
            tunnel: w1176 -> [_ w1224]
            tunnel: w1175 -> [w1213 w1223]
            tunnel: w1174 -> [w1214 w1222]
            frame False {
              w1221 = 0.0
              n525 = Build Array (concatenate)(w1219, w1221) -> (w1220:dbl[])
              n526 = Build Array (concatenate)(w1218, w1221) -> (w1208:dbl[])
              n527 = Build Array (concatenate)(w1217, w1221) -> (w1209:dbl[])
              n528 = Build Array (concatenate)(w1216, w1221) -> (w1210:dbl[])
              n529 = Build Array (concatenate)(w1215, w1221) -> (w1211:dbl[])
              n530 = Build Array (concatenate)(w1214, w1213) -> (w1212:timestamp[])
            }
            frame True {
              n531 = Build Array (concatenate)(w1232, w1231) -> (w1239:dbl[])
              n532 = Build Array (concatenate)(w1233, w1230) -> (w1238:dbl[])
              n533 = Build Array (concatenate)(w1228, w1229) -> (w1237:dbl[])
              n534 = Build Array (concatenate)(w1227, w1226) -> (w1236:dbl[])
              n535 = Build Array (concatenate)(w1225, w1224) -> (w1235:dbl[])
              n536 = Build Array (concatenate)(w1222, w1223) -> (w1234:timestamp[])
            }
          }
          n537 = Build Array (concatenate)(w1191, w1161) -> (w1169:dbl[])
          n538 = Build Array (concatenate)(w1192, w1158) -> (w1168:dbl[])
        }
        n539 = local write "#imgs avd so far"(0.0 ("Numeric")) -> ()
        n540 = Array Size(array=w1111) -> (size(s)=w1132:i32[])
        n541 = Index Array(array=w1132, index=1) -> (element=w1130:i32)
        "History Index" <- w1130
        n542 = call <vilib>:"Add State(s) to Queue__jki_lib_state_machine.vi"("State(s) in (\"\")"=w1120, "State(s) at Back (\"\")"="Check Move\ntdms" ("State(s) at Back (\"\")")) -> ("States Out"=w1124:string)  [unwired: 13 in]
        n543 = Unbundle By Name(w1110) -> ("Detection.img to avg"=w1107:i32)
        n544 = Initialize Array(0.0 ("element"), 12 ("dimension size"), w1107) -> (w1106:dbl[][])
        n545 = Bundle By Name(cluster=w1110, "Detection.Centroid X"=w1106, "Detection.Centroid Y"=w1106, "Mean Centroid X"=w1133, "Mean Centroid Y"=w1143, "Offset X"=w1111, "Offset Y"=w1134, "Mean Size"=w1138, "Detection.Size"=w1106, "Time"=w1135, "Motor X"=w1116, "Motor Y"=w1115) -> (w1103:T35)
        n546 = Greater?(x=w1130, y="History Size") -> (0:w1128:bool)
        n547 = Select(t="history" ("State(s) at Back (\"\")"), s=w1128, f="") -> (s? t:f=w1125:string)
        n548 = call <vilib>:"Add State(s) to Queue__jki_lib_state_machine.vi"("State(s) in (\"\")"=w1124, "State(s) at Back (\"\")"=w1125) -> ("States Out"=w1105:string)  [unwired: 13 in]
        n549 = call <vilib>:"Add State(s) to Queue__jki_lib_state_machine.vi"("State(s) in (\"\")"=w1105) -> ("States Out"=w1104:string)  [unwired: 14 in]
      }
      frame "Check Move" {
        n550 = Unbundle By Name(w1250) -> ("move properties"=w1260:T11[], "Mean Size"=w1259:dbl[][], "move properties"=w1258:T11[], "Offset X"=w1257:dbl[][], "Offset Y"=w1256:dbl[][], "active cams"=w1255:string[])
        n551 = Unbundle By Name(w1250) -> ("steps speed X"=w1249:dbl[], "steps speed Y"=w1248:dbl[])
        n552 = for {
          tunnel: w1258 -> [w1300]
          tunnel: w1257 -> [w1298]
          tunnel: w1256 -> [w1296]
          tunnel: w1259 -> [w1304]
          tunnel: [w1314] -> w1244 mode=indexing
          tunnel: [w1310] -> w1242 mode=indexing
          tunnel: w1255 -> [w1305] mode=indexing
          tunnel: [w1331] -> w1261 mode=indexing
          tunnel: [w1330] -> w1253 mode=indexing
          tunnel: w1260 -> [w1303]
          tunnel: [w1282] -> w1245 mode=indexing
          tunnel: [w1294] -> w1243 mode=indexing
          tunnel: "Speedmode" -> [w1308]
          tunnel: w1252 -> [w1306]
          shift-right: [w1287] -> w1247
          shift-left: w1249 -> [w1292]
          shift-right: [w1286] -> w1246
          shift-left: w1248 -> [w1291]
          tunnel: [w1283] -> w1240 mode=indexing
          n553 = call-poly <userlib>:"Filter 1D Array__ogtk.vi"("items to filter"=w1305, "array"=w1306) -> ("filtered item indices"=w1307:i32[])  [unwired: 4 in, 1 out]
          n554 = Index Array(array=w1307) -> (element=w1290:i32)  [unwired: 1 in]
          n555 = Index Array(array=w1303, index=w1290) -> (element=w1302:T11)
          n556 = Index Array(array=w1304, index (row)=w1290) -> (element=w1301:dbl[])  [unwired: 1 in]
          n557 = Index Array(array=w1300, index=w1290) -> (element=w1299:T11)
          n558 = Index Array(array=w1298, index (row)=w1290) -> (element=w1297:dbl[])  [unwired: 1 in]
          n559 = Index Array(array=w1296, index (row)=w1290) -> (element=w1295:dbl[])  [unwired: 1 in]
          n560 = Unbundle By Name(w1299) -> ("Tolerance [%]"=w1324:dbl)
          n561 = Reverse 1D Array(array=w1297) -> (reversed array=w1329:dbl[])
          n562 = Reverse 1D Array(array=w1295) -> (reversed array=w1328:dbl[])
          n563 = Reverse 1D Array(array=w1301) -> (reversed array=w1323:dbl[])
          n564 = Unbundle By Name(w1302) -> ("Stepsize"=w1285:dbl, "enable feedback"=w1313:bool)
          n565 = Index Array(array=w1329) -> (element=w1327:dbl)  [unwired: 1 in]
          n566 = Index Array(array=w1328) -> (element=w1326:dbl)  [unwired: 1 in]
          n567 = Index Array(array=w1323) -> (element=w1322:dbl)  [unwired: 1 in]
          n568 = Absolute Value(x=w1327) -> (abs(x)=w1293:dbl)
          n569 = Absolute Value(x=w1326) -> (abs(x)=w1309:dbl)
          n570 = Square Root(x=w1322) -> (sqrt(x)=w1321:dbl)
          n571 = Divide(x=w1324, y=100.0) -> (x/y=w1284:dbl)
          n572 = Multiply(x=w1321, y=w1284) -> (x*y=w1283:dbl)
          n573 = Not Equal To 0?(x=w1309) -> (x != 0?=w1311:bool)
          n574 = Not Equal To 0?(x=w1293) -> (x != 0?=w1316:bool)
          n575 = Greater Or Equal?(x=w1293, y=w1283) -> (x >= y?=w1315:bool)
          n576 = Greater Or Equal?(x=w1309, y=w1283) -> (x >= y?=w1312:bool)
          n577 = call "speedmode.vi"("offset X"=w1293, "offset Y"=w1309, "beamsize x tolerance"=w1283, "Speedmode @"=w1308, "step size"=w1285) -> ("steps speed Y"=w1288:dbl, "steps speed X"=w1289:dbl, "speedmode X"=w1282:bool, "speedmode Y"=w1294:bool)  [unwired: 3 in]
          n578 = Compound Arithmetic op=AND(w1313, w1316, w1315) -> (w1314:bool)
          n579 = Compound Arithmetic op=AND(w1313, w1312, w1311) -> (w1310:bool)
          n580 = Boolean To (0,1)(Boolean=w1310) -> (0, 1=w1317:i16)
          n581 = Multiply(x=w1317, y=w1309) -> (x*y=w1318:dbl)
          n582 = Boolean To (0,1)(Boolean=w1314) -> (0, 1=w1320:i16)
          n583 = Replace Array Subset(array=w1292, new element=w1289, index=w1290) -> (w1287:dbl[])
          n584 = Replace Array Subset(array=w1291, new element=w1288, index=w1290) -> (w1286:dbl[])
          n585 = Multiply(x=w1320, y=w1293) -> (x*y=w1319:dbl)
          n586 = Bundle(w1318, "GUIdevice 8"=w1305) -> (w1330:cluster{dbl, "GUIdevice 8":string})  [unwired: 1 in]
          n587 = Bundle(w1319, "GUIdevice 8"=w1305) -> (w1331:cluster{dbl, "GUIdevice 8":string})  [unwired: 1 in]
        }
        "required X" <- w1244
        "required Y" <- w1242
        "tolerances (pix)" <- w1240
        n588 = case shown="False" "Align" {
          tunnel: w1261 -> [w1337 w1342]
          tunnel: w1253 -> [w1336 w1339]
          tunnel: [w1335 w1341] -> w1264
          tunnel: [w1334 w1338] -> w1263
          frame False {
            n589 = Sort 1D Array(array=w1336) -> (sorted array=w1333:cluster{dbl, "GUIdevice 8":string}[])
            n590 = Sort 1D Array(array=w1337) -> (sorted array=w1332:cluster{dbl, "GUIdevice 8":string}[])
            n591 = Reverse 1D Array(array=w1333) -> (reversed array=w1334:cluster{dbl, "GUIdevice 8":string}[])
            n592 = Reverse 1D Array(array=w1332) -> (reversed array=w1335:cluster{dbl, "GUIdevice 8":string}[])
          }
          frame True {
            w1340 = cluster{dbl, "GUIdevice 8":string}[] [] ("Array")
            n593 = for {
              shift-right: [w1352] -> w1341
              shift-left: w1340 -> [w1354]
              tunnel: w1342 -> [w1353] mode=indexing
              n594 = Unbundle(w1353) -> (w1356:dbl)  [unwired: 1 out]
              n595 = Not Equal To 0?(x=w1356) -> (x != 0?=w1355:bool)
              n596 = case shown="True" w1355 {
                tunnel: w1354 -> [w1357 w1360]
                tunnel: w1353 -> [_ w1359]
                tunnel: [w1357 w1358] -> w1352
                frame False {
                }
                frame True {
                  n597 = Build Array (concatenate)(w1360, w1359) -> (w1358:cluster{dbl, "GUIdevice 8":string}[])
                }
              }
            }
            n598 = for {
              shift-right: [w1343] -> w1338
              shift-left: w1340 -> [w1345]
              tunnel: w1339 -> [w1344] mode=indexing
              n599 = Unbundle(w1344) -> (w1347:dbl)  [unwired: 1 out]
              n600 = Not Equal To 0?(x=w1347) -> (x != 0?=w1346:bool)
              n601 = case shown="True" w1346 {
                tunnel: w1345 -> [w1348 w1351]
                tunnel: w1344 -> [_ w1350]
                tunnel: [w1348 w1349] -> w1343
                frame False {
                }
                frame True {
                  n602 = Build Array (concatenate)(w1351, w1350) -> (w1349:cluster{dbl, "GUIdevice 8":string}[])
                }
              }
            }
          }
        }
        n603 = call <vilib>:"Add State(s) to Queue__jki_lib_state_machine.vi"("State(s) in (\"\")"=w1267) -> ("States Out"=w1266:string)  [unwired: 14 in]
        n604 = Bundle By Name(cluster=w1250, "speedmode X"=w1245, "speedmode Y"=w1243, "steps speed X"=w1247, "steps speed Y"=w1246) -> (w1251:T35)
        n605 = Index Array(array=w1263) -> (element=w1268:cluster{dbl, "GUIdevice 8":string})  [unwired: 1 in]
        n606 = Index Array(array=w1264) -> (element=w1269:cluster{dbl, "GUIdevice 8":string})  [unwired: 1 in]
        n607 = Empty Array?(array=w1263) -> (empty?=w1271:bool)
        n608 = Unbundle(w1269) -> (w1277:dbl)  [unwired: 1 out]
        n609 = Unbundle(w1268) -> (w1273:dbl)  [unwired: 1 out]
        n610 = Unbundle By Name(w1251) -> ("Feedback global"=w1278:bool)
        n611 = Empty Array?(array=w1264) -> (empty?=w1275:bool)
        n612 = property on="autodetect" class="Bool (strict)"("Value"=FALSE ("autodetect")) -> ()  [unwired: 2 in, 2 out]
        n613 = Equal To 0?(x=w1277) -> (x = 0?=w1276:bool)
        n614 = Equal To 0?(x=w1273) -> (x = 0?=w1272:bool)
        n615 = Or(x=w1276, y=w1275) -> (x .or. y?=w1274:bool)
        n616 = Or(x=w1272, y=w1271) -> (x .or. y?=w1270:bool)
        n617 = case shown="True" w1278 {
          tunnel: w1274 -> [_ w1379]
          tunnel: w1264 -> [_ w1378]
          tunnel: w1270 -> [_ w1376]
          tunnel: w1263 -> [_ w1375]
          tunnel: w1266 -> [w1361 w1374]
          tunnel: [w1361 w1373] -> w1279
          tunnel: w1245 -> [_ w1372]
          tunnel: w1244 -> [_ w1371]
          tunnel: w1243 -> [_ w1370]
          tunnel: w1242 -> [_ w1369]
          frame False {
          }
          frame True {
            n618 = case shown="False" w1379 {
              tunnel: w1378 -> [w1403 _]
              tunnel: w1374 -> [w1399 w1404]
              tunnel: [w1397 w1404] -> w1377
              frame False {
                n619 = Index Array(array=w1403) -> (element=w1402:cluster{dbl, "GUIdevice 8":string})  [unwired: 1 in]
                n620 = Unbundle By Name(w1402) -> ("GUIdevice 8"=w1401:string)
                n621 = call <vilib>:"Build State String with Arguments__jki_lib_state_machine.vi"("Arguments (\"\")"=w1401, "State"="Move X") -> ("State with Arguments"=w1398:string)  [unwired: 4 in]
                n622 = call <vilib>:"Add State(s) to Queue__jki_lib_state_machine.vi"("State(s) in (\"\")"=w1399, "State(s) at Back (\"\")"=w1398) -> ("States Out"=w1397:string)  [unwired: 13 in]
              }
              frame True {
              }
            }
            n623 = case shown="False" w1376 {
              tunnel: w1375 -> [w1395 _]
              tunnel: w1377 -> [w1391 w1396]
              tunnel: [w1389 w1396] -> w1373
              frame False {
                n624 = Index Array(array=w1395) -> (element=w1394:cluster{dbl, "GUIdevice 8":string})  [unwired: 1 in]
                n625 = Unbundle By Name(w1394) -> ("GUIdevice 8"=w1393:string)
                n626 = call <vilib>:"Build State String with Arguments__jki_lib_state_machine.vi"("Arguments (\"\")"=w1393, "State"="Move Y") -> ("State with Arguments"=w1390:string)  [unwired: 4 in]
                n627 = call <vilib>:"Add State(s) to Queue__jki_lib_state_machine.vi"("State(s) in (\"\")"=w1391, "State(s) at Back (\"\")"=w1390) -> ("States Out"=w1389:string)  [unwired: 13 in]
              }
              frame True {
              }
            }
            n628 = for {
              tunnel: w1372 -> [w1388] mode=indexing
              tunnel: w1371 -> [w1387] mode=indexing
              tunnel: [w1386] -> w1368 mode=indexing
              n629 = And(x=w1388, y=w1387) -> (x .and. y?=w1386:bool)
            }
            n630 = for {
              tunnel: w1370 -> [w1385] mode=indexing
              tunnel: w1369 -> [w1384] mode=indexing
              tunnel: [w1383] -> w1367 mode=indexing
              n631 = And(x=w1385, y=w1384) -> (x .and. y?=w1383:bool)
            }
            n632 = Or Array Elements(Boolean array=w1368) -> (logical OR=w1366:bool)
            n633 = Or Array Elements(Boolean array=w1367) -> (logical OR=w1365:bool)
            n634 = Or(x=w1366, y=w1365) -> (x .or. y?=w1364:bool)
            n635 = property on="alarms" class="Bool (strict)"() -> ("Value"=w1363:bool)  [unwired: 2 in, 2 out]
            n636 = And(x=w1363, y=w1364) -> (x .and. y?=w1362:bool)
            n637 = case shown="True" w1362 {
              frame False {
              }
              frame True {
                n638 = call <vilib>:"Beep.vi"("use system alert? (T)"=FALSE, "duration (msec)"=u32 750, "frequency (Hz)"=u32 750) -> ()  [unwired: 9 in]
              }
            }
          }
        }
        n639 = call <vilib>:"Add State(s) to Queue__jki_lib_state_machine.vi"("State(s) in (\"\")"=w1266, "State(s) at Back (\"\")"=w1279) -> ("States Out"=w1281:string)  [unwired: 13 in]
      }
      frame "Move X" {
        # "Your code here.\n(You can make a copy of, or modify, this frame)"
        n640 = Unbundle By Name(w1418) -> ("Offset X"=w1430:dbl[][])
        n641 = call-poly <userlib>:"Filter 1D Array__ogtk.vi"("items to filter"=w1424, "array"=w1431) -> ("filtered item indices"=w1427:i32[])  [unwired: 4 in, 1 out]
        n642 = Unbundle By Name(w1418) -> ("dev var alias arrays.dev variable alias Motors X"=w1420:string[][])
        n643 = Unbundle By Name(w1418) -> ("move properties"=w1423:T11[])
        n644 = for {
          tunnel: w1427 -> [w1459] mode=indexing
          tunnel: w1423 -> [w1463]
          shift-right: [w1458] -> w1425
          shift-left: i32[] [] ("filtered item indices") -> [w1461]
          n645 = Index Array(array=w1463, index=w1459) -> (element=w1462:T11)
          n646 = Unbundle By Name(w1462) -> ("enable feedback"=w1460:bool)
          n647 = case shown="True" w1460 {
            tunnel: w1461 -> [w1464 w1467]
            tunnel: w1459 -> [_ w1466]
            tunnel: [w1464 w1465] -> w1458
            frame False {
            }
            frame True {
              n648 = Build Array (concatenate)(w1467, w1466) -> (w1465:i32[])
            }
          }
        }
        n649 = Index Array(array=w1425) -> (element=w1415:i32)  [unwired: 1 in]
        n650 = call "Beampointing get set motor position.vi"("Active CCD"=w1415, "error in (no error)"=w1413, "get or set"=enum16{"get", "set"}."get", "dev variable alias Motors X"=w1420) -> ("error out"=w1411:errorcluster, "Actual Position"=w1419:dbl)  [unwired: 6 in]
        n651 = Index Array(array=w1430, index (row)=w1415) -> (element=w1429:dbl[])  [unwired: 1 in]
        n652 = Reverse 1D Array(array=w1429) -> (reversed array=w1428:dbl[])
        n653 = Index Array(array=w1428) -> (element=w1409:dbl)  [unwired: 1 in]
        n654 = Index Array(array=w1423, index=w1415) -> (element=w1405:T11)
        n655 = Unbundle By Name(w1405) -> ("Invert Direction X"=w1410:bool, "enable feedback"=w1412:bool)
        n656 = local read "Align"() -> (w1407:bool)
        n657 = call "relative move from offset and calibration.vi"("Align"=w1407, "axis"=enum16{"x", "y"}."x", "Offset"=w1409, "element"=w1405) -> ("relative move out"=w1408:dbl)  [unwired: 7 in]
        n658 = case shown="No Error" w1411 {
          selector: w1411 -> [w1435 w1456]
          tunnel: w1410 -> [_ _]
          tunnel: w1412 -> [w1445 _]
          tunnel: w1420 -> [w1444 _]
          tunnel: w1419 -> [w1443 _]
          tunnel: w1418 -> [w1442 w1457]
          tunnel: [w1438 w1457] -> w1417
          tunnel: w1415 -> [w1437 _]
          tunnel: w1408 -> [w1436 _]
          tunnel: [w1434 w1456] -> w1414
          frame No Error {
            n659 = case shown="True" w1445 {
              tunnel: w1436 -> [_ w1455]
              tunnel: w1444 -> [_ w1453]
              tunnel: w1437 -> [_ w1452]
              tunnel: w1443 -> [w1446 w1450]
              tunnel: [w1446 w1449] -> w1439
              tunnel: w1435 -> [_ w1448]
              tunnel: [_ w1447] -> w1434
              frame False {
              }
              frame True {
                n660 = Add(x=w1450, y=w1455) -> (x+y=w1451:dbl)
                n661 = call "Beampointing get set motor position.vi"("Active CCD"=w1452, "error in (no error)"=w1448, "Set position"=w1451, "get or set"=enum16{"get", "set"}."set", "dev variable alias Motors X"=w1453) -> ("error out"=w1447:errorcluster, "Actual Position"=w1449:dbl)  [unwired: 5 in]
              }
            }
            n662 = Unbundle By Name(w1442) -> ("Motor positions.Positions x"=w1441:dbl[])
            n663 = Replace Array Subset(array=w1441, new element=w1439, index=w1437) -> (w1440:dbl[])
            n664 = Bundle By Name(cluster=w1442, "Motor positions.Positions x"=w1440) -> (w1438:T35)
          }
          frame Error {
          }
        }
        n665 = call <vilib>:"Build State String with Arguments__jki_lib_state_machine.vi"("Arguments (\"\")"=w1424, "State"="Wait" ("State(s) in Front (\"\")")) -> ()  [unwired: 4 in, 1 out]
        n666 = call <vilib>:"Add State(s) to Queue__jki_lib_state_machine.vi"("State(s) in (\"\")"=w1433) -> ("States Out"=w1432:string)  [unwired: 14 in]
        "Moving X" <- w1424
      }
      frame "ManMove X" {
        # "Your code here.\n(You can make a copy of, or modify, this frame)"
        n667 = Unbundle By Name(w1473) -> ("dev var alias arrays.dev variable alias Motors X"=w1477:string[][])
        n668 = Unbundle By Name(w1473) -> ("move properties"=w1484:T11[], "active ccd"=w1470:i32)
        n669 = call "Beampointing get set motor position.vi"("Active CCD"=w1470, "get or set"=enum16{"get", "set"}."get", "dev variable alias Motors X"=w1477) -> ("error out"=w1468:errorcluster, "Actual Position"=w1478:dbl)  [unwired: 7 in]
        n670 = Index Array(array=w1484, index=w1470) -> (element=w1486:T11)
        n671 = Unbundle By Name(w1486) -> ("Invert Direction X"=w1485:bool)
        n672 = call <vilib>:"Add State(s) to Queue__jki_lib_state_machine.vi"("State(s) in Front (\"\")"="RestartAveraging" ("State(s) in Front (\"\")"), "State(s) in (\"\")"=w1489) -> ("States Out"=w1488:string)  [unwired: 13 in]
        n673 = case shown="\"Left\", Default" w1482 {
          tunnel: w1485 -> [w1493 w1503]
          tunnel: "StepSize" -> [w1492 w1502]
          tunnel: w1478 -> [w1491 w1501]
          tunnel: [w1490 w1500] -> w1476
          frame "Right" {
            n674 = case shown="False" w1493 {
              tunnel: w1491 -> [w1496 w1499]
              tunnel: w1492 -> [w1495 w1498]
              tunnel: [w1494 w1497] -> w1490
              frame False {
                n675 = Add(x=w1496, y=w1495) -> (x+y=w1494:dbl)
              }
              frame True {
                n676 = Subtract(x=w1499, y=w1498) -> (x-y=w1497:dbl)
              }
            }
          }
          frame "Left", Default {
            n677 = case shown="True" w1503 {
              tunnel: w1501 -> [w1506 w1509]
              tunnel: w1502 -> [w1505 w1508]
              tunnel: [w1504 w1507] -> w1500
              frame False {
                n678 = Subtract(x=w1506, y=w1505) -> (x-y=w1504:dbl)
              }
              frame True {
                n679 = Add(x=w1509, y=w1508) -> (x+y=w1507:dbl)
              }
            }
          }
        }
        n680 = call "Beampointing get set motor position.vi"("Active CCD"=w1470, "error in (no error)"=w1468, "Set position"=w1476, "get or set"=enum16{"get", "set"}."set", "dev variable alias Motors X"=w1477) -> ("Actual Position"=w1471:dbl)  [unwired: 5 in, 1 out]
        n681 = Unbundle By Name(w1473) -> ("Motor positions.Positions x"=w1475:dbl[])
        n682 = Replace Array Subset(array=w1475, new element=w1471, index=w1470) -> (w1474:dbl[])
        n683 = Bundle By Name(cluster=w1473, "Motor positions.Positions x"=w1474) -> (w1472:T35)
      }
      frame "ManMove Y" {
        # "Your code here.\n(You can make a copy of, or modify, this frame)"
        n684 = Equal?(x=w1523, y="Down") -> ()  [unwired: 1 out]
        n685 = Unbundle By Name(w1512) -> ("move properties"=w1527:T11[], "active ccd"=w1513:i32)
        n686 = Unbundle By Name(w1512) -> ("dev var alias arrays.dev variable alias Motors Y"=w1521:string[][])
        n687 = call "Beampointing get set motor position.vi"("Active CCD"=w1513, "get or set"=enum16{"get", "set"}."get", "dev variable alias Motors X"=w1521) -> ("Actual Position"=w1517:dbl)  [unwired: 7 in, 1 out]
        n688 = Index Array(array=w1527, index=w1513) -> (element=w1528:T11)
        n689 = property on="StepSize" class="DigNum (strict)"() -> ("Value"=w1524:dbl)  [unwired: 2 in, 2 out]
        n690 = Unbundle By Name(w1528) -> ("Invert Direction Y"=w1525:bool)
        n691 = case shown="\"Up\", Default" w1523 {
          tunnel: w1525 -> [w1535 w1545]
          tunnel: w1524 -> [w1534 w1544]
          tunnel: [w1533 w1542] -> w1518
          tunnel: w1517 -> [w1532 w1543]
          frame "Down" {
            n692 = case shown="False" w1535 {
              tunnel: w1532 -> [w1538 w1541]
              tunnel: w1534 -> [w1537 w1540]
              tunnel: [w1536 w1539] -> w1533
              frame False {
                n693 = Add(x=w1538, y=w1537) -> (x+y=w1536:dbl)
              }
              frame True {
                n694 = Subtract(x=w1541, y=w1540) -> (x-y=w1539:dbl)
              }
            }
          }
          frame "Up", Default {
            n695 = case shown="False" w1545 {
              tunnel: w1543 -> [w1548 w1551]
              tunnel: w1544 -> [w1547 w1550]
              tunnel: [w1546 w1549] -> w1542
              frame False {
                n696 = Subtract(x=w1548, y=w1547) -> (x-y=w1546:dbl)
              }
              frame True {
                n697 = Add(x=w1551, y=w1550) -> (x+y=w1549:dbl)
              }
            }
          }
        }
        n698 = call <vilib>:"Add State(s) to Queue__jki_lib_state_machine.vi"("State(s) in Front (\"\")"="RestartAveraging" ("State(s) in Front (\"\")"), "State(s) in (\"\")"=w1531) -> ("States Out"=w1530:string)  [unwired: 13 in]
        n699 = call "Beampointing get set motor position.vi"("Active CCD"=w1513, "Set position"=w1518, "get or set"=enum16{"get", "set"}."set", "dev variable alias Motors X"=w1521) -> ("Actual Position"=w1514:dbl)  [unwired: 6 in, 1 out]
        n700 = Unbundle By Name(w1512) -> ("Motor positions.Positions y"=w1516:dbl[])
        n701 = Replace Array Subset(array=w1516, new element=w1514, index=w1513) -> (w1515:dbl[])
        n702 = Bundle By Name(cluster=w1512, "Motor positions.Positions y"=w1515) -> (w1511:T35)
      }
      frame "Move Y" {
        # "Your code here.\n(You can make a copy of, or modify, this frame)"
        n703 = Unbundle By Name(w1563) -> ("dev var alias arrays.dev variable alias Motors Y"=w1564:string[][])
        n704 = Unbundle By Name(w1563) -> ("Offset Y"=w1576:dbl[][])
        n705 = call-poly <userlib>:"Filter 1D Array__ogtk.vi"("items to filter"=w1568, "array"=w1577) -> ("filtered item indices"=w1572:i32[])  [unwired: 4 in, 1 out]
        n706 = Unbundle By Name(w1563) -> ("move properties"=w1570:T11[])
        n707 = for {
          tunnel: w1572 -> [w1603] mode=indexing
          tunnel: w1570 -> [w1607]
          shift-right: [w1602] -> w1571
          shift-left: i32[] [] ("filtered item indices") -> [w1605]
          n708 = Index Array(array=w1607, index=w1603) -> (element=w1606:T11)
          n709 = Unbundle By Name(w1606) -> ("enable feedback"=w1604:bool)
          n710 = case shown="True" w1604 {
            tunnel: w1605 -> [w1608 w1611]
            tunnel: w1603 -> [_ w1610]
            tunnel: [w1608 w1609] -> w1602
            frame False {
            }
            frame True {
              n711 = Build Array (concatenate)(w1611, w1610) -> (w1609:i32[])
            }
          }
        }
        n712 = Index Array(array=w1571) -> (element=w1561:i32)  [unwired: 1 in]
        n713 = Index Array(array=w1576, index (row)=w1561) -> (element=w1575:dbl[])  [unwired: 1 in]
        n714 = Reverse 1D Array(array=w1575) -> (reversed array=w1574:dbl[])
        n715 = call "Beampointing get set motor position.vi"("Active CCD"=w1561, "error in (no error)"=w1557, "get or set"=enum16{"get", "set"}."get", "dev variable alias Motors X"=w1564) -> ("error out"=w1559:errorcluster, "Actual Position"=w1565:dbl)  [unwired: 6 in]
        n716 = Index Array(array=w1574) -> (element=w1556:dbl)  [unwired: 1 in]
        n717 = Index Array(array=w1570, index=w1561) -> (element=w1553:T11)
        n718 = Unbundle By Name(w1553) -> ("enable feedback"=w1573:bool)
        n719 = local read "Align"() -> (w1552:bool)
        n720 = call "relative move from offset and calibration.vi"("Align"=w1552, "axis"=enum16{"x", "y"}."y", "Offset"=w1556, "element"=w1553) -> ("relative move out"=w1555:dbl)  [unwired: 7 in]
        n721 = case shown="No Error" w1559 {
          selector: w1559 -> [_ w1600]
          tunnel: w1573 -> [w1590 _]
          tunnel: w1565 -> [w1589 _]
          tunnel: w1564 -> [w1588 _]
          tunnel: w1563 -> [w1585 w1601]
          tunnel: [w1584 w1601] -> w1562
          tunnel: w1561 -> [w1582 _]
          tunnel: w1555 -> [w1581 _]
          tunnel: [w1580 w1600] -> w1558
          frame No Error {
            n722 = case shown="True" w1590 {
              tunnel: w1581 -> [_ w1599]
              tunnel: w1589 -> [w1591 w1598]
              tunnel: w1588 -> [_ w1595]
              tunnel: w1582 -> [_ w1594]
              tunnel: [w1591 w1593] -> w1583
              tunnel: [_ w1592] -> w1580
              frame False {
              }
              frame True {
                n723 = Add(x=w1598, y=w1599) -> (x+y=w1597:dbl)
                n724 = call "Beampointing get set motor position.vi"("Active CCD"=w1594, "Set position"=w1597, "get or set"=enum16{"get", "set"}."set", "dev variable alias Motors X"=w1595) -> ("error out"=w1592:errorcluster, "Actual Position"=w1593:dbl)  [unwired: 6 in]
              }
            }
            n725 = Unbundle By Name(w1585) -> ("Motor positions.Positions y"=w1587:dbl[])
            n726 = Replace Array Subset(array=w1587, new element=w1583, index=w1582) -> (w1586:dbl[])
            n727 = Bundle By Name(cluster=w1585, "Motor positions.Positions y"=w1586) -> (w1584:T35)
          }
          frame Error {
          }
        }
        n728 = call <vilib>:"Build State String with Arguments__jki_lib_state_machine.vi"("Arguments (\"\")"=w1568, "State"="Wait" ("State(s) in Front (\"\")")) -> ()  [unwired: 4 in, 1 out]
        n729 = call <vilib>:"Add State(s) to Queue__jki_lib_state_machine.vi"("State(s) in (\"\")"=w1579) -> ("States Out"=w1578:string)  [unwired: 14 in]
        "Moving Y" <- w1568
      }
      frame "Wait" {
        # "Your code here.\n(You can make a copy of, or modify, this frame)"
        n730 = disable-structure shown="Disabled" {
          disable-tunnel: w1617 -> [w1631 _]
          disable-tunnel: w1616 -> [w1630 _]
          disable-tunnel: w1615 -> [w1629 _]
          disable-tunnel: w1614 -> [w1627 w1651]
          disable-tunnel: [w1626 w1651] -> w1613
          frame Disabled {
            n731 = call-poly <userlib>:"Filter 1D Array__ogtk.vi"("items to filter"=w1629, "array"=w1630) -> ("filtered item indices"=w1628:i32[])  [unwired: 4 in, 1 out]
            n732 = flat-sequence {
              tunnel: T30."Disabled and Grayed Out" ("Disabled") -> [w1632]
              tunnel: w1627 -> [w1640]
              tunnel: [w1639] -> w1626
              tunnel: w1625 -> [w1638]
              tunnel: w1624 -> [w1637]
              tunnel: T30."Enabled" ("Disabled") -> [w1650]
              frame #0 {
                n733 = property on="Right" class="Bool (strict)"("DisabledEnum"=w1632) -> ()  [unwired: 2 in, 2 out]
                n734 = property on="Up" class="Bool (strict)"("DisabledEnum"=w1632) -> ()  [unwired: 2 in, 2 out]
                n735 = property on="Left" class="Bool (strict)"("DisabledEnum"=w1632) -> ()  [unwired: 2 in, 2 out]
                n736 = property on="Down" class="Bool (strict)"("DisabledEnum"=w1632) -> ()  [unwired: 2 in, 2 out]
                n737 = property on="StepSize" class="DigNum (strict)"("DisabledEnum"=w1632) -> ()  [unwired: 2 in, 2 out]
              }
              frame #1 {
                n738 = Wait (ms)(milliseconds to wait=u32 1500) -> ()  [unwired: 1 out]
              }
              frame #2 {
                n739 = property on="Moving Y" class="Str"("Value"="") -> ()  [unwired: 2 in, 2 out]
                n740 = property on="Moving X" class="Str"("Value"="") -> ()  [unwired: 2 in, 2 out]
              }
              frame #3 {
                n741 = Equal?(x=w1637, y=w1638) -> (x = y?=w1636:bool)
                n742 = case shown="True" w1636 {
                  tunnel: _ -> [_ w1647]
                  tunnel: w1640 -> [w1641 w1644]
                  tunnel: [w1641 w1642] -> w1639
                  frame False {
                  }
                  frame True {
                    n743 = Unbundle By Name(w1647) -> ("Ref X"=w1646, "Ref Y"=w1645)
                    n744 = property class="DigNum (strict)"(reference=w1646, error in=w1644) -> (error out=w1643:errorcluster, "Value"=w1649:dbl)  [unwired: 1 out]
                    n745 = property class="DigNum (strict)"(reference=w1645, error in=w1643) -> (error out=w1642:errorcluster, "Value"=w1648:dbl)  [unwired: 1 out]
                    n746 = property on="Position 1" class="DigNum (strict)"("Value"=w1649) -> ()  [unwired: 2 in, 2 out]
                    n747 = property on="Position 2" class="DigNum (strict)"("Value"=w1648) -> ()  [unwired: 2 in, 2 out]
                  }
                }
              }
              frame #4 {
                n748 = property on="Right" class="Bool (strict)"("DisabledEnum"=w1650) -> ()  [unwired: 2 in, 2 out]
                n749 = property on="Up" class="Bool (strict)"("DisabledEnum"=w1650) -> ()  [unwired: 2 in, 2 out]
                n750 = property on="Left" class="Bool (strict)"("DisabledEnum"=w1650) -> ()  [unwired: 2 in, 2 out]
                n751 = property on="Down" class="Bool (strict)"("DisabledEnum"=w1650) -> ()  [unwired: 2 in, 2 out]
                n752 = property on="StepSize" class="DigNum (strict)"("DisabledEnum"=w1650) -> ()  [unwired: 2 in, 2 out]
              }
            }
            n753 = Index Array(array=w1628) -> (element=w1625:i32)  [unwired: 1 in]
            n754 = Unbundle By Name(w1631) -> ("active ccd"=w1624:i32)
          }
          frame Enabled {
          }
        }
        n755 = call <vilib>:"Add State(s) to Queue__jki_lib_state_machine.vi"("State(s) in (\"\")"=w1621) -> ("States Out"=w1620:string)  [unwired: 14 in]
        n756 = local read "Mean Centroid X"() -> (w1618:dbl[][])
        n757 = Bundle By Name(cluster=w1617, "Mean Centroid X"=w1618, "Mean Centroid Y"=w1618) -> (w1619:T35)
      }
      frame "RestartAveraging" {
        # "clear arrays"
        n758 = Unbundle By Name(w1658) -> ("Detection"=w1659:T32)
        n759 = Unbundle By Name(w1659) -> ("img to avg"=w1661:i32)
        n760 = Decrement(x=w1661) -> (x-1=w1656:i32)
        n761 = Initialize Array(0.0 ("element"), 12 ("dimension size"), w1656) -> (w1653:dbl[][])
        n762 = Bundle By Name(cluster=w1659, "Centroid X"=w1653, "Centroid Y"=w1653, "Size"=w1653) -> (w1660:T32)
        n763 = Bundle By Name(cluster=w1658, "Detection"=w1660) -> (w1657:T35)
        n764 = local write "#imgs avd so far"(0.0 ("#imgs avd so far")) -> ()
        n765 = call <vilib>:"Add State(s) to Queue__jki_lib_state_machine.vi"("State(s) in (\"\")"=w1665) -> ("States Out"=w1664:string)  [unwired: 14 in]
      }
      frame "---------------Statistics--------------" {
        # "Template Separator\n(You can make a copy of, or modify, this frame)"
        n766 = call <vilib>:"Add State(s) to Queue__jki_lib_state_machine.vi"("State(s) in (\"\")"=w1670) -> ("States Out"=w1669:string)  [unwired: 14 in]
      }
      frame "Save Stats" {
        # "Your code here.\n(You can make a copy of, or modify, this frame)"
        n767 = disable-structure shown="Disabled" {
          disable-tunnel: w1677 -> [w1681 _]
          disable-tunnel: [w1680 _] -> w1676
          disable-tunnel: _ -> [w1679 _]
          disable-tunnel: w1673 -> [w1678 _]
          frame Disabled {
            n768 = for {
              tunnel: w1679 -> [w1684] mode=indexing
              tunnel: w1678 -> [w1683] mode=indexing
              n769 = Empty String/Path?(string/path=w1683) -> (empty?=w1682:bool)
              n770 = case shown="False" w1682 {
                tunnel: w1684 -> [w1690 _]
                tunnel: w1683 -> [w1688 _]
                frame False {
                  n771 = Index Array(array=w1690, index #1=0 ("index"), index #2=1 ("index"), index #3=2 ("index"), index #4=3 ("index")) -> (element #1=w1725, element #2=w1719, element #3=w1718, element #4=w1717)  [unwired: 1 in, 1 out]
                  n772 = Concatenate Strings(w1688, ".dat" ("string")) -> (w1686:string)
                  n773 = Unbundle(w1725) -> (w1724, w1702)
                  n774 = Unbundle(w1719) -> (w1693)  [unwired: 1 out]
                  n775 = Unbundle(w1718) -> (w1692)  [unwired: 1 out]
                  n776 = Unbundle(w1717) -> (w1691)  [unwired: 1 out]
                  n777 = Build Path(base path="save path", name or relative path=w1686) -> (appended path=w1685:path)
                  n778 = for {
                    tunnel: w1724 -> [w1727]
                    tunnel: [w1726] -> w1700 mode=indexing
                    n779 = Format Date/Time String(time format string (%c)="%Y%m%d%H%M%S", seconds (now)=w1727) -> (date/time string=w1726:string)  [unwired: 1 in]
                  }
                  n780 = Array Size(array=w1702) -> (size(s)=w1703:i32)
                  n781 = Number To Fractional String(number=w1702) -> (F-format string=w1699:string)  [unwired: 3 in]
                  n782 = Number To Fractional String(number=w1693) -> (F-format string=w1696:string)  [unwired: 3 in]
                  n783 = Number To Fractional String(number=w1692) -> (F-format string=w1695:string)  [unwired: 3 in]
                  n784 = Number To Fractional String(number=w1691) -> (F-format string=w1694:string)  [unwired: 3 in]
                  n785 = Initialize Array("", w1703, 5 ("dimension size")) -> (w1701:string[][])
                  n786 = Insert Into Array(array=w1701, index (col)=0 ("disabled index (col)"), new element=w1700) -> (w1711:string[][])  [unwired: 1 in]
                  n787 = Insert Into Array(array=w1711, index (col)=1 ("disabled index (col)"), new element=w1699) -> (w1710:string[][])  [unwired: 1 in]
                  n788 = Insert Into Array(array=w1710, index (col)=2 ("disabled index (col)"), new element=w1696) -> (w1714:string[][])  [unwired: 1 in]
                  n789 = Insert Into Array(array=w1714, index (col)=3 ("disabled index (col)"), new element=w1695) -> (w1715:string[][])  [unwired: 1 in]
                  n790 = Insert Into Array(array=w1715, index (col)=4 ("disabled index (col)"), new element=w1694) -> (w1716:string[][])  [unwired: 1 in]
                  n791 = Insert Into Array(array=w1716, index (row)=0, new element=string[] ["time", "Centroid X", "Centroid Y", "Motor Axis 1", "Motor Axis 2"] ("new element/subarray 2")) -> (w1698:string[][])  [unwired: 1 in]
                  n792 = call-poly <vilib>:"Write To Spreadsheet File.vi"("2D data"=w1698, "file path (dialog if empty)"=w1685) -> ()  [unwired: 6 in, 1 out]
                }
                frame True {
                }
              }
            }
            n793 = call <vilib>:"Add State(s) to Queue__jki_lib_state_machine.vi"("State(s) in (\"\")"=w1681) -> ("States Out"=w1680:string)  [unwired: 14 in]
          }
          frame Enabled {
          }
        }
        n794 = property on="Save Stats" class="Bool (strict)"("Value"=FALSE ("Save Stats")) -> ()  [unwired: 2 in, 2 out]
      }
      frame "tdms" {
        w1742 = 21600.0 ("new tdms")
        # "Your code here.\n(You can make a copy of, or modify, this frame)"
        n795 = Unbundle By Name(w1749) -> ("active cams"=w1735:string[], "tdms ref"=w1732:refnum<k34>, "Offset X"=w1748:dbl[][], "Offset Y"=w1747:dbl[][], "Motor positions.Positions x"=w1730:dbl[], "Motor positions.Positions y"=w1729:dbl[])
        n796 = for {
          tunnel: w1748 -> [w1792]
          tunnel: w1747 -> [w1791]
          tunnel: w1735 -> [w1764] mode=indexing
          tunnel: w1732 -> [w1765]
          tunnel: w1751 -> [w1759]
          tunnel: [w1768] -> w1750
          tunnel: w1730 -> [w1758]
          tunnel: w1729 -> [w1756]
          i -> [w1755]
          n797 = Index Array(array=w1792, index (row)=w1755) -> (element=w1790:dbl[])  [unwired: 1 in]
          n798 = Index Array(array=w1791, index (row)=w1755) -> (element=w1789:dbl[])  [unwired: 1 in]
          n799 = Reverse 1D Array(array=w1789) -> (reversed array=w1787:dbl[])
          n800 = Reverse 1D Array(array=w1790) -> (reversed array=w1788:dbl[])
          n801 = Index Array(array=w1788) -> (element=w1786:dbl)  [unwired: 1 in]
          n802 = Index Array(array=w1787) -> (element=w1785:dbl)  [unwired: 1 in]
          n803 = Index Array(array=w1756, index=w1755) -> (element=w1754:dbl)
          n804 = Index Array(array=w1758, index=w1755) -> (element=w1757:dbl)
          n805 = Build Array(w1786) -> (w1767:dbl[])
          n806 = Build Array(w1785) -> (w1780:dbl[])
          n807 = Get Date/Time In Seconds() -> (seconds since 1Jan1904=w1766:timestamp)
          n808 = Build Array(w1766) -> (w1762:timestamp[])
          n809 = Build Array(w1757) -> (w1774:dbl[])
          n810 = TDMS Write(0:w1765, 5:w1764, 7:"time", 9:w1762, 11:w1759) -> (4:w1761:refnum<k34>, 15:w1760:errorcluster)  [unwired: 1 in, 2 out]
          n811 = Build Array(w1754) -> (w1769:dbl[])
          n812 = TDMS Write(0:w1761, 5:w1764, 7:"centroid X", 9:w1767, 11:w1760) -> (4:w1783:refnum<k34>, 6:w1782:string, 15:w1781:errorcluster)  [unwired: 1 in, 1 out]
          n813 = TDMS Write(0:w1783, 5:w1782, 7:"centroid Y", 9:w1780, 11:w1781) -> (4:w1777:refnum<k34>, 6:w1776:string, 15:w1778:errorcluster)  [unwired: 1 in, 1 out]
          n814 = TDMS Write(0:w1777, 5:w1776, 7:"Motor Axis 1", 9:w1774, 11:w1778) -> (4:w1773:refnum<k34>, 6:w1772:string, 15:w1770:errorcluster)  [unwired: 1 in, 1 out]
          n815 = TDMS Write(0:w1773, 5:w1772, 7:"Motor Axis 2", 9:w1769, 11:w1770) -> (15:w1768:errorcluster)  [unwired: 1 in, 3 out]
        }
        n816 = property on="millisecond timer value" class="DigNum (strict)"() -> ("Value"=w1734:u32)  [unwired: 2 in, 2 out]
        n817 = Tick Count (ms)() -> (millisecond timer value=w1733:u32)
        n818 = Unbundle By Name(w1749) -> ()  [unwired: 1 out]
        n819 = Subtract(x=w1733, y=w1734) -> (x-y=w1737:u32)
        n820 = Divide(x=w1737, y=u32 1000) -> (x/y=w1739:dbl)
        n821 = Quotient & Remainder(x=w1739, y=w1742) -> (x-y*floor(x/y)=w1740:dbl)  [unwired: 1 out]
        n822 = Subtract(x=w1742, y=20.0) -> (x-y=w1744:dbl)
        n823 = Greater?(x=w1740, y=w1744) -> (0:w1741:bool)
        n824 = Select(t="newtdms", s=w1741, f="") -> (s? t:f=w1736:string)
        n825 = call <vilib>:"Add State(s) to Queue__jki_lib_state_machine.vi"("State(s) in (\"\")"=w1753, "State(s) at Back (\"\")"=w1736) -> ("States Out"=w1752:string)  [unwired: 13 in]
      }
      frame "Reset History" {
        # "Your code here.\n(You can make a copy of, or modify, this frame)"
        n826 = for {
          N: 1 -> [_]
          shift-right: [w1803] -> w1795
          shift-left: timestamp[][] [] ("Time") -> [w1805]
          n827 = for {
            N: 12 -> [_]
            tunnel: w1805 -> [w1808] mode=indexing
            tunnel: [w1806] -> w1803 mode=indexing
            n828 = Get Date/Time In Seconds() -> (seconds since 1Jan1904=w1807:timestamp)
            n829 = Build Array (concatenate)(w1808, w1807) -> (w1806:timestamp[])
          }
        }
        n830 = local read "Offset X"() -> (w1794:dbl[][])
        n831 = Bundle By Name(cluster=w1799, "Offset X"=w1794, "Offset Y"=w1794, "Time"=w1795, "Motor X"=w1794) -> (w1798:T35)
        n832 = call <vilib>:"Add State(s) to Queue__jki_lib_state_machine.vi"("State(s) in (\"\")"=w1802) -> ("States Out"=w1801:string)  [unwired: 14 in]
      }
      frame "New Category: 2" {
        n833 = call <vilib>:"Add State(s) to Queue__jki_lib_state_machine.vi"("State(s) in (\"\")"=w1813) -> ("States Out"=w1812:string)  [unwired: 14 in]
      }
      frame "perpective read" {
        n834 = call <vilib>:"Add State(s) to Queue__jki_lib_state_machine.vi"("State(s) in (\"\")"=w1818) -> ("States Out"=w1817:string)  [unwired: 14 in]
      }
      frame "stats" {
        # "Your code here.\n(You can make a copy of, or modify, this frame)"
        n835 = Unbundle By Name(w1834) -> ("Offset X"=w1825:dbl[][], "Offset Y"=w1824:dbl[][], "Time"=w1823:timestamp[][], "Motor X"=w1822:dbl[][], "Motor Y"=w1821:dbl[][], "tdms ref"=w1829:refnum<k34>)
        n836 = TDMS List Contents(4:w1828, 7:w1829) -> (0:w1820:errorcluster, 2:w1832:string[], 3:w1831:refnum<k34>)  [unwired: 1 in, 1 out]
        n837 = call <vilib>:"ClearError.vi"("error in (no error)"=w1820) -> ("error out"=w1830:errorcluster)
        n838 = for {
          tunnel: w1830 -> [w1879]
          tunnel: [w1865] -> w1826 mode=indexing
          tunnel: [w1864] -> w1827
          tunnel: [w1863] -> _
          tunnel: w1831 -> [w1862]
          tunnel: w1832 -> [w1861] mode=indexing
          w1880 = dbl[] [] ("appended array")
          n839 = TDMS Read(0:w1862, 5:w1861, 7:"time", 11:w1879, 12:timestamp[] [] ("appended array")) -> (4:w1894:refnum<k34>, 6:w1890:string, 10:w1871:timestamp[], 15:w1878:errorcluster)  [unwired: 3 in, 2 out]
          n840 = TDMS Read(0:w1894, 5:w1890, 7:"centroid X", 11:w1878, 12:w1880) -> (4:w1893:refnum<k34>, 6:w1889:string, 10:w1874:dbl[], 15:w1877:errorcluster)  [unwired: 3 in, 2 out]
          n841 = TDMS Read(0:w1893, 5:w1889, 7:"centroid Y", 11:w1877, 12:w1880) -> (4:w1892:refnum<k34>, 6:w1888:string, 10:w1873:dbl[], 15:w1876:errorcluster)  [unwired: 3 in, 2 out]
          n842 = TDMS Read(0:w1892, 5:w1888, 7:"Motor Axis 1", 11:w1876, 12:w1880) -> (4:w1891:refnum<k34>, 6:w1887:string, 10:w1872:dbl[], 15:w1875:errorcluster)  [unwired: 3 in, 2 out]
          n843 = TDMS Read(0:w1891, 5:w1887, 7:"Motor Axis 2", 11:w1875, 12:w1880) -> (4:w1863:refnum<k34>, 10:w1870:dbl[], 15:w1864:errorcluster)  [unwired: 3 in, 3 out]
          n844 = Bundle("appended array"=w1871, "appended array"=w1874) -> (w1869:T56)  [unwired: 1 in]
          n845 = Bundle("appended array"=w1871, "appended array"=w1873) -> (w1868:T56)  [unwired: 1 in]
          n846 = Bundle("appended array"=w1871, "appended array"=w1872) -> (w1867:T56)  [unwired: 1 in]
          n847 = Bundle("appended array"=w1871, "appended array"=w1870) -> (w1866:T56)  [unwired: 1 in]
          n848 = Build Array(w1869, w1868, w1867, w1866) -> (w1865:T57)
        }
        n849 = disable-structure shown="Disabled" {
          disable-tunnel: w1833 -> [w1844 _]
          disable-tunnel: w1825 -> [w1843 _]
          disable-tunnel: w1824 -> [w1842 _]
          disable-tunnel: w1823 -> [w1841 _]
          disable-tunnel: w1822 -> [w1840 _]
          disable-tunnel: w1821 -> [w1839 _]
          frame Disabled {
            n850 = for {
              tunnel: w1844 -> [_] mode=indexing
              tunnel: w1843 -> [w1854]
              tunnel: w1842 -> [w1853]
              tunnel: w1841 -> [w1852]
              tunnel: w1840 -> [w1848]
              tunnel: w1839 -> [w1847]
              tunnel: [w1856] -> _ mode=indexing
              i -> [w1855]
              n851 = Index Array(array=w1853, index (row)=w1855) -> (element=w1849:dbl[])  [unwired: 1 in]
              n852 = Index Array(array=w1848, index (row)=w1855) -> (element=w1846:dbl[])  [unwired: 1 in]
              n853 = Index Array(array=w1847, index (row)=w1855) -> (element=w1845:dbl[])  [unwired: 1 in]
              n854 = Index Array(array=w1854, index (row)=w1855) -> (element=w1850:dbl[])  [unwired: 1 in]
              n855 = Index Array(array=w1852, index (row)=w1855) -> (element=w1851:timestamp[])  [unwired: 1 in]
              n856 = Bundle("Time"=w1851, "Motor X"=w1846) -> (w1859:cluster{"Time":timestamp[], "Motor X":dbl[]})  [unwired: 1 in]
              n857 = Bundle("Time"=w1851, "Motor Y"=w1845) -> (w1860:cluster{"Time":timestamp[], "Motor Y":dbl[]})  [unwired: 1 in]
              n858 = Bundle("Time"=w1851, "Offset X"=w1850) -> (w1858:cluster{"Time":timestamp[], "Offset X":dbl[]})  [unwired: 1 in]
              n859 = Bundle("Time"=w1851, "Offset Y"=w1849) -> (w1857:cluster{"Time":timestamp[], "Offset Y":dbl[]})  [unwired: 1 in]
              n860 = Build Array(w1857, w1858, w1859, w1860) -> (w1856:cluster{"Time":timestamp[], "Motor Y":dbl[]}[])
            }
          }
          frame Enabled {
          }
        }
        n861 = Index Array(array=w1826, index (row)="Cam# history") -> (element=→"CCD 1":T57)  [unwired: 1 in]
        n862 = call <vilib>:"Add State(s) to Queue__jki_lib_state_machine.vi"("State(s) in (\"\")"=w1838) -> ("States Out"=w1837:string)  [unwired: 14 in]
      }
      frame "newtdms" {
        n863 = Unbundle By Name(w1933) -> ("tdms ref"=w1926:refnum<k34>, "active cams"=w1921:string[])
        n864 = Empty String/Path?(string/path="tdms root") -> (empty?=w1898:bool)
        n865 = Select(t=path "c:/BeamPointing" ("tdms root"), s=w1898, f="tdms root") -> (s? t:f=w1895:path)
        n866 = TDMS Close(8:w1931, 11:w1926) -> (0:w1920:errorcluster)  [unwired: 1 out]
        n867 = local read "config path"() -> (w1902:string)
        n868 = call <vilib>:"Clear Errors.vi"("error in (no error)"=w1920) -> ("error out"=w1909:errorcluster)  [unwired: 5 in, 1 out]
        n869 = Get Date/Time In Seconds() -> (seconds since 1Jan1904=w1914:timestamp)
        n870 = call-poly <userlib>:"Strip Path Extension__ogtk.vi"("path"=w1902) -> ("root"=w1901:string)  [unwired: 1 out]
        n871 = property on="new tdms" class="Bool (strict)"("Value"=FALSE ("new tdms")) -> ()  [unwired: 2 in, 2 out]
        n872 = Format Date/Time String(time format string (%c)="%Y%m%d", seconds (now)=w1914) -> (date/time string=w1915:string)  [unwired: 1 in]
        n873 = Format Date/Time String(time format string (%c)="%Y%m%d%H%M", seconds (now)=w1914) -> (date/time string=w1912:string)  [unwired: 1 in]
        n874 = String To Path(string=w1901) -> (path=w1900:path)
        n875 = Strip Path(path=w1900) -> (name=w1899:string)  [unwired: 1 out]
        n876 = Build Path(base path=w1895, name or relative path=w1915) -> (appended path=w1916:path)
        n877 = Concatenate Strings(w1912, w1899, ".tdms" ("string")) -> (w1911:string)
        n878 = String To Path(string=w1911) -> (path=w1907:path)
        n879 = call <vilib>:"Check if File or Folder Exists.vi"("error in (no error)"=w1909, "path"=w1916) -> ("error out"=w1919:errorcluster, "file or folder exists?"=w1917:bool, "dup path"=w1918:path)  [unwired: 7 in]
        n880 = case shown="False" w1917 {
          tunnel: w1918 -> [w1939 w1941]
          tunnel: [w1938 w1941] -> w1906
          tunnel: w1919 -> [w1937 w1940]
          tunnel: [w1936 w1940] -> w1908
          frame False {
            n881 = Create Folder(path (use dialog)=w1939, error in=w1937) -> (created path=w1938:path, error out=w1936:errorcluster)  [unwired: 1 in, 1 out]
          }
          frame True {
          }
        }
        n882 = call <vilib>:"Add State(s) to Queue__jki_lib_state_machine.vi"("State(s) in (\"\")"=w1935) -> ("States Out"=w1934:string)  [unwired: 14 in]
        n883 = Build Path(base path=w1906, name or relative path=w1907) -> (appended path=w1927:path)
        n884 = TDMS Open(6:FALSE ("disable buffering (T)"), 7:enum16{"1.0", "2.0"}."2.0" ("file format version (2.0)"), 8:w1908, 10:T31."create or replace" ("operation"), 11:w1927) -> (0:w1924:errorcluster, 3:w1923:refnum<k34>)  [unwired: 2 in]
        n885 = call "TDMSbuffersize.vi"("error in (no error)"=w1924, "group names"=w1921, "Data Value Reference in"=w1923) -> ("error out"=w1904:errorcluster, "Data Value Reference out"=w1922:refnum<k34>)  [unwired: 7 in]
        n886 = Bundle By Name(cluster=w1933, "tdms ref"=w1922) -> (w1932:T35)
      }
      frame "Center" {
        # "Your code here.\n(You can make a copy of, or modify, this frame)"
        n887 = control-ref of="Display1"() -> (w1957:refnum<vi>)
        n888 = control-ref of="Display2"() -> (w1956:refnum<vi>)
        n889 = control-ref of="Display3"() -> (w1955:refnum<vi>)
        n890 = control-ref of="Display4"() -> (w1954:refnum<vi>)
        n891 = control-ref of="Display5"() -> (w1953:refnum<vi>)
        n892 = control-ref of="Display6"() -> (w1952:refnum<vi>)
        n893 = control-ref of="Display7"() -> (w1951:refnum<vi>)
        n894 = control-ref of="Dsiplay8"() -> (w1950:refnum<vi>)
        n895 = control-ref of="Display9"() -> (w1949:refnum<vi>)
        n896 = control-ref of="Display10"() -> (w1948:refnum<vi>)
        n897 = control-ref of="Display11"() -> (w1947:refnum<vi>)
        n898 = control-ref of="Display12"() -> (w1946:refnum<vi>)
        n899 = for {
          tunnel: [w1966] -> w1945 mode=indexing
          tunnel: w1944 -> [w1965] mode=indexing
          n900 = Unbundle By Name(w1965) -> ("Target.X::12"=w1964:refnum<vi>, "Target.Y::12"=w1963:refnum<vi>)
          n901 = property class="DigNum (strict)"(reference=w1964) -> ("Value"=w1967:dbl)  [unwired: 1 in, 2 out]
          n902 = property class="DigNum (strict)"(reference=w1963) -> ("Value"=w1968:dbl)  [unwired: 1 in, 2 out]
          n903 = Bundle("Value"=w1967, "Value"=w1968) -> (w1966:cluster{"Value":dbl, "Value":dbl})  [unwired: 1 in]
        }
        n904 = call <vilib>:"Add State(s) to Queue__jki_lib_state_machine.vi"("State(s) in (\"\")"=w1962) -> ("States Out"=w1961:string)  [unwired: 14 in]
        n905 = Build Array(w1957, w1956, w1955, w1954, w1953, w1952, w1951, w1950, w1949, w1948, w1947, w1946) -> (w1958:refnum<vi>[])
        n906 = for {
          tunnel: w1958 -> [w1970] mode=indexing
          tunnel: w1945 -> [w1969] mode=indexing
          n907 = property class="ImageControl"(reference=w1970, "Image Center Position"=w1969) -> ()  [unwired: 1 in, 2 out]
        }
        n908 = property on="Center" class="Bool (strict)"("Value"=FALSE ("Center")) -> ()  [unwired: 2 in, 2 out]
      }
      frame "ImgToAvg" {
        n909 = Bundle By Name(cluster=w1980, "Detection.img to avg"="img to avg") -> (w1979:T35)
        n910 = call <vilib>:"Build State String with Arguments__jki_lib_state_machine.vi"("Arguments (\"\")"="T" ("Arguments (\"\")"), "State"=" Device Ini") -> ("State with Arguments"=w1973:string)  [unwired: 4 in]
        n911 = call <vilib>:"Add State(s) to Queue__jki_lib_state_machine.vi"("State(s) in Front (\"\")"=w1973, "State(s) in (\"\")"=w1978) -> ("States Out"=w1977:string)  [unwired: 13 in]
      }
      frame "history" {
        # "Your code here.\n(You can make a copy of, or modify, this frame)"
        n912 = Unbundle By Name(w1991) -> ("Offset X"=w1997:dbl[][], "Offset Y"=w1996:dbl[][], "Mean Centroid X"=w1995:dbl[][], "Mean Centroid Y"=w1994:dbl[][], "Motor X"=w1993:dbl[][], "Motor Y"=w1992:dbl[][], "Time"=w1983:timestamp[][])
        n913 = for {
          tunnel: w1997 -> [w2015] mode=indexing
          tunnel: w1996 -> [w2013] mode=indexing
          tunnel: w1995 -> [w2012] mode=indexing
          tunnel: w1994 -> [w2011] mode=indexing
          tunnel: w1993 -> [w2010] mode=indexing
          tunnel: w1992 -> [w2009] mode=indexing
          tunnel: [w2014] -> w1989 mode=indexing
          tunnel: [w2008] -> w1988 mode=indexing
          tunnel: [w2004] -> w1987 mode=indexing
          tunnel: [w2007] -> w1986 mode=indexing
          tunnel: [w2006] -> w1985 mode=indexing
          tunnel: [w2005] -> w1984 mode=indexing
          tunnel: w1983 -> [w2003] mode=indexing
          tunnel: [w2001] -> w1982 mode=indexing
          w2002 = 0
          n914 = Delete From Array(array=w2010, index=w2002) -> (array with subset deleted=w2006:dbl[])  [unwired: 1 in, 1 out]
          n915 = Delete From Array(array=w2009, index=w2002) -> (array with subset deleted=w2005:dbl[])  [unwired: 1 in, 1 out]
          n916 = Delete From Array(array=w2003, index=w2002) -> (array with subset deleted=w2001:timestamp[])  [unwired: 1 in, 1 out]
          n917 = Delete From Array(array=w2012, index=w2002) -> (array with subset deleted=w2004:dbl[])  [unwired: 1 in, 1 out]
          n918 = Delete From Array(array=w2011, index=w2002) -> (array with subset deleted=w2007:dbl[])  [unwired: 1 in, 1 out]
          n919 = Delete From Array(array=w2013, index=w2002) -> (array with subset deleted=w2008:dbl[])  [unwired: 1 in, 1 out]
          n920 = Delete From Array(array=w2015, index=w2002) -> (array with subset deleted=w2014:dbl[])  [unwired: 1 in, 1 out]
        }
        n921 = call <vilib>:"Add State(s) to Queue__jki_lib_state_machine.vi"("State(s) in (\"\")"=w2000) -> ("States Out"=w1999:string)  [unwired: 14 in]
        n922 = Bundle By Name(cluster=w1991, "Offset X"=w1989, "Offset Y"=w1988, "Mean Centroid X"=w1987, "Mean Centroid Y"=w1986, "Motor X"=w1985, "Motor Y"=w1984, "Time"=w1982) -> (w1990:T35)
      }
    }
    "Prev State" <- w49
    n923 = property on="Box" class="Arr (strict)"() -> ("Value"=w57:T3)  [unwired: 2 in, 2 out]
    n924 = for {
      tunnel: w58 -> [w104]
      tunnel: w51 -> [w112]
      tunnel: w55 -> [w70] mode=indexing
      tunnel: w57 -> [w72] mode=indexing
      tunnel: w54 -> [w102]
      tunnel: w53 -> [w101]
      tunnel: w52 -> [w83]
      i -> [w82]
      w97 = T58 {"Draw"=TRUE, "Target"={"x"=20.0, "y"=20.0}, "Size"={"x"=20.0, "y"=20.0}, "Angle"=1250067.0, "Color"=1250067, "Thickness"=0, "CrosshairLabel"=""} ("Crosshair")
      w91 = T59 {"Left"=0, "Top"=0, "Right"=0, "Bottom"=0} ("Bounding Rectangle")
      n925 = call-poly <userlib>:"Filter 1D Array__ogtk.vi"("items to filter"=w70, "array"=w112) -> ("filtered item indices"=w113:i32[])  [unwired: 4 in, 1 out]
      n926 = Index Array(array=w113) -> (element=w103:i32)  [unwired: 1 in]
      n927 = Index Array(array=w83, index (row)=w82) -> (element=w80:dbl[])  [unwired: 1 in]
      n928 = Index Array(array=w102, index (row)=w82) -> (element=w90:dbl[])  [unwired: 1 in]
      n929 = Index Array(array=w104, index=w103) -> (element=w111:T20)
      n930 = Index Array(array=w101, index (row)=w82) -> (element=w88:dbl[])  [unwired: 1 in]
      n931 = Reverse 1D Array(array=w80) -> (reversed array=w79:dbl[])
      n932 = Unbundle By Name(w111) -> ("Target.X::12"=w115:refnum<vi>, "Target.Y::12"=w114:refnum<vi>)
      n933 = Reverse 1D Array(array=w90) -> (reversed array=w89:dbl[])
      n934 = Reverse 1D Array(array=w88) -> (reversed array=w87:dbl[])
      n935 = Index Array(array=w79) -> (element=w77:dbl)  [unwired: 1 in]
      n936 = Concatenate Strings(w70, "_proc" ("string")) -> (w68:string)
      n937 = Square Root(x=w77) -> (sqrt(x)=w76:dbl)
      n938 = Index Array(array=w87) -> (element=w84:dbl)  [unwired: 1 in]
      n939 = Index Array(array=w89) -> (element=w85:dbl)  [unwired: 1 in]
      n940 = Divide(x=w76, y=2.0) -> (x/y=w74:dbl)
      n941 = property class="DigNum (strict)"(reference=w115) -> ("Value"=w108:dbl)  [unwired: 1 in, 2 out]
      n942 = property class="DigNum (strict)"(reference=w114) -> ("Value"=w107:dbl)  [unwired: 1 in, 2 out]
      n943 = Bundle(cluster=cluster{"xhair size":dbl, "xhair size 2":dbl} {"xhair size"=25.0, "xhair size 2"=25.0} ("size"), "xhair size"=w74, "xhair size 2"=w74) -> (w78:cluster{"xhair size":dbl, "xhair size 2":dbl})
      n944 = Bundle By Name(cluster=w97, "Draw"=TRUE, "Target.x"=w108, "Target.y"=w107, "Size"=w78, "Color"=u32 16774656, "Angle"=0.0, "Thickness"=u8 1) -> (w110:T58)
      n945 = call "draw crosshair imaq.vi"("clear overlay"=TRUE, "Crosshair"=w110, "Bounding Rectangle"=w91, "image in"=w68) -> ("error out"=w94:errorcluster, "image out"=w93:T1)  [unwired: 6 in]
      n946 = Bundle By Name(cluster=w97, "Draw"=TRUE, "Target.x"=w85, "Target.y"=w84, "Size"=w78, "Color"=u32 8322834, "Angle"=0.0, "Thickness"=u8 1) -> (w95:T58)
      n947 = case shown="False" "average centroid" {
        tunnel: w95 -> [_ w120]
        tunnel: w94 -> [_ w125]
        tunnel: w93 -> [w117 w124]
        tunnel: w91 -> [_ w123]
        tunnel: w72 -> [w118 _]
        tunnel: [w116 w122] -> w71
        frame False {
          n948 = call "draw box imaq.vi"("Color"=u32 1244928, "Rectangle"=w118, "image in"=w117) -> ("error out"=w116:errorcluster)  [unwired: 7 in, 1 out]
        }
        frame True {
          n949 = call "draw crosshair imaq.vi"("clear overlay"=FALSE, "error in (no error)"=w125, "Crosshair"=w120, "Bounding Rectangle"=w123, "image in"=w124) -> ("error out"=w122:errorcluster)  [unwired: 5 in, 1 out]
        }
      }
      "error out 3" <- w71
    }
  }
  n950 = call <userlib>:"Fit VI window to Largest Dec__ogtk.vi"() -> ()  [unwired: 6 in, 2 out]
  n951 = disable-structure shown="Disabled" {
    frame Disabled {
      # "GetMotorPositions"
      # "get all motor positions"
      n952 = call <userlib>:"Tick Count (ms)__ogtk.vi"() -> ("millisecond timer value"=w2024:u32)  [unwired: 10 in, 1 out]
      n953 = Unbundle By Name(w2025) -> ("dev var alias arrays"=w2017)
      n954 = Unbundle By Name(w2017) -> ("dev variable alias Motors X"=w2016, "dev variable alias Motors Y"=w2020)
      n955 = for {
        tunnel: w2020 -> [w2033]
        tunnel: w2016 -> [w2032]
        tunnel: [w2028] -> w2018 mode=indexing
        tunnel: [w2027] -> w2019 mode=indexing
        tunnel: w2020 -> [_]
        tunnel: [errorcluster {"status"=FALSE, "code"=0, "source"=""} ("error out")] -> w2021
        i -> [w2029]
        n956 = call "Beampointing get set motor position.vi"("Active CCD"=w2029, "get or set"=enum16{"get", "set"}."get", "dev variable alias Motors X"=w2032) -> ("Actual Position"=w2028:dbl)  [unwired: 7 in, 1 out]
        n957 = call "Beampointing get set motor position.vi"("Active CCD"=w2029, "get or set"=enum16{"get", "set"}."get", "dev variable alias Motors X"=w2033) -> ("Actual Position"=w2027:dbl)  [unwired: 7 in, 1 out]
      }
      n958 = Bundle By Name("Positions x"=w2018, "Positions y"=w2019) -> (w2025:cluster{})  [unwired: 1 out]
      n959 = call <userlib>:"Tick Count (ms)__ogtk.vi"("error in (no error)"=w2021) -> ("millisecond timer value"=w2022:u32)  [unwired: 9 in, 1 out]
      n960 = Subtract(x=w2022, y=w2024) -> (x-y=→"get pos time":u32)
    }
    frame Enabled {
    }
  }
  n961 = Unbundle By Name(w17) -> ("tdms ref"=w16:refnum<k34>)
  n962 = for {
    tunnel: w45 -> [w2036] mode=indexing
    tunnel: w44 -> [w2035]
    tunnel: [w2034] -> w15
    n963 = call "IMAQ Dispose"("Image"=w2036, "error in (no error)"=w2035) -> ("error out"=w2034:errorcluster)  [unwired: 4 in]
  }
  n964 = TDMS Close(8:w15, 11:w16) -> (0:→"error out 2":errorcluster)  [unwired: 1 out]
